vi "test_waypoint-files.vi"() -> ()   [LabVIEW 2019]
panel:
  in  "waypoint files cfg":T1={"Waypoint array"=[{"sel"=TRUE, "inv"=FALSE, "path"=path "C:/AGV/Log/0709/refwpt_0709-1 parking-lot to cafe.txt"}, {"sel"=TRUE, "inv"=TRUE, "path"=path "C:/AGV/Log/0709/refwpt_0709-3 hill to cafe.txt"}, {"sel"=TRUE, "inv"=FALSE, "path"=path "C:/AGV/Log/0709/refwpt_0709-3 hill to cafe.txt"}, {"sel"=TRUE, "inv"=TRUE, "path"=path "C:/AGV/Log/0709/refwpt_0709-1 parking-lot to cafe.txt"}]}
  in  "dt":u32
  out "curr":cluster{cluster{"X":dbl, "Y":dbl}[]}[](graph)
  in  "test run":bool
  in  "Finish":bool
  out "waypoint all":cluster{"XY 그래프":cluster{"X":dbl, "Y":dbl}[]}[](graph)=[{"XY 그래프"=[{"X"=175271.17619236137, "Y"=530128.4758223048}, {"X"=175271.19894111593, "Y"=530128.5113948234}, {"X"=175271.22097384508, "Y"=530128.5456653745}, {"X"=175271.24233997884, "Y"=530128.5782775495}, {"X"=175271.2630835386, "Y"=530128.6094398685}, {"X"=175271.28287635016, "Y"=530128.6390045825}, {"X"=175271.30246842964, "Y"=530128.6674888867}, {"X"=175271.32169791235, "Y"=530128.6949698408}, {"X"=175271.34079370368, "Y"=530128.7218740666}, {"X"=175271.35919639948, "Y"=530128.7486404965}, {"X"=175271.37760654237, "Y"=530128.7749307759}, {"X"=175271.3958476775, "Y"=530128.8006821633}, {"X"=175271.41409588268, "Y"=530128.82612943}, {"X"=175271.43256535105, "Y"=530128.8515127783}, {"X"=175271.45115096163, "Y"=530128.8775306249}, {"X"=175271.47020953769, "Y"=530128.9047301803}, {"X"=175271.48983988236, "Y"=530128.9335728578}, {"X"=175271.51075350813, "Y"=530128.9641342413}, {"X"=175271.5327281118, "Y"=530128.9964238653}, {"X"=175271.5556798252, "Y"=530129.0296384441}, {"X"=175271.57926803536, "Y"=530129.0639199342}, {"X"=175271.60322265813, "Y"=530129.0989961097}, {"X"=175271.62739598114, "Y"=530129.1343413345}, {"X"=175271.65204231316, "Y"=530129.1693854983}, {"X"=175271.67727888995, "Y"=530129.2039340293}, {"X"=175271.7021960715, "Y"=530129.2380118149}, {"X"=175271.7265418914, "Y"=530129.272080192}, {"X"=175271.75024861834, "Y"=530129.3060017383}, {"X"=175271.77407374466, "Y"=530129.3392237227}, {"X"=175271.79764021302, "Y"=530129.3715452666}, {"X"=175271.8208334585, "Y"=530129.4034650351}, {"X"=175271.84318632656, "Y"=530129.4351664272}, {"X"=175271.86533794703, "Y"=530129.4668095922}, {"X"=175271.88783310482, "Y"=530129.4987014595}, {"X"=175271.91096245, "Y"=530129.5317778906}, {"X"=175271.93534531837, "Y"=530129.5660936565}, {"X"=175271.96072388045, "Y"=530129.6019292073}, {"X"=175271.98658903624, "Y"=530129.6387610785}, {"X"=175272.01334256688, "Y"=530129.6755681273}, {"X"=175272.04048386813, "Y"=530129.7120055571}, {"X"=175272.06705517654, "Y"=530129.7482981697}, {"X"=175272.0929584909, "Y"=530129.7842564705}, {"X"=175272.1187534381, "Y"=530129.8198133239}, {"X"=175272.14471871415, "Y"=530129.8539590411}, {"X"=175272.16995301557, "Y"=530129.8877395594}, {"X"=175272.19405677487, "Y"=530129.9217287443}, {"X"=175272.21833020137, "Y"=530129.9549815882}, {"X"=175272.24264042586, "Y"=530129.9874995985}, {"X"=175272.26682258598, "Y"=530130.019843742}, {"X"=175272.29097599763, "Y"=530130.0526518888}, {"X"=175272.3154578647, "Y"=530130.085699904}, {"X"=175272.3404045608, "Y"=530130.1189762856}, {"X"=175272.36576607375, "Y"=530130.1526421116}, {"X"=175272.39173061957, "Y"=530130.1868411056}, {"X"=175272.41826742142, "Y"=530130.2219496026}, {"X"=175272.44515761113, "Y"=530130.2582423848}, {"X"=175272.47299428293, "Y"=530130.2955867319}, {"X"=175272.50161956908, "Y"=530130.333617972}, {"X"=175272.53078700637, "Y"=530130.3725632413}, {"X"=175272.56009692047, "Y"=530130.4117622469}, {"X"=175272.58948861354, "Y"=530130.4507579056}, {"X"=175272.6189694897, "Y"=530130.4887599788}, {"X"=175272.64772876413, "Y"=530130.5265710694}, {"X"=175272.6754292347, "Y"=530130.564287625}, {"X"=175272.70290686525, "Y"=530130.6006341625}, {"X"=175272.73019329942, "Y"=530130.6358292324}, {"X"=175272.75748037494, "Y"=530130.6700431828}, {"X"=175272.78426411733, "Y"=530130.7035893793}, {"X"=175272.8101597084, "Y"=530130.736937318}, {"X"=175272.83573870684, "Y"=530130.7704626593}, {"X"=175272.8619184958, "Y"=530130.8040616941}, {"X"=175272.88838454854, "Y"=530130.8380128188}, {"X"=175272.9151794416, "Y"=530130.8723347735}, {"X"=175272.94225210417, "Y"=530130.9071309266}, {"X"=175272.9695424264, "Y"=530130.941844306}, {"X"=175272.99712724722, "Y"=530130.976398106}, {"X"=175273.02454639255, "Y"=530131.0115406199}, {"X"=175273.05220733272, "Y"=530131.0472728647}, {"X"=175273.0807986791, "Y"=530131.083413007}, {"X"=175273.11001776106, "Y"=530131.12035483}, {"X"=175273.13982529996, "Y"=530131.1576933515}, {"X"=175273.16959295332, "Y"=530131.1950231135}, {"X"=175273.199150427, "Y"=530131.2322702568}, {"X"=175273.22822233994, "Y"=530131.2691692308}, {"X"=175273.25699849764, "Y"=530131.3055019411}, {"X"=175273.28514402997, "Y"=530131.3418553857}, {"X"=175273.31300851193, "Y"=530131.3778234285}, {"X"=175273.34109626192, "Y"=530131.4126099229}, {"X"=175273.36875248022, "Y"=530131.4470458659}, {"X"=175273.39565498653, "Y"=530131.481215453}, {"X"=175273.42227395362, "Y"=530131.5150573613}, {"X"=175273.44885639485, "Y"=530131.5491280085}, {"X"=175273.47631335634, "Y"=530131.5835800796}, {"X"=175273.50455634613, "Y"=530131.6181441419}, {"X"=175273.53303207213, "Y"=530131.6526309372}, {"X"=175273.56118465195, "Y"=530131.6871741797}, {"X"=175273.5885399682, "Y"=530131.7217009136}, {"X"=175273.6153169799, "Y"=530131.7553703267}, {"X"=175273.64185773276, "Y"=530131.7882246927}, {"X"=175273.66779895552, "Y"=530131.8208311108}, {"X"=175273.69422745312, "Y"=530131.8528678423}, {"X"=175273.72143691947, "Y"=530131.8851020389}, {"X"=175273.74863117086, "Y"=530131.9187824245}, {"X"=175273.77588163048, "Y"=530131.9540952493}, {"X"=175273.80346250045, "Y"=530131.9897123085}, {"X"=175273.83148837282, "Y"=530132.0248430432}, {"X"=175273.85959956356, "Y"=530132.0594696489}, {"X"=175273.88716057636, "Y"=530132.0931644908}, {"X"=175273.91324101866, "Y"=530132.1258215536}, {"X"=175273.93725872994, "Y"=530132.1552794413}, {"X"=175273.9610060394, "Y"=530132.1840588958}, {"X"=175273.98491793906, "Y"=530132.2148788949}, {"X"=175274.01010218015, "Y"=530132.247312195}, {"X"=175274.0370394344, "Y"=530132.2812519423}, {"X"=175274.06522422977, "Y"=530132.3159082977}, {"X"=175274.09411559426, "Y"=530132.3504648948}, {"X"=175274.1227654554, "Y"=530132.3851287554}, {"X"=175274.1503264592, "Y"=530132.419419592}, {"X"=175274.17705452998, "Y"=530132.4530147897}, {"X"=175274.20284159074, "Y"=530132.4856116782}, {"X"=175274.2283037938, "Y"=530132.5170863498}, {"X"=175274.25342691143, "Y"=530132.547721861}, {"X"=175274.27838808816, "Y"=530132.5781114623}, {"X"=175274.3033260028, "Y"=530132.6090216575}, {"X"=175274.32839360525, "Y"=530132.6409536466}, {"X"=175274.35449309755, "Y"=530132.6734641539}, {"X"=175274.38062100383, "Y"=530132.7068968687}, {"X"=175274.40689989371, "Y"=530132.7407642006}, {"X"=175274.43333091473, "Y"=530132.7745556141}, {"X"=175274.4600217053, "Y"=530132.807526073}, {"X"=175274.4868586656, "Y"=530132.8399023252}, {"X"=175274.51285591608, "Y"=530132.87228661}, {"X"=175274.5382562742, "Y"=530132.9044162827}, {"X"=175274.5635473854, "Y"=530132.9355474041}, {"X"=175274.5884104021, "Y"=530132.9653934666}, {"X"=175274.61236441362, "Y"=530132.9945796295}, {"X"=175274.63632652618, "Y"=530133.0250077015}, {"X"=175274.66100385884, "Y"=530133.0573637048}, {"X"=175274.68682189335, "Y"=530133.0908495001}, {"X"=175274.71343456453, "Y"=530133.1246625733}, {"X"=175274.7394069741, "Y"=530133.1582322615}, {"X"=175274.76481200277, "Y"=530133.1910433752}, {"X"=175274.78956166538, "Y"=530133.2229962848}, {"X"=175274.8136799043, "Y"=530133.2538012478}, {"X"=175274.83683646756, "Y"=530133.2832084121}, {"X"=175274.85901448457, "Y"=530133.3115041718}, {"X"=175274.88039296027, "Y"=530133.3396114007}, {"X"=175274.90220277346, "Y"=530133.3680036975}, {"X"=175274.92494321318, "Y"=530133.3965796971}, {"X"=175274.94867800857, "Y"=530133.4259230008}, {"X"=175274.97288089248, "Y"=530133.4562959785}, {"X"=175274.99738909313, "Y"=530133.4874727023}, {"X"=175275.02195266922, "Y"=530133.5191031941}, {"X"=175275.04693453235, "Y"=530133.5507990399}, {"X"=175275.07211187517, "Y"=530133.582399972}, {"X"=175275.0973483225, "Y"=530133.6136189348}, {"X"=175275.12214456138, "Y"=530133.6445484182}, {"X"=175275.1461691421, "Y"=530133.6748353543}, {"X"=175275.16997141903, "Y"=530133.7045325036}, {"X"=175275.19344551215, "Y"=530133.7334825781}, {"X"=175275.21657627032, "Y"=530133.7622516518}, {"X"=175275.2396087607, "Y"=530133.791039883}, {"X"=175275.263063832, "Y"=530133.8204461659}, {"X"=175275.28697082214, "Y"=530133.8502073783}, {"X"=175275.3107248371, "Y"=530133.8806593737}, {"X"=175275.33444671123, "Y"=530133.9113245594}, {"X"=175275.35827569605, "Y"=530133.9419672296}, {"X"=175275.38238149675, "Y"=530133.9721618079}, {"X"=175275.40583026237, "Y"=530134.0021319196}, {"X"=175275.42878089705, "Y"=530134.0313976321}, {"X"=175275.451392896, "Y"=530134.0596743522}, {"X"=175275.4738905455, "Y"=530134.0867261271}, {"X"=175275.49585796281, "Y"=530134.113300008}, {"X"=175275.5176917569, "Y"=530134.1402172334}, {"X"=175275.53996690773, "Y"=530134.1678123861}, {"X"=175275.5632661976, "Y"=530134.1963612096}, {"X"=175275.58703968537, "Y"=530134.2259097229}, {"X"=175275.6113424378, "Y"=530134.2565077101}, {"X"=175275.63557628682, "Y"=530134.2880681476}, {"X"=175275.66020323776, "Y"=530134.3195641611}, {"X"=175275.68491628268, "Y"=530134.35081908}, {"X"=175275.7097711018, "Y"=530134.3817905674}, {"X"=175275.73389469017, "Y"=530134.4126088354}, {"X"=175275.7577146616, "Y"=530134.4423003837}, {"X"=175275.78100623479, "Y"=530134.4715351238}, {"X"=175275.80342291066, "Y"=530134.5005604674}, {"X"=175275.82593068006, "Y"=530134.5292381555}, {"X"=175275.84870407218, "Y"=530134.557576552}, {"X"=175275.8723047294, "Y"=530134.5861932964}, {"X"=175275.8962104465, "Y"=530134.6158257698}, {"X"=175275.9206685924, "Y"=530134.6465531515}, {"X"=175275.94534715984, "Y"=530134.6778314793}, {"X"=175275.97041945267, "Y"=530134.7092562574}, {"X"=175275.99540918533, "Y"=530134.7409198968}, {"X"=175276.0208479327, "Y"=530134.7722559111}, {"X"=175276.04626527152, "Y"=530134.8032423825}, {"X"=175276.0707201348, "Y"=530134.8340574529}, {"X"=175276.09469571977, "Y"=530134.8642524196}, {"X"=175276.11845871908, "Y"=530134.8938497994}, {"X"=175276.14216767476, "Y"=530134.9231443482}, {"X"=175276.16565515427, "Y"=530134.9527281164}, {"X"=175276.18933507518, "Y"=530134.9829883279}, {"X"=175276.21328929672, "Y"=530135.0137471656}, {"X"=175276.23786405282, "Y"=530135.0443687653}, {"X"=175276.26216325478, "Y"=530135.07556498}, {"X"=175276.28639760052, "Y"=530135.1066959022}, {"X"=175276.3104839446, "Y"=530135.1375020731}, {"X"=175276.33440064892, "Y"=530135.1675562614}, {"X"=175276.35738667226, "Y"=530135.1965088919}, {"X"=175276.37903969965, "Y"=530135.2246053237}, {"X"=175276.40010305776, "Y"=530135.2524926253}, {"X"=175276.42257118158, "Y"=530135.2821426697}, {"X"=175276.44697916886, "Y"=530135.3138823927}, {"X"=175276.47269765826, "Y"=530135.3469600595}, {"X"=175276.4987057177, "Y"=530135.3812077725}, {"X"=175276.52459011346, "Y"=530135.415572385}, {"X"=175276.54989015873, "Y"=530135.449730072}, {"X"=175276.57483091034, "Y"=530135.4828044904}, {"X"=175276.59904920924, "Y"=530135.5148000421}, {"X"=175276.62270533358, "Y"=530135.5457007147}, {"X"=175276.64582765175, "Y"=530135.5755130845}, {"X"=175276.66823122185, "Y"=530135.6040024065}, {"X"=175276.68969509072, "Y"=530135.6316354779}, {"X"=175276.71066645414, "Y"=530135.6586684603}, {"X"=175276.73236713343, "Y"=530135.6861043859}, {"X"=175276.75435481517, "Y"=530135.7147414407}, {"X"=175276.7766906527, "Y"=530135.7445894321}, {"X"=175276.79958941144, "Y"=530135.7757864564}, {"X"=175276.82353418818, "Y"=530135.8078460784}, {"X"=175276.8479998637, "Y"=530135.8408220143}, {"X"=175276.87281893456, "Y"=530135.874385132}, {"X"=175276.8982353833, "Y"=530135.9077689041}, {"X"=175276.92355676193, "Y"=530135.941353842}, {"X"=175276.94920471654, "Y"=530135.9748434767}, {"X"=175276.97503856523, "Y"=530136.0085911597}, {"X"=175277.00103956382, "Y"=530136.042549222}, {"X"=175277.0271864251, "Y"=530136.0773070601}, {"X"=175277.0538277369, "Y"=530136.1127238036}, {"X"=175277.08122741545, "Y"=530136.1490827955}, {"X"=175277.1097199428, "Y"=530136.1859668468}, {"X"=175277.13826682538, "Y"=530136.2235588295}, {"X"=175277.16623464657, "Y"=530136.2618339786}, {"X"=175277.19366071408, "Y"=530136.3005269243}, {"X"=175277.2211805134, "Y"=530136.3385669983}, {"X"=175277.24894896135, "Y"=530136.3759193327}, {"X"=175277.27651148668, "Y"=530136.4128305535}, {"X"=175277.30377007398, "Y"=530136.4488059506}, {"X"=175277.3310530873, "Y"=530136.4837557664}, {"X"=175277.35790209068, "Y"=530136.5187157434}, {"X"=175277.38489518996, "Y"=530136.5535776294}, {"X"=175277.41163428145, "Y"=530136.5885124052}, {"X"=175277.43827130183, "Y"=530136.6233775625}, {"X"=175277.4651897453, "Y"=530136.6581553189}, {"X"=175277.49179216905, "Y"=530136.6927042685}, {"X"=175277.5176344978, "Y"=530136.727524051}, {"X"=175277.54344339736, "Y"=530136.7624216232}, {"X"=175277.56908157616, "Y"=530136.7971010571}, {"X"=175277.59486848288, "Y"=530136.8314515362}, {"X"=175277.62049959434, "Y"=530136.8667358635}, {"X"=175277.6472220221, "Y"=530136.9020269552}, {"X"=175277.6753270872, "Y"=530136.9375892024}, {"X"=175277.70423989603, "Y"=530136.9740158635}, {"X"=175277.73315492744, "Y"=530137.0114946631}, {"X"=175277.762207521, "Y"=530137.0490629561}, {"X"=175277.79086273597, "Y"=530137.08704529}, {"X"=175277.81920082003, "Y"=530137.1247233516}, {"X"=175277.84718645428, "Y"=530137.1618353155}, {"X"=175277.87464469287, "Y"=530137.1979299895}, {"X"=175277.9008237915, "Y"=530137.2337065866}, {"X"=175277.9271261955, "Y"=530137.2689456482}, {"X"=175277.95360932988, "Y"=530137.3044938259}, {"X"=175277.98064951657, "Y"=530137.3403033918}, {"X"=175278.00823913375, "Y"=530137.376793897}, {"X"=175278.03589400547, "Y"=530137.4140821989}, {"X"=175278.06381256797, "Y"=530137.4518780371}, {"X"=175278.0928952896, "Y"=530137.4894506804}, {"X"=175278.12228673112, "Y"=530137.5271800106}, {"X"=175278.151430175, "Y"=530137.5652175064}, {"X"=175278.180067244, "Y"=530137.6036560485}, {"X"=175278.2089476153, "Y"=530137.6413968799}, {"X"=175278.23784769257, "Y"=530137.67891235}, {"X"=175278.26667870057, "Y"=530137.7167343476}, {"X"=175278.295506967, "Y"=530137.7548282683}, {"X"=175278.3247139495, "Y"=530137.7924860048}, {"X"=175278.35371856295, "Y"=530137.8306049308}, {"X"=175278.38247794105, "Y"=530137.8690675278}, {"X"=175278.41117485458, "Y"=530137.9076745918}, {"X"=175278.43986590861, "Y"=530137.9460974373}, {"X"=175278.46847093437, "Y"=530137.9841853591}, {"X"=175278.49675173132, "Y"=530138.0219634802}, {"X"=175278.52471101953, "Y"=530138.0600522002}, {"X"=175278.55337122487, "Y"=530138.097927977}, {"X"=175278.58284640842, "Y"=530138.1352219965}, {"X"=175278.61280407023, "Y"=530138.1730195764}, {"X"=175278.6421407967, "Y"=530138.212318413}, {"X"=175278.6718176569, "Y"=530138.2519125747}, {"X"=175278.70174630472, "Y"=530138.2918822337}, {"X"=175278.7324047895, "Y"=530138.33213164}, {"X"=175278.76330645662, "Y"=530138.3722427061}, {"X"=175278.7947664709, "Y"=530138.4115552426}, {"X"=175278.82585993598, "Y"=530138.4509254653}, {"X"=175278.85671998298, "Y"=530138.4901432156}, {"X"=175278.88660487908, "Y"=530138.5296956997}, {"X"=175278.91639916634, "Y"=530138.5691607723}, {"X"=175278.9459413744, "Y"=530138.6081526802}, {"X"=175278.97519875658, "Y"=530138.6466803991}, {"X"=175279.00399939533, "Y"=530138.6850196817}, {"X"=175279.0333091102, "Y"=530138.7223730155}, {"X"=175279.06206272755, "Y"=530138.760087587}, {"X"=175279.09082204034, "Y"=530138.7988298717}, {"X"=175279.12034452776, "Y"=530138.8386420244}, {"X"=175279.1511945661, "Y"=530138.8792682199}, {"X"=175279.18281582693, "Y"=530138.9203915691}, {"X"=175279.21403033624, "Y"=530138.9614550801}, {"X"=175279.2443611752, "Y"=530139.0023391879}, {"X"=175279.27433731925, "Y"=530139.0421966133}, {"X"=175279.30379101905, "Y"=530139.0806149871}, {"X"=175279.33186221574, "Y"=530139.1185080461}, {"X"=175279.35892676964, "Y"=530139.1559723445}, {"X"=175279.38686212158, "Y"=530139.1922598379}, {"X"=175279.41540915347, "Y"=530139.2284112311}, {"X"=175279.44399877635, "Y"=530139.2654858995}, {"X"=175279.47229163084, "Y"=530139.3037501057}, {"X"=175279.5011885739, "Y"=530139.3417073153}, {"X"=175279.5302888436, "Y"=530139.3795274108}, {"X"=175279.55929689365, "Y"=530139.4170148209}, {"X"=175279.58712148367, "Y"=530139.4547876343}, {"X"=175279.614104584, "Y"=530139.4922666025}, {"X"=175279.64106285188, "Y"=530139.5288355612}, {"X"=175279.66805218573, "Y"=530139.5639283156}, {"X"=175279.69406272576, "Y"=530139.5987243007}, {"X"=175279.72019882765, "Y"=530139.6337452154}, {"X"=175279.7465857226, "Y"=530139.6700028821}, {"X"=175279.77402264145, "Y"=530139.7072807357}, {"X"=175279.8023412458, "Y"=530139.7461663891}, {"X"=175279.83184920144, "Y"=530139.7864591549}, {"X"=175279.86223487387, "Y"=530139.8276150165}, {"X"=175279.89343681408, "Y"=530139.8689249574}, {"X"=175279.9246664868, "Y"=530139.910027272}, {"X"=175279.95597331063, "Y"=530139.9508596614}, {"X"=175279.98646708307, "Y"=530139.9914291999}, {"X"=175280.0165342933, "Y"=530140.0312308655}, {"X"=175280.0455922527, "Y"=530140.0703207663}, {"X"=175280.07421584064, "Y"=530140.1081000975}, {"X"=175280.10217132277, "Y"=530140.1449069497}, {"X"=175280.1291443291, "Y"=530140.1810696573}, {"X"=175280.15513247682, "Y"=530140.2166825664}, {"X"=175280.18117865722, "Y"=530140.2509501547}, {"X"=175280.206797209, "Y"=530140.2840913909}, {"X"=175280.23235000763, "Y"=530140.3165635753}, {"X"=175280.25719254743, "Y"=530140.350583895}, {"X"=175280.28322486824, "Y"=530140.3861567193}, {"X"=175280.31067604403, "Y"=530140.4234656083}, {"X"=175280.3394714572, "Y"=530140.4627371931}, {"X"=175280.36899300263, "Y"=530140.5034339112}, {"X"=175280.3984291721, "Y"=530140.5446147801}, {"X"=175280.42762195613, "Y"=530140.5855666273}, {"X"=175280.45709143404, "Y"=530140.6248306718}, {"X"=175280.48662985, "Y"=530140.6622443764}, {"X"=175280.51499879934, "Y"=530140.6989856332}, {"X"=175280.54198175855, "Y"=530140.7349207922}, {"X"=175280.56821058405, "Y"=530140.7692488853}, {"X"=175280.5935160324, "Y"=530140.8028483094}, {"X"=175280.61895653373, "Y"=530140.8353896387}, {"X"=175280.64395685605, "Y"=530140.8685493513}, {"X"=175280.66892636206, "Y"=530140.9029710654}, {"X"=175280.69431101237, "Y"=530140.9384925328}, {"X"=175280.72115648974, "Y"=530140.9743659461}, {"X"=175280.74851024564, "Y"=530141.0107827985}, {"X"=175280.77549811464, "Y"=530141.0483794013}, {"X"=175280.80221979975, "Y"=530141.0867248375}, {"X"=175280.83002676512, "Y"=530141.1242324503}, {"X"=175280.85869850015, "Y"=530141.1612214238}, {"X"=175280.88737895148, "Y"=530141.1984623082}, {"X"=175280.9154864763, "Y"=530141.2366638052}, {"X"=175280.94386501168, "Y"=530141.2751508438}, {"X"=175280.97276275096, "Y"=530141.3139804051}, {"X"=175281.00228102322, "Y"=530141.3529734996}, {"X"=175281.03115592728, "Y"=530141.3927687078}, {"X"=175281.0600630094, "Y"=530141.4329611481}, {"X"=175281.08951047983, "Y"=530141.4728734163}, {"X"=175281.1195389884, "Y"=530141.5124709872}, {"X"=175281.1496177038, "Y"=530141.5525733957}, {"X"=175281.1799730451, "Y"=530141.5930623271}, {"X"=175281.20985549872, "Y"=530141.6341930445}, {"X"=175281.24002660922, "Y"=530141.6758856092}, {"X"=175281.2701406386, "Y"=530141.7180455929}, {"X"=175281.30071187392, "Y"=530141.7596526246}, {"X"=175281.3314443854, "Y"=530141.8009806047}, {"X"=175281.36215111212, "Y"=530141.8419768134}, {"X"=175281.39229160105, "Y"=530141.8831999974}, {"X"=175281.42191398598, "Y"=530141.9244513493}, {"X"=175281.4515510467, "Y"=530141.9652731441}, {"X"=175281.48146043535, "Y"=530142.005928764}, {"X"=175281.51131504713, "Y"=530142.0472304844}, {"X"=175281.54193657986, "Y"=530142.088173672}, {"X"=175281.57268864528, "Y"=530142.1289266894}, {"X"=175281.60313783126, "Y"=530142.1699991305}, {"X"=175281.63309546496, "Y"=530142.2110941121}, {"X"=175281.66344358743, "Y"=530142.2512401207}, {"X"=175281.6938036245, "Y"=530142.2909221732}, {"X"=175281.7242871103, "Y"=530142.3298147498}, {"X"=175281.75410497762, "Y"=530142.3688757736}, {"X"=175281.78380300084, "Y"=530142.4081480255}, {"X"=175281.8133516878, "Y"=530142.4481421259}, {"X"=175281.843129746, "Y"=530142.4887193365}, {"X"=175281.87290404478, "Y"=530142.530421954}, {"X"=175281.9035498242, "Y"=530142.5720776024}, {"X"=175281.93428441955, "Y"=530142.6138128963}, {"X"=175281.96503678558, "Y"=530142.6558666679}, {"X"=175281.9955543286, "Y"=530142.697891169}, {"X"=175282.02619666213, "Y"=530142.7392804611}, {"X"=175282.05613426614, "Y"=530142.7804920393}, {"X"=175282.085671532, "Y"=530142.8211187952}, {"X"=175282.11518036062, "Y"=530142.8620131105}, {"X"=175282.1456811949, "Y"=530142.9028811874}, {"X"=175282.1771792938, "Y"=530142.9437019224}, {"X"=175282.20884129676, "Y"=530142.9851325951}, {"X"=175282.2397414916, "Y"=530143.0274545162}, {"X"=175282.27097983484, "Y"=530143.0694003062}, {"X"=175282.30222752306, "Y"=530143.1112106664}, {"X"=175282.33341880344, "Y"=530143.1525184269}, {"X"=175282.36387121098, "Y"=530143.1931857627}, {"X"=175282.39415697358, "Y"=530143.2332143132}, {"X"=175282.42362074467, "Y"=530143.273250842}, {"X"=175282.4527898988, "Y"=530143.313107335}, {"X"=175282.48128543983, "Y"=530143.3534241924}, {"X"=175282.51088211057, "Y"=530143.3931717661}, {"X"=175282.54090583324, "Y"=530143.4323542686}, {"X"=175282.5705854428, "Y"=530143.471693168}, {"X"=175282.59956877265, "Y"=530143.5110152598}, {"X"=175282.6287490361, "Y"=530143.5495365605}, {"X"=175282.6578151003, "Y"=530143.588080396}, {"X"=175282.68706937856, "Y"=530143.626769067}, {"X"=175282.7166015784, "Y"=530143.6659829883}, {"X"=175282.7467854581, "Y"=530143.7057077412}, {"X"=175282.7773134472, "Y"=530143.7458743079}, {"X"=175282.80814411398, "Y"=530143.7859523029}, {"X"=175282.838184342, "Y"=530143.826524301}, {"X"=175282.8683331907, "Y"=530143.8669838827}, {"X"=175282.89893667438, "Y"=530143.906620824}, {"X"=175282.9292553414, "Y"=530143.9460954601}, {"X"=175282.95864972533, "Y"=530143.9860345288}, {"X"=175282.98848236992, "Y"=530144.0253041666}, {"X"=175283.0181754902, "Y"=530144.0647196089}, {"X"=175283.04813967334, "Y"=530144.1041386905}, {"X"=175283.0777535639, "Y"=530144.1434200734}, {"X"=175283.10767498845, "Y"=530144.1824585982}, {"X"=175283.13729311575, "Y"=530144.2216767089}, {"X"=175283.16682575422, "Y"=530144.2604411386}, {"X"=175283.19558793583, "Y"=530144.298968117}, {"X"=175283.2241672666, "Y"=530144.3373668897}, {"X"=175283.25312463212, "Y"=530144.3756990653}, {"X"=175283.2826412646, "Y"=530144.4144435665}, {"X"=175283.31204253566, "Y"=530144.4543149145}, {"X"=175283.3421730828, "Y"=530144.4945792174}, {"X"=175283.3722977522, "Y"=530144.5352508556}, {"X"=175283.40277253534, "Y"=530144.5759991499}, {"X"=175283.4329718328, "Y"=530144.6164463753}, {"X"=175283.46352714679, "Y"=530144.6565706909}, {"X"=175283.49419215746, "Y"=530144.6963472951}, {"X"=175283.52462383907, "Y"=530144.7353998523}, {"X"=175283.55396090678, "Y"=530144.7748296679}, {"X"=175283.5835840078, "Y"=530144.8145316618}, {"X"=175283.61356165347, "Y"=530144.8549118419}, {"X"=175283.64420085354, "Y"=530144.8958449971}, {"X"=175283.6745753304, "Y"=530144.9374226541}, {"X"=175283.7054805737, "Y"=530144.9784593498}, {"X"=175283.73611770716, "Y"=530145.0195933951}, {"X"=175283.76646929348, "Y"=530145.060618409}, {"X"=175283.79638575143, "Y"=530145.1009754644}, {"X"=175283.82613484285, "Y"=530145.1407492278}, {"X"=175283.85577592644, "Y"=530145.1808429519}, {"X"=175283.885663239, "Y"=530145.2218282747}, {"X"=175283.91601352586, "Y"=530145.2642128682}, {"X"=175283.947973915, "Y"=530145.3071054613}, {"X"=175283.98073738883, "Y"=530145.3501865757}, {"X"=175284.0130592979, "Y"=530145.3937184858}, {"X"=175284.04495574543, "Y"=530145.4371550977}, {"X"=175284.07744431793, "Y"=530145.4792348221}, {"X"=175284.10977979988, "Y"=530145.5207656174}, {"X"=175284.14209092426, "Y"=530145.5618481026}, {"X"=175284.1734844176, "Y"=530145.6035470525}, {"X"=175284.20526964756, "Y"=530145.64591853}, {"X"=175284.23726074316, "Y"=530145.6887122538}, {"X"=175284.26911709429, "Y"=530145.7317705223}, {"X"=175284.3002081578, "Y"=530145.7757400281}, {"X"=175284.3324970653, "Y"=530145.8188969061}, {"X"=175284.3652071701, "Y"=530145.861604157}, {"X"=175284.39764851984, "Y"=530145.9041912265}, {"X"=175284.42918119673, "Y"=530145.9465290459}, {"X"=175284.46056710478, "Y"=530145.9883589816}, {"X"=175284.49216892465, "Y"=530146.0298153689}, {"X"=175284.52417019266, "Y"=530146.0712561457}, {"X"=175284.55620185586, "Y"=530146.1139909273}, {"X"=175284.58914297097, "Y"=530146.1578373206}, {"X"=175284.62234006467, "Y"=530146.2022778434}, {"X"=175284.65546114062, "Y"=530146.246771863}, {"X"=175284.6880941868, "Y"=530146.290381658}, {"X"=175284.7208188328, "Y"=530146.3323175148}, {"X"=175284.75239886277, "Y"=530146.3738938312}, {"X"=175284.7831501817, "Y"=530146.4147045729}, {"X"=175284.8133402377, "Y"=530146.4547267567}, {"X"=175284.84401715046, "Y"=530146.4940394099}, {"X"=175284.87397091367, "Y"=530146.5335351082}, {"X"=175284.9036312302, "Y"=530146.5732458769}, {"X"=175284.93309855444, "Y"=530146.613594275}, {"X"=175284.96356257205, "Y"=530146.6534025557}, {"X"=175284.99386236374, "Y"=530146.6933911182}, {"X"=175285.02346019607, "Y"=530146.7338401279}, {"X"=175285.05236272336, "Y"=530146.7740026298}, {"X"=175285.08160787256, "Y"=530146.8135059732}, {"X"=175285.11075855847, "Y"=530146.8522171556}, {"X"=175285.1397029091, "Y"=530146.8900477202}, {"X"=175285.16758823174, "Y"=530146.9277071673}, {"X"=175285.1958097519, "Y"=530146.9649305547}, {"X"=175285.22430324028, "Y"=530147.0021642376}, {"X"=175285.25292049572, "Y"=530147.0399147498}, {"X"=175285.2813211958, "Y"=530147.0781209449}, {"X"=175285.31057523662, "Y"=530147.1161381598}, {"X"=175285.34005196817, "Y"=530147.1539760306}, {"X"=175285.36896240644, "Y"=530147.1923216721}, {"X"=175285.39717128137, "Y"=530147.2306616167}, {"X"=175285.42578933577, "Y"=530147.2680836085}, {"X"=175285.45344861108, "Y"=530147.3059856722}, {"X"=175285.48089067373, "Y"=530147.3438228995}, {"X"=175285.5080579749, "Y"=530147.3816032234}, {"X"=175285.5362745623, "Y"=530147.4192572538}, {"X"=175285.56450088962, "Y"=530147.457507248}, {"X"=175285.59262162892, "Y"=530147.4962980582}, {"X"=175285.62062185156, "Y"=530147.535671899}, {"X"=175285.64955586256, "Y"=530147.5747999209}, {"X"=175285.67873101955, "Y"=530147.6137008192}, {"X"=175285.70778441665, "Y"=530147.6521647931}, {"X"=175285.73595734, "Y"=530147.6906291493}, {"X"=175285.76424656826, "Y"=530147.7282851851}, {"X"=175285.79254815428, "Y"=530147.7653274323}, {"X"=175285.82039661068, "Y"=530147.8022034307}, {"X"=175285.8475120278, "Y"=530147.8389140045}, {"X"=175285.87503700587, "Y"=530147.8754358034}, {"X"=175285.90290258938, "Y"=530147.9124127475}, {"X"=175285.9312492372, "Y"=530147.9503150036}, {"X"=175285.96021217544, "Y"=530147.9893430532}, {"X"=175285.99025259638, "Y"=530148.0293912095}, {"X"=175286.020547502, "Y"=530148.0707260491}, {"X"=175286.0507198295, "Y"=530148.1125473701}, {"X"=175286.0801991385, "Y"=530148.1548557479}, {"X"=175286.11029842027, "Y"=530148.1962377818}, {"X"=175286.140521968, "Y"=530148.236507368}, {"X"=175286.1702336265, "Y"=530148.2765109926}, {"X"=175286.19897639108, "Y"=530148.3165685348}, {"X"=175286.22822459688, "Y"=530148.3559109423}, {"X"=175286.25734444545, "Y"=530148.3955811377}, {"X"=175286.28666392548, "Y"=530148.4356613915}, {"X"=175286.31565993704, "Y"=530148.4762897632}, {"X"=175286.3452906467, "Y"=530148.5167775253}, {"X"=175286.37519197192, "Y"=530148.5571168768}, {"X"=175286.4050008174, "Y"=530148.5970369751}, {"X"=175286.43396749627, "Y"=530148.6376310271}, {"X"=175286.46322490054, "Y"=530148.6782874814}, {"X"=175286.492849835, "Y"=530148.7186198815}, {"X"=175286.52249772992, "Y"=530148.7589289073}, {"X"=175286.55175465223, "Y"=530148.7991236621}, {"X"=175286.58125565466, "Y"=530148.8385840784}, {"X"=175286.61029576242, "Y"=530148.8779481912}, {"X"=175286.63886234077, "Y"=530148.9171383454}, {"X"=175286.6662366717, "Y"=530148.9560379102}, {"X"=175286.69313776202, "Y"=530148.994561523}, {"X"=175286.71988594692, "Y"=530149.0322998049}, {"X"=175286.74621013305, "Y"=530149.0686387003}, {"X"=175286.77196082624, "Y"=530149.105147988}, {"X"=175286.79863885418, "Y"=530149.142826546}, {"X"=175286.826449198, "Y"=530149.1826948401}, {"X"=175286.85571812605, "Y"=530149.22455435}, {"X"=175286.8856057402, "Y"=530149.2680490734}, {"X"=175286.9166891728, "Y"=530149.3112439304}, {"X"=175286.94756222956, "Y"=530149.3539899159}, {"X"=175286.97788231372, "Y"=530149.3960549736}, {"X"=175287.0072642036, "Y"=530149.4374746449}, {"X"=175287.036659181, "Y"=530149.4776268187}, {"X"=175287.06515292102, "Y"=530149.5170491512}, {"X"=175287.09290277224, "Y"=530149.5556312968}, {"X"=175287.119605925, "Y"=530149.5949179686}, {"X"=175287.14739103278, "Y"=530149.6343412843}, {"X"=175287.17584614863, "Y"=530149.6735817129}, {"X"=175287.2043462658, "Y"=530149.713065068}, {"X"=175287.23238548372, "Y"=530149.7533488837}, {"X"=175287.2611683341, "Y"=530149.7940866544}, {"X"=175287.29022015305, "Y"=530149.8350178539}, {"X"=175287.31949523537, "Y"=530149.8762647061}, {"X"=175287.3483993774, "Y"=530149.9178800166}, {"X"=175287.37800341408, "Y"=530149.9598373151}, {"X"=175287.40788540026, "Y"=530150.0026284064}, {"X"=175287.43796715222, "Y"=530150.0458750587}, {"X"=175287.46768028973, "Y"=530150.0890806267}, {"X"=175287.4980408877, "Y"=530150.131969081}, {"X"=175287.52849568735, "Y"=530150.1743611491}, {"X"=175287.55858161338, "Y"=530150.2166244559}, {"X"=175287.587891292, "Y"=530150.2584882879}, {"X"=175287.61718485222, "Y"=530150.299393249}, {"X"=175287.6459290996, "Y"=530150.3402576577}, {"X"=175287.6745216954, "Y"=530150.3816607958}, {"X"=175287.70312189191, "Y"=530150.4232381617}, {"X"=175287.73260160128, "Y"=530150.4650881741}, {"X"=175287.76249647667, "Y"=530150.5074463824}, {"X"=175287.79194968793, "Y"=530150.5502209846}, {"X"=175287.82063771554, "Y"=530150.5936437859}, {"X"=175287.85010417973, "Y"=530150.6364072509}, {"X"=175287.8799999824, "Y"=530150.6784802239}, {"X"=175287.90960605638, "Y"=530150.7208281889}, {"X"=175287.93873272298, "Y"=530150.7643085173}, {"X"=175287.96876992864, "Y"=530150.8083710499}, {"X"=175287.99941347007, "Y"=530150.8537847098}, {"X"=175288.03114061506, "Y"=530150.8995947163}, {"X"=175288.06276278125, "Y"=530150.9458489771}, {"X"=175288.09491236706, "Y"=530150.9922304217}, {"X"=175288.12711197292, "Y"=530151.0378525751}, {"X"=175288.15885105054, "Y"=530151.0829045124}, {"X"=175288.18957201828, "Y"=530151.1275432631}, {"X"=175288.22029953293, "Y"=530151.1716992052}, {"X"=175288.25093068994, "Y"=530151.2162216855}, {"X"=175288.28194385857, "Y"=530151.2608229464}, {"X"=175288.31247756336, "Y"=530151.3053401643}, {"X"=175288.3432649797, "Y"=530151.3499842685}, {"X"=175288.37381855643, "Y"=530151.3946312824}, {"X"=175288.40417486875, "Y"=530151.4390691165}, {"X"=175288.43387214167, "Y"=530151.4838041204}, {"X"=175288.4640216559, "Y"=530151.5281038334}, {"X"=175288.49419391077, "Y"=530151.5723058113}, {"X"=175288.52442907562, "Y"=530151.6168139238}, {"X"=175288.5542325439, "Y"=530151.6615153196}, {"X"=175288.58497125428, "Y"=530151.7061640078}, {"X"=175288.6160333851, "Y"=530151.7508494728}, {"X"=175288.6471765447, "Y"=530151.7953782111}, {"X"=175288.67735389853, "Y"=530151.8404070201}, {"X"=175288.7079524178, "Y"=530151.8849762128}, {"X"=175288.73890247892, "Y"=530151.928907307}, {"X"=175288.76994925848, "Y"=530151.9731943812}, {"X"=175288.80061505685, "Y"=530152.0180497186}, {"X"=175288.8317122577, "Y"=530152.0632134323}, {"X"=175288.86321392213, "Y"=530152.1088598475}, {"X"=175288.89513094307, "Y"=530152.1541798481}, {"X"=175288.92626476596, "Y"=530152.1997463321}, {"X"=175288.95799837503, "Y"=530152.2447483455}, {"X"=175288.98898292525, "Y"=530152.2889612439}, {"X"=175289.01901433212, "Y"=530152.3328628676}, {"X"=175289.04869555627, "Y"=530152.376364868}, {"X"=175289.07902414582, "Y"=530152.419217908}, {"X"=175289.10912839917, "Y"=530152.4628917961}, {"X"=175289.13898367598, "Y"=530152.50744099}, {"X"=175289.16920329822, "Y"=530152.5520878835}, {"X"=175289.200499284, "Y"=530152.5967771014}, {"X"=175289.23222510127, "Y"=530152.6409434144}, {"X"=175289.26360565764, "Y"=530152.6851751207}, {"X"=175289.29417483156, "Y"=530152.7294092241}, {"X"=175289.32498934455, "Y"=530152.7727347375}, {"X"=175289.35533826269, "Y"=530152.8164722754}, {"X"=175289.385890799, "Y"=530152.8604711375}, {"X"=175289.41661120942, "Y"=530152.904625996}, {"X"=175289.4478910891, "Y"=530152.9495616502}, {"X"=175289.47917020373, "Y"=530152.9951376967}, {"X"=175289.5106185431, "Y"=530153.0407265619}, {"X"=175289.54200313758, "Y"=530153.08602594}, {"X"=175289.5739645148, "Y"=530153.130472353}, {"X"=175289.60522496788, "Y"=530153.1748287205}, {"X"=175289.6366590831, "Y"=530153.2192023303}, {"X"=175289.6678968938, "Y"=530153.2639904988}, {"X"=175289.69931618578, "Y"=530153.3099423731}, {"X"=175289.73108270628, "Y"=530153.3561928844}, {"X"=175289.76287250203, "Y"=530153.402526566}, {"X"=175289.7944634813, "Y"=530153.4493247548}, {"X"=175289.82722049116, "Y"=530153.4953348278}, {"X"=175289.8601326513, "Y"=530153.5407928433}, {"X"=175289.89234136775, "Y"=530153.5862074348}, {"X"=175289.9231350958, "Y"=530153.6320945667}, {"X"=175289.95472487184, "Y"=530153.6784854437}, {"X"=175289.98763897427, "Y"=530153.7249001521}, {"X"=175290.0213877559, "Y"=530153.7711048503}, {"X"=175290.05441688612, "Y"=530153.8180774795}, {"X"=175290.0870279125, "Y"=530153.865045794}, {"X"=175290.1190894426, "Y"=530153.9119114052}, {"X"=175290.15082290868, "Y"=530153.9583695601}, {"X"=175290.18253651966, "Y"=530154.004402696}, {"X"=175290.215824471, "Y"=530154.0499339624}, {"X"=175290.24876343764, "Y"=530154.0957714727}, {"X"=175290.28090772417, "Y"=530154.1421662602}, {"X"=175290.31260737777, "Y"=530154.1888720124}, {"X"=175290.34510314872, "Y"=530154.2349083878}, {"X"=175290.37745346018, "Y"=530154.2805800489}, {"X"=175290.40967781737, "Y"=530154.3255950455}, {"X"=175290.4415173953, "Y"=530154.3698930992}, {"X"=175290.47334424395, "Y"=530154.4146795312}, {"X"=175290.50540644318, "Y"=530154.4602743543}, {"X"=175290.5380738031, "Y"=530154.5068251977}, {"X"=175290.57155401353, "Y"=530154.5544701797}, {"X"=175290.60687618723, "Y"=530154.6022528902}, {"X"=175290.64227715097, "Y"=530154.6503194917}, {"X"=175290.6771000642, "Y"=530154.6985121064}, {"X"=175290.71074572636, "Y"=530154.7463930005}, {"X"=175290.74366782108, "Y"=530154.7937166628}, {"X"=175290.77674741115, "Y"=530154.8397823889}, {"X"=175290.8104922183, "Y"=530154.8852446075}, {"X"=175290.84345047412, "Y"=530154.9319166768}, {"X"=175290.8771305831, "Y"=530154.9791648488}, {"X"=175290.91168912026, "Y"=530155.0269198505}, {"X"=175290.94661003543, "Y"=530155.0750045214}, {"X"=175290.981122192, "Y"=530155.1229516666}, {"X"=175291.01579159318, "Y"=530155.1701547412}, {"X"=175291.04955919375, "Y"=530155.2164370784}, {"X"=175291.08231414267, "Y"=530155.262653598}, {"X"=175291.11492730505, "Y"=530155.3085508951}, {"X"=175291.14872001382, "Y"=530155.3537377286}, {"X"=175291.182644366, "Y"=530155.3991095183}, {"X"=175291.21636701853, "Y"=530155.4442699214}, {"X"=175291.24936465317, "Y"=530155.4895811882}, {"X"=175291.28248111415, "Y"=530155.5349365}, {"X"=175291.31537208255, "Y"=530155.580122668}, {"X"=175291.348325878, "Y"=530155.6252864538}, {"X"=175291.38153227052, "Y"=530155.6705005467}, {"X"=175291.41516056712, "Y"=530155.7158055122}, {"X"=175291.44858402072, "Y"=530155.7616338248}, {"X"=175291.48274548614, "Y"=530155.8069127973}, {"X"=175291.51713847913, "Y"=530155.8517049672}, {"X"=175291.55134679007, "Y"=530155.8960504106}, {"X"=175291.58456519523, "Y"=530155.9396351947}, {"X"=175291.61696642355, "Y"=530155.9821591497}, {"X"=175291.6479902135, "Y"=530156.023771541}, {"X"=175291.6785537982, "Y"=530156.0649235916}, {"X"=175291.70969666803, "Y"=530156.1063669323}, {"X"=175291.7420121854, "Y"=530156.1480631868}, {"X"=175291.77421945485, "Y"=530156.1905977037}, {"X"=175291.80641845273, "Y"=530156.2342298953}, {"X"=175291.83880961206, "Y"=530156.2778426528}, {"X"=175291.8714862793, "Y"=530156.3212525729}, {"X"=175291.903615614, "Y"=530156.3652911794}, {"X"=175291.9363788722, "Y"=530156.4089272545}, {"X"=175291.9693198524, "Y"=530156.4530544727}, {"X"=175292.00263982284, "Y"=530156.4980373809}, {"X"=175292.03573972572, "Y"=530156.5440875158}, {"X"=175292.06968311957, "Y"=530156.5908099515}, {"X"=175292.10416577995, "Y"=530156.6374730819}, {"X"=175292.13854745447, "Y"=530156.6838335177}, {"X"=175292.1720661163, "Y"=530156.7301088271}, {"X"=175292.2050774269, "Y"=530156.7758551223}, {"X"=175292.23774666685, "Y"=530156.8212483841}, {"X"=175292.2703950841, "Y"=530156.8658914415}, {"X"=175292.30284617713, "Y"=530156.9103042324}, {"X"=175292.33573019976, "Y"=530156.9552418168}, {"X"=175292.3690841089, "Y"=530157.0006197365}, {"X"=175292.40287209605, "Y"=530157.0463115734}, {"X"=175292.43625491866, "Y"=530157.0924818472}, {"X"=175292.46991898818, "Y"=530157.1379065764}, {"X"=175292.50292587615, "Y"=530157.1830557807}, {"X"=175292.53606117488, "Y"=530157.2272967426}, {"X"=175292.56777705185, "Y"=530157.2717072674}, {"X"=175292.59928240773, "Y"=530157.317118397}, {"X"=175292.63191829307, "Y"=530157.3626160842}, {"X"=175292.66587593383, "Y"=530157.4075682566}, {"X"=175292.69985293486, "Y"=530157.4527767475}, {"X"=175292.73331970134, "Y"=530157.49827975}, {"X"=175292.76675738787, "Y"=530157.5444332153}, {"X"=175292.8009040642, "Y"=530157.5910063332}, {"X"=175292.8354354053, "Y"=530157.637958995}, {"X"=175292.87064782495, "Y"=530157.6854778919}, {"X"=175292.90666329346, "Y"=530157.7325748918}, {"X"=175292.94218916725, "Y"=530157.7803559012}, {"X"=175292.97651543948, "Y"=530157.8283546561}, {"X"=175293.01087843996, "Y"=530157.8758927135}, {"X"=175293.04497236086, "Y"=530157.9235003758}, {"X"=175293.07881658027, "Y"=530157.9705383087}, {"X"=175293.11260566092, "Y"=530158.0172023829}, {"X"=175293.14703717566, "Y"=530158.0636470264}, {"X"=175293.1813700373, "Y"=530158.1105791891}, {"X"=175293.21539555187, "Y"=530158.1584179054}, {"X"=175293.2495375595, "Y"=530158.205812335}, {"X"=175293.28470608912, "Y"=530158.252269229}, {"X"=175293.3199063943, "Y"=530158.2983886322}, {"X"=175293.35488698122, "Y"=530158.3438949328}, {"X"=175293.3886446154, "Y"=530158.389809945}, {"X"=175293.4223983855, "Y"=530158.4359169754}, {"X"=175293.45635716093, "Y"=530158.4824551338}, {"X"=175293.49104767398, "Y"=530158.5290177691}, {"X"=175293.52591940033, "Y"=530158.5751547926}, {"X"=175293.56061870293, "Y"=530158.6210958796}, {"X"=175293.59411550115, "Y"=530158.6668718222}, {"X"=175293.6271809516, "Y"=530158.7120597042}, {"X"=175293.65945930034, "Y"=530158.7576716585}, {"X"=175293.69267942, "Y"=530158.8030433188}, {"X"=175293.72706808845, "Y"=530158.8484792291}, {"X"=175293.76185547217, "Y"=530158.895451116}, {"X"=175293.7965144529, "Y"=530158.9433356876}, {"X"=175293.83203452808, "Y"=530158.9915551107}, {"X"=175293.86796527763, "Y"=530159.0399619979}, {"X"=175293.90361325, "Y"=530159.0885983519}, {"X"=175293.93887625565, "Y"=530159.1373534874}, {"X"=175293.97487363513, "Y"=530159.1852274456}, {"X"=175294.01073365632, "Y"=530159.2333814944}, {"X"=175294.04643691002, "Y"=530159.2821408798}, {"X"=175294.0818756446, "Y"=530159.3307123703}, {"X"=175294.11788264144, "Y"=530159.3791445598}, {"X"=175294.15405635608, "Y"=530159.4270401951}, {"X"=175294.19031250803, "Y"=530159.474657012}, {"X"=175294.2255617339, "Y"=530159.5217474012}, {"X"=175294.25969315338, "Y"=530159.5685591893}, {"X"=175294.29275883175, "Y"=530159.6156260639}, {"X"=175294.32651326683, "Y"=530159.6616609548}, {"X"=175294.3607518941, "Y"=530159.7075834295}, {"X"=175294.3953102612, "Y"=530159.754094294}, {"X"=175294.4301660572, "Y"=530159.800839571}, {"X"=175294.46538930168, "Y"=530159.8478312608}, {"X"=175294.5005892464, "Y"=530159.8944334593}, {"X"=175294.5360717114, "Y"=530159.9401191891}, {"X"=175294.57088286872, "Y"=530159.9855471951}, {"X"=175294.60512637242, "Y"=530160.0307227217}, {"X"=175294.63868134032, "Y"=530160.0764041571}, {"X"=175294.67373468378, "Y"=530160.1216560913}, {"X"=175294.7093190078, "Y"=530160.167040749}, {"X"=175294.74458629126, "Y"=530160.2136494077}, {"X"=175294.7794420138, "Y"=530160.2609707027}, {"X"=175294.81483305173, "Y"=530160.3092915086}, {"X"=175294.85090509735, "Y"=530160.3593561125}, {"X"=175294.88806120938, "Y"=530160.4102709948}, {"X"=175294.92585483048, "Y"=530160.4622982909}, {"X"=175294.96463635506, "Y"=530160.5147089018}, {"X"=175295.00314084318, "Y"=530160.5674932406}, {"X"=175295.04201721685, "Y"=530160.6190278914}, {"X"=175295.08002002342, "Y"=530160.6696039869}, {"X"=175295.1164572531, "Y"=530160.7191503169}, {"X"=175295.15120238528, "Y"=530160.7677160925}, {"X"=175295.18513989958, "Y"=530160.8154596288}, {"X"=175295.21911985, "Y"=530160.8622751979}, {"X"=175295.25361585215, "Y"=530160.908367834}, {"X"=175295.2882631498, "Y"=530160.9541026478}, {"X"=175295.3227068247, "Y"=530160.9995739195}, {"X"=175295.35650395526, "Y"=530161.0453733961}, {"X"=175295.39054459677, "Y"=530161.090246534}, {"X"=175295.4242712038, "Y"=530161.1346622286}, {"X"=175295.45741238436, "Y"=530161.1797045011}, {"X"=175295.49052893237, "Y"=530161.2251053321}, {"X"=175295.52422381577, "Y"=530161.2716753556}, {"X"=175295.5584969615, "Y"=530161.3190916035}, {"X"=175295.59356381797, "Y"=530161.3671225884}, {"X"=175295.62898613833, "Y"=530161.4158406355}, {"X"=175295.66490363725, "Y"=530161.4645672088}, {"X"=175295.70087106727, "Y"=530161.5140039441}, {"X"=175295.7368334574, "Y"=530161.563833585}, {"X"=175295.77286787695, "Y"=530161.6140581218}, {"X"=175295.80940447663, "Y"=530161.6645608615}, {"X"=175295.84631290415, "Y"=530161.7143954771}, {"X"=175295.88293148752, "Y"=530161.7641654665}, {"X"=175295.91866648968, "Y"=530161.8137837979}, {"X"=175295.95399056026, "Y"=530161.862829545}, {"X"=175295.9882959008, "Y"=530161.9112501208}, {"X"=175296.021704602, "Y"=530161.9589974427}, {"X"=175296.05467506434, "Y"=530162.0062210971}, {"X"=175296.08883693878, "Y"=530162.0522559017}, {"X"=175296.12335942886, "Y"=530162.0980232735}, {"X"=175296.15767913012, "Y"=530162.1438101135}, {"X"=175296.19184323237, "Y"=530162.18969841}, {"X"=175296.22616491732, "Y"=530162.2364574812}, {"X"=175296.26090724123, "Y"=530162.2837780067}, {"X"=175296.29650390253, "Y"=530162.3312458408}, {"X"=175296.33225156722, "Y"=530162.3800550482}, {"X"=175296.36839006183, "Y"=530162.4298308986}, {"X"=175296.40405752033, "Y"=530162.4808744899}, {"X"=175296.4404195736, "Y"=530162.5316652008}, {"X"=175296.4771856306, "Y"=530162.5818831403}, {"X"=175296.5143190418, "Y"=530162.6314185419}, {"X"=175296.55121999886, "Y"=530162.6796261277}, {"X"=175296.58696759774, "Y"=530162.7272156009}, {"X"=175296.62106253332, "Y"=530162.7745791067}, {"X"=175296.65513370547, "Y"=530162.8216951848}, {"X"=175296.6894842066, "Y"=530162.8689147633}, {"X"=175296.7245051825, "Y"=530162.9161112749}, {"X"=175296.7594826378, "Y"=530162.9641680548}, {"X"=175296.7949428259, "Y"=530163.0125164114}, {"X"=175296.83066872833, "Y"=530163.0611569866}, {"X"=175296.8668875833, "Y"=530163.1102511483}, {"X"=175296.90347265196, "Y"=530163.1594751914}, {"X"=175296.94033878695, "Y"=530163.2096906174}, {"X"=175296.97742890092, "Y"=530163.2601628694}, {"X"=175297.0145870955, "Y"=530163.3102930847}, {"X"=175297.0517672564, "Y"=530163.3603633035}, {"X"=175297.0892145761, "Y"=530163.4100154234}, {"X"=175297.1260384531, "Y"=530163.4594196689}, {"X"=175297.16179432158, "Y"=530163.5083098755}, {"X"=175297.1968335202, "Y"=530163.5568792308}, {"X"=175297.2321241116, "Y"=530163.6047908057}, {"X"=175297.26783519427, "Y"=530163.6517155846}, {"X"=175297.3031716078, "Y"=530163.6989466816}, {"X"=175297.3376430369, "Y"=530163.7460238435}, {"X"=175297.37241788793, "Y"=530163.7935651409}, {"X"=175297.40764496886, "Y"=530163.8421672372}, {"X"=175297.44412403886, "Y"=530163.8908943782}, {"X"=175297.4814756149, "Y"=530163.9405212577}, {"X"=175297.51936847973, "Y"=530163.9910710508}, {"X"=175297.5573672983, "Y"=530164.0433064074}, {"X"=175297.595877763, "Y"=530164.0960252604}, {"X"=175297.63482324645, "Y"=530164.1484764633}, {"X"=175297.67408375622, "Y"=530164.201420622}, {"X"=175297.71312810254, "Y"=530164.2540568792}, {"X"=175297.7516670672, "Y"=530164.3059288258}, {"X"=175297.78913671337, "Y"=530164.3565442422}, {"X"=175297.82573620637, "Y"=530164.4067560205}, {"X"=175297.8615577048, "Y"=530164.4559778853}, {"X"=175297.8972371134, "Y"=530164.5047762007}, {"X"=175297.93302551022, "Y"=530164.553887177}, {"X"=175297.96961301554, "Y"=530164.6033398478}, {"X"=175298.00658313325, "Y"=530164.653376285}, {"X"=175298.04413234367, "Y"=530164.7030403184}, {"X"=175298.08174063195, "Y"=530164.7529128302}, {"X"=175298.11949670635, "Y"=530164.8033376161}, {"X"=175298.15754264174, "Y"=530164.8535340244}, {"X"=175298.19573262517, "Y"=530164.9039153553}, {"X"=175298.2333517534, "Y"=530164.9547600736}, {"X"=175298.2709253971, "Y"=530165.0063984748}, {"X"=175298.30921058325, "Y"=530165.0575242384}, {"X"=175298.34725989297, "Y"=530165.108563021}, {"X"=175298.3849848592, "Y"=530165.160152141}, {"X"=175298.42313040857, "Y"=530165.2113859762}, {"X"=175298.46161175598, "Y"=530165.2629473361}, {"X"=175298.5006422235, "Y"=530165.3141863251}, {"X"=175298.53957860355, "Y"=530165.3662590976}, {"X"=175298.57924604914, "Y"=530165.4196282434}, {"X"=175298.61979824462, "Y"=530165.4744453614}, {"X"=175298.66179051698, "Y"=530165.5306877274}, {"X"=175298.70499840498, "Y"=530165.5885357952}, {"X"=175298.74955290352, "Y"=530165.6482533285}, {"X"=175298.79480152024, "Y"=530165.7087545921}, {"X"=175298.83997422215, "Y"=530165.7702460737}, {"X"=175298.8847225618, "Y"=530165.8314136203}, {"X"=175298.9291021474, "Y"=530165.8912926009}, {"X"=175298.97281817885, "Y"=530165.9496397171}, {"X"=175299.01543963805, "Y"=530166.0068768775}, {"X"=175299.05688362545, "Y"=530166.0634271845}, {"X"=175299.09825262203, "Y"=530166.1191808339}, {"X"=175299.13975714424, "Y"=530166.173434664}, {"X"=175299.18070865513, "Y"=530166.2269953544}, {"X"=175299.22062828136, "Y"=530166.2793770946}, {"X"=175299.25974002617, "Y"=530166.3308455878}, {"X"=175299.297952328, "Y"=530166.3812912287}, {"X"=175299.33612488734, "Y"=530166.4305771838}, {"X"=175299.37402761978, "Y"=530166.4784788326}, {"X"=175299.41189246927, "Y"=530166.5255504185}, {"X"=175299.44854593184, "Y"=530166.5730484385}, {"X"=175299.48464680242, "Y"=530166.620295045}, {"X"=175299.5206186963, "Y"=530166.667360014}, {"X"=175299.5570817157, "Y"=530166.7139596118}, {"X"=175299.59393444148, "Y"=530166.760246189}, {"X"=175299.63101704643, "Y"=530166.8075875615}, {"X"=175299.66873832993, "Y"=530166.8558371342}, {"X"=175299.70755977381, "Y"=530166.9049891003}, {"X"=175299.74702618556, "Y"=530166.954779551}, {"X"=175299.78702946118, "Y"=530167.0048947148}, {"X"=175299.8269780119, "Y"=530167.0550766316}, {"X"=175299.86691015412, "Y"=530167.1045016735}, {"X"=175299.9056200963, "Y"=530167.1539902581}, {"X"=175299.94444108658, "Y"=530167.202690514}, {"X"=175299.9832469312, "Y"=530167.2507615263}, {"X"=175300.02239172766, "Y"=530167.2984286564}, {"X"=175300.06160983795, "Y"=530167.3454263278}, {"X"=175300.10023907598, "Y"=530167.3924845605}, {"X"=175300.13795698716, "Y"=530167.4389938845}, {"X"=175300.17463229306, "Y"=530167.4854940797}, {"X"=175300.21027157555, "Y"=530167.53151233}, {"X"=175300.2456148467, "Y"=530167.5762784209}, {"X"=175300.28083256615, "Y"=530167.6208229107}, {"X"=175300.31683014592, "Y"=530167.6648911891}, {"X"=175300.35295156413, "Y"=530167.7092010507}, {"X"=175300.38885968522, "Y"=530167.754471571}, {"X"=175300.42531408952, "Y"=530167.7996572366}, {"X"=175300.4626722015, "Y"=530167.8446127126}, {"X"=175300.49978768127, "Y"=530167.8895922136}, {"X"=175300.5366776678, "Y"=530167.9350018955}, {"X"=175300.57296706524, "Y"=530167.9810026871}, {"X"=175300.60997343756, "Y"=530168.02653078}, {"X"=175300.64725950157, "Y"=530168.0722844577}, {"X"=175300.6848355032, "Y"=530168.1178341768}, {"X"=175300.72194708392, "Y"=530168.1629945957}, {"X"=175300.75843372697, "Y"=530168.2077007085}, {"X"=175300.79459920572, "Y"=530168.2516353095}, {"X"=175300.8309390622, "Y"=530168.2958279934}, {"X"=175300.86721646803, "Y"=530168.3407689049}, {"X"=175300.9041467231, "Y"=530168.3860186503}, {"X"=175300.94086441226, "Y"=530168.431876116}, {"X"=175300.97748970473, "Y"=530168.4773398549}, {"X"=175301.01311529457, "Y"=530168.5226245311}, {"X"=175301.04880451673, "Y"=530168.5675605212}, {"X"=175301.08470138145, "Y"=530168.6111218947}, {"X"=175301.11998015357, "Y"=530168.6544464744}, {"X"=175301.1544579749, "Y"=530168.6983050416}, {"X"=175301.1899404005, "Y"=530168.7422039253}, {"X"=175301.2262133977, "Y"=530168.787153732}, {"X"=175301.26329977365, "Y"=530168.8327792599}, {"X"=175301.30040072044, "Y"=530168.8794402435}, {"X"=175301.33783310797, "Y"=530168.9261524099}, {"X"=175301.37482062684, "Y"=530168.9724974196}, {"X"=175301.41083388752, "Y"=530169.0185789398}, {"X"=175301.44611475465, "Y"=530169.0635150287}, {"X"=175301.48104166967, "Y"=530169.107673044}, {"X"=175301.515584441, "Y"=530169.1522306317}, {"X"=175301.5505684368, "Y"=530169.1965216612}, {"X"=175301.58586430468, "Y"=530169.2408384063}, {"X"=175301.621437572, "Y"=530169.2849046132}, {"X"=175301.65624651004, "Y"=530169.3287078214}, {"X"=175301.69067446323, "Y"=530169.3715787638}, {"X"=175301.72433513994, "Y"=530169.4131889531}, {"X"=175301.7572057744, "Y"=530169.4545273413}, {"X"=175301.7897156011, "Y"=530169.4957669071}, {"X"=175301.82262842666, "Y"=530169.5363948606}, {"X"=175301.85541520052, "Y"=530169.5775315022}, {"X"=175301.88877971005, "Y"=530169.6193356836}, {"X"=175301.92198627733, "Y"=530169.6622479695}, {"X"=175301.9549979493, "Y"=530169.7066524813}, {"X"=175301.98874946675, "Y"=530169.7514277223}, {"X"=175302.02408231725, "Y"=530169.7962715428}, {"X"=175302.05988879167, "Y"=530169.84162117}, {"X"=175302.09521931363, "Y"=530169.886875645}, {"X"=175302.12915909418, "Y"=530169.9324128029}, {"X"=175302.16313239714, "Y"=530169.9770042623}, {"X"=175302.19741865405, "Y"=530170.0198878336}, {"X"=175302.23161996814, "Y"=530170.0622022983}, {"X"=175302.2647214002, "Y"=530170.1043091388}, {"X"=175302.29732747353, "Y"=530170.1466471837}, {"X"=175302.32942471874, "Y"=530170.1900533064}, {"X"=175302.36214685687, "Y"=530170.2339004164}, {"X"=175302.39546431036, "Y"=530170.2777679664}, {"X"=175302.42970125427, "Y"=530170.3213508952}, {"X"=175302.46371953157, "Y"=530170.3649755353}, {"X"=175302.4970483943, "Y"=530170.409108309}, {"X"=175302.53014454423, "Y"=530170.452725684}, {"X"=175302.56359763598, "Y"=530170.4957338027}, {"X"=175302.59699459223, "Y"=530170.5389285439}, {"X"=175302.63076028306, "Y"=530170.5819079936}, {"X"=175302.6641188947, "Y"=530170.625916373}, {"X"=175302.6977430426, "Y"=530170.6704567027}, {"X"=175302.7314268824, "Y"=530170.7154141635}, {"X"=175302.76559054904, "Y"=530170.7605799701}, {"X"=175302.80000400502, "Y"=530170.8048449432}, {"X"=175302.83450216462, "Y"=530170.8486979064}, {"X"=175302.868423361, "Y"=530170.8930431358}, {"X"=175302.9020594507, "Y"=530170.9368298354}, {"X"=175302.93501567593, "Y"=530170.9804587241}, {"X"=175302.96820232505, "Y"=530171.0238283353}, {"X"=175303.0014239085, "Y"=530171.0667294834}, {"X"=175303.03441731303, "Y"=530171.1100519415}, {"X"=175303.06691230068, "Y"=530171.153469102}, {"X"=175303.09917383848, "Y"=530171.1964219182}, {"X"=175303.13118923537, "Y"=530171.2397117508}, {"X"=175303.1637000194, "Y"=530171.2824795955}, {"X"=175303.19595648517, "Y"=530171.3261138815}, {"X"=175303.22875163666, "Y"=530171.3703914051}, {"X"=175303.26162110508, "Y"=530171.4149395159}, {"X"=175303.2943639709, "Y"=530171.4604080732}, {"X"=175303.3270933593, "Y"=530171.5061119605}, {"X"=175303.36078521397, "Y"=530171.5507863855}, {"X"=175303.39476642053, "Y"=530171.5950592977}, {"X"=175303.42826067653, "Y"=530171.6391105651}, {"X"=175303.46060070378, "Y"=530171.683447147}, {"X"=175303.4932010295, "Y"=530171.7277418941}, {"X"=175303.5264554045, "Y"=530171.7715508118}, {"X"=175303.56027406864, "Y"=530171.815673263}, {"X"=175303.59372100336, "Y"=530171.8604982444}, {"X"=175303.62725594908, "Y"=530171.9051320691}, {"X"=175303.66013932397, "Y"=530171.9501906737}, {"X"=175303.69312924595, "Y"=530171.9947339906}, {"X"=175303.72571887134, "Y"=530172.0390054631}, {"X"=175303.75856571438, "Y"=530172.0833916041}, {"X"=175303.7914979888, "Y"=530172.1276121215}, {"X"=175303.82426099747, "Y"=530172.1724058269}, {"X"=175303.85658823774, "Y"=530172.2175126894}, {"X"=175303.8893403862, "Y"=530172.2622276273}, {"X"=175303.9219982045, "Y"=530172.3070960032}, {"X"=175303.95487855875, "Y"=530172.3514321018}, {"X"=175303.98756941865, "Y"=530172.395190523}, {"X"=175304.0198873744, "Y"=530172.4383540505}, {"X"=175304.05146210626, "Y"=530172.4803022576}, {"X"=175304.08243248635, "Y"=530172.5218682386}, {"X"=175304.11302771606, "Y"=530172.5638781629}, {"X"=175304.14440576072, "Y"=530172.6058125234}, {"X"=175304.17647083785, "Y"=530172.6485317448}, {"X"=175304.2092485257, "Y"=530172.6916983553}, {"X"=175304.2421544904, "Y"=530172.7351098659}, {"X"=175304.27474581596, "Y"=530172.7793591394}, {"X"=175304.30713692037, "Y"=530172.8241972291}, {"X"=175304.33966600779, "Y"=530172.8692668731}, {"X"=175304.3725380399, "Y"=530172.9146862191}, {"X"=175304.40615073708, "Y"=530172.9595551069}, {"X"=175304.43922888403, "Y"=530173.0045820643}, {"X"=175304.47193721798, "Y"=530173.0500607167}, {"X"=175304.50408048517, "Y"=530173.095561017}, {"X"=175304.53664703757, "Y"=530173.1407204481}, {"X"=175304.57019344828, "Y"=530173.1850401526}, {"X"=175304.60417604624, "Y"=530173.229188761}, {"X"=175304.63733822326, "Y"=530173.274475177}, {"X"=175304.67012666404, "Y"=530173.3200845581}, {"X"=175304.70293440312, "Y"=530173.3656295104}, {"X"=175304.73601901694, "Y"=530173.4107485677}, {"X"=175304.7688052838, "Y"=530173.4550216836}, {"X"=175304.80180875398, "Y"=530173.4984595454}, {"X"=175304.83439683876, "Y"=530173.5410129662}, {"X"=175304.86641084577, "Y"=530173.5832384543}, {"X"=175304.89706473134, "Y"=530173.6259163404}, {"X"=175304.92851563115, "Y"=530173.6676274072}, {"X"=175304.96001501603, "Y"=530173.7089609802}, {"X"=175304.9911972434, "Y"=530173.7511778257}, {"X"=175305.0218017102, "Y"=530173.7939191228}, {"X"=175305.0528701443, "Y"=530173.8368965593}, {"X"=175305.0845467455, "Y"=530173.8803494384}, {"X"=175305.11676661787, "Y"=530173.9241980441}, {"X"=175305.1485606208, "Y"=530173.9687116023}, {"X"=175305.1810053819, "Y"=530174.0134252321}, {"X"=175305.21403351048, "Y"=530174.0580150564}, {"X"=175305.24728412752, "Y"=530174.1035575917}, {"X"=175305.28061614945, "Y"=530174.1499689076}, {"X"=175305.31471056672, "Y"=530174.1962902915}, {"X"=175305.3486507356, "Y"=530174.243170392}, {"X"=175305.3823800229, "Y"=530174.2900289173}, {"X"=175305.4154933949, "Y"=530174.3367893738}, {"X"=175305.4486278848, "Y"=530174.3826019497}, {"X"=175305.48151879795, "Y"=530174.4275195878}, {"X"=175305.5138967311, "Y"=530174.4724010066}, {"X"=175305.54595081756, "Y"=530174.517701799}, {"X"=175305.57926572644, "Y"=530174.562519407}, {"X"=175305.61313334163, "Y"=530174.6076283868}, {"X"=175305.64742550213, "Y"=530174.6531223445}, {"X"=175305.68094282097, "Y"=530174.6995930464}, {"X"=175305.7142195681, "Y"=530174.7464862061}, {"X"=175305.74732664338, "Y"=530174.7932144965}, {"X"=175305.78057287785, "Y"=530174.8402742251}, {"X"=175305.8133739154, "Y"=530174.8877536852}, {"X"=175305.84608374408, "Y"=530174.9352422942}, {"X"=175305.8802467283, "Y"=530174.9825878779}, {"X"=175305.91585264518, "Y"=530175.02962732}, {"X"=175305.95117603574, "Y"=530175.0772802396}, {"X"=175305.98675250847, "Y"=530175.1248480605}, {"X"=175306.0226269634, "Y"=530175.1719366532}, {"X"=175306.05766248834, "Y"=530175.219295199}, {"X"=175306.09146300732, "Y"=530175.2665819227}, {"X"=175306.1256061778, "Y"=530175.3138176922}, {"X"=175306.15987830423, "Y"=530175.3612284362}, {"X"=175306.19375731278, "Y"=530175.4089977182}, {"X"=175306.2272617157, "Y"=530175.4570955143}, {"X"=175306.26149442443, "Y"=530175.5043554353}, {"X"=175306.29601557076, "Y"=530175.5512049651}, {"X"=175306.33110052024, "Y"=530175.5979052205}, {"X"=175306.3664420601, "Y"=530175.6445070498}, {"X"=175306.40137430347, "Y"=530175.6922876495}, {"X"=175306.43611313298, "Y"=530175.7405627077}, {"X"=175306.47135692826, "Y"=530175.7888606924}, {"X"=175306.50683563814, "Y"=530175.836619701}, {"X"=175306.5427093849, "Y"=530175.8837704501}, {"X"=175306.57804036967, "Y"=530175.9312979346}, {"X"=175306.61314321528, "Y"=530175.9786596134}, {"X"=175306.64723720393, "Y"=530176.0260398111}, {"X"=175306.68197792507, "Y"=530176.0728576195}, {"X"=175306.71729545467, "Y"=530176.1191287831}, {"X"=175306.75288187485, "Y"=530176.1655689615}, {"X"=175306.78805515857, "Y"=530176.2121868278}, {"X"=175306.82317604765, "Y"=530176.2593597791}, {"X"=175306.85816065417, "Y"=530176.3068771907}, {"X"=175306.89302999235, "Y"=530176.3543549852}, {"X"=175306.92829042548, "Y"=530176.4019892259}, {"X"=175306.96434128538, "Y"=530176.4494269079}, {"X"=175307.0002629, "Y"=530176.4974909314}, {"X"=175307.03651319438, "Y"=530176.5461732863}, {"X"=175307.07280654478, "Y"=530176.5944370972}, {"X"=175307.10929617652, "Y"=530176.6425793526}, {"X"=175307.1459389947, "Y"=530176.6904026284}, {"X"=175307.1830941412, "Y"=530176.738340926}, {"X"=175307.2198662148, "Y"=530176.7870406077}, {"X"=175307.25608431565, "Y"=530176.836519937}, {"X"=175307.2923623031, "Y"=530176.8870823126}, {"X"=175307.32952882035, "Y"=530176.9370727075}, {"X"=175307.36630468437, "Y"=530176.9870564856}, {"X"=175307.40306440124, "Y"=530177.0369715019}, {"X"=175307.43982546963, "Y"=530177.0867444496}, {"X"=175307.47700678377, "Y"=530177.1363463515}, {"X"=175307.51413816065, "Y"=530177.1855366402}, {"X"=175307.55166098283, "Y"=530177.2347013578}, {"X"=175307.58907466935, "Y"=530177.2841050166}, {"X"=175307.62627763985, "Y"=530177.3341430286}, {"X"=175307.66311196302, "Y"=530177.3850267321}, {"X"=175307.7005225817, "Y"=530177.4357899772}, {"X"=175307.73824461747, "Y"=530177.486425782}, {"X"=175307.77605915256, "Y"=530177.5362899586}, {"X"=175307.81286147056, "Y"=530177.5865344778}, {"X"=175307.84951953805, "Y"=530177.6365241562}, {"X"=175307.88651088442, "Y"=530177.6859901074}, {"X"=175307.92401568915, "Y"=530177.7353546531}, {"X"=175307.9616221725, "Y"=530177.7846556385}, {"X"=175307.99953877402, "Y"=530177.8345883267}, {"X"=175308.03749193915, "Y"=530177.884904919}, {"X"=175308.07523145544, "Y"=530177.9354618721}, {"X"=175308.11299889255, "Y"=530177.9858755714}, {"X"=175308.15146935455, "Y"=530178.0352905402}, {"X"=175308.1892898605, "Y"=530178.0844787983}, {"X"=175308.2265397046, "Y"=530178.1335943816}, {"X"=175308.26328121778, "Y"=530178.1833474154}, {"X"=175308.30082930517, "Y"=530178.2326729915}, {"X"=175308.3391933072, "Y"=530178.2817331203}, {"X"=175308.37776592822, "Y"=530178.3309480151}, {"X"=175308.41586902775, "Y"=530178.3798457655}, {"X"=175308.45360439137, "Y"=530178.4289987606}, {"X"=175308.49054393347, "Y"=530178.4786213585}, {"X"=175308.52805617274, "Y"=530178.5275064252}, {"X"=175308.56581533956, "Y"=530178.5760211812}, {"X"=175308.60384613005, "Y"=530178.6241300373}, {"X"=175308.6412520306, "Y"=530178.6727002201}, {"X"=175308.67826697233, "Y"=530178.7214602334}, {"X"=175308.71486306612, "Y"=530178.7711648659}, {"X"=175308.75246034496, "Y"=530178.8215513228}, {"X"=175308.7912765256, "Y"=530178.872557922}, {"X"=175308.83084101314, "Y"=530178.9247021361}, {"X"=175308.8709113982, "Y"=530178.9771833654}, {"X"=175308.9109508622, "Y"=530179.0296935422}, {"X"=175308.95094127575, "Y"=530179.0814902235}, {"X"=175308.99123117467, "Y"=530179.1321184501}, {"X"=175309.03012990014, "Y"=530179.1819827599}, {"X"=175309.0674750189, "Y"=530179.2309682134}, {"X"=175309.1034754659, "Y"=530179.2796402158}, {"X"=175309.13934451604, "Y"=530179.327610065}, {"X"=175309.1753644265, "Y"=530179.3756738087}, {"X"=175309.21217135477, "Y"=530179.4232857344}, {"X"=175309.24893715564, "Y"=530179.4707690383}, {"X"=175309.28518585657, "Y"=530179.5189197841}, {"X"=175309.32090653412, "Y"=530179.5670399042}, {"X"=175309.35713197305, "Y"=530179.6151130308}, {"X"=175309.3934266228, "Y"=530179.6635266797}, {"X"=175309.42987620586, "Y"=530179.712513667}, {"X"=175309.46639058788, "Y"=530179.7624460628}, {"X"=175309.50371548356, "Y"=530179.8120852838}, {"X"=175309.5409782049, "Y"=530179.8619666371}, {"X"=175309.5787927472, "Y"=530179.9121404743}, {"X"=175309.61645778242, "Y"=530179.9635788811}, {"X"=175309.65459812188, "Y"=530180.0163932223}, {"X"=175309.69325909083, "Y"=530180.0694357668}, {"X"=175309.7317165625, "Y"=530180.122557711}, {"X"=175309.76908308847, "Y"=530180.1751967588}, {"X"=175309.80636802042, "Y"=530180.2269015467}, {"X"=175309.84373904276, "Y"=530180.2774640337}, {"X"=175309.88096197287, "Y"=530180.3267706002}, {"X"=175309.91734318458, "Y"=530180.3757034084}, {"X"=175309.9532567708, "Y"=530180.4237596989}, {"X"=175309.98798831712, "Y"=530180.472282293}, {"X"=175310.02238339974, "Y"=530180.5208502738}, {"X"=175310.0573020126, "Y"=530180.5694289177}, {"X"=175310.09330661935, "Y"=530180.6183128951}, {"X"=175310.12955154193, "Y"=530180.6672871724}, {"X"=175310.1658978246, "Y"=530180.7169914382}, {"X"=175310.20254698073, "Y"=530180.7669722736}, {"X"=175310.23967130386, "Y"=530180.817684213}, {"X"=175310.2773086728, "Y"=530180.8690550049}, {"X"=175310.3148211599, "Y"=530180.9201309427}, {"X"=175310.3511979726, "Y"=530180.9723744758}, {"X"=175310.38740139623, "Y"=530181.0252955357}, {"X"=175310.42416107788, "Y"=530181.0797110443}, {"X"=175310.4624049127, "Y"=530181.1348802013}, {"X"=175310.50164816767, "Y"=530181.1901351993}, {"X"=175310.54203527907, "Y"=530181.244894042}, {"X"=175310.58194975206, "Y"=530181.2991792613}, {"X"=175310.62001042886, "Y"=530181.3529172424}, {"X"=175310.65622358862, "Y"=530181.4049370685}, {"X"=175310.69123930926, "Y"=530181.4558061787}, {"X"=175310.72519802517, "Y"=530181.5047872087}, {"X"=175310.75874079563, "Y"=530181.5520969089}, {"X"=175310.79136085967, "Y"=530181.5980020331}, {"X"=175310.82360926468, "Y"=530181.6437328964}, {"X"=175310.85623968006, "Y"=530181.6907456301}, {"X"=175310.8897590421, "Y"=530181.7388267526}, {"X"=175310.9243145624, "Y"=530181.7880357637}, {"X"=175310.959343698, "Y"=530181.8383487933}, {"X"=175310.99435753067, "Y"=530181.8885797397}, {"X"=175311.0290962056, "Y"=530181.9392199271}, {"X"=175311.06388729028, "Y"=530181.990211786}, {"X"=175311.09868500763, "Y"=530182.0416486778}, {"X"=175311.13335366588, "Y"=530182.0931758506}, {"X"=175311.16810784728, "Y"=530182.1445684781}, {"X"=175311.20274703568, "Y"=530182.1960147172}, {"X"=175311.2379057422, "Y"=530182.2467135971}, {"X"=175311.27227776014, "Y"=530182.2976745092}, {"X"=175311.30606672564, "Y"=530182.3482675583}, {"X"=175311.3395601565, "Y"=530182.3986683643}, {"X"=175311.37393442274, "Y"=530182.448891213}, {"X"=175311.40852775157, "Y"=530182.4980068854}, {"X"=175311.44232597886, "Y"=530182.5478374333}, {"X"=175311.475157056, "Y"=530182.5983112288}, {"X"=175311.50801931764, "Y"=530182.6491478536}, {"X"=175311.54183613407, "Y"=530182.6998740053}, {"X"=175311.57663097818, "Y"=530182.7503397807}, {"X"=175311.61155363472, "Y"=530182.8014932929}, {"X"=175311.64626777923, "Y"=530182.8537284222}, {"X"=175311.68068305723, "Y"=530182.906743557}, {"X"=175311.7154702105, "Y"=530182.9591049955}, {"X"=175311.75001092287, "Y"=530183.0102019231}, {"X"=175311.78433634012, "Y"=530183.0606824049}, {"X"=175311.8183494312, "Y"=530183.1100850247}, {"X"=175311.8516716377, "Y"=530183.1588970209}, {"X"=175311.88408727964, "Y"=530183.2072721894}, {"X"=175311.91671428684, "Y"=530183.2552338662}, {"X"=175311.94992222873, "Y"=530183.3031472128}, {"X"=175311.98340970423, "Y"=530183.3515336459}, {"X"=175312.01677082642, "Y"=530183.4009259832}, {"X"=175312.0510007853, "Y"=530183.4505787942}, {"X"=175312.08557931965, "Y"=530183.5009863878}, {"X"=175312.12013653468, "Y"=530183.5522741646}, {"X"=175312.1542311072, "Y"=530183.6031737451}, {"X"=175312.1881540991, "Y"=530183.6538618514}, {"X"=175312.22243575216, "Y"=530183.7045222601}, {"X"=175312.25757506452, "Y"=530183.7549559459}, {"X"=175312.29278177244, "Y"=530183.8060153938}, {"X"=175312.32824544844, "Y"=530183.8574059312}, {"X"=175312.36394127307, "Y"=530183.9094206324}, {"X"=175312.4001556887, "Y"=530183.9609732128}, {"X"=175312.43641827087, "Y"=530184.0123380839}, {"X"=175312.4721263033, "Y"=530184.0636879449}, {"X"=175312.5069555313, "Y"=530184.1153023272}, {"X"=175312.54130807726, "Y"=530184.1674741576}, {"X"=175312.57628509818, "Y"=530184.2193444809}, {"X"=175312.61243834853, "Y"=530184.2708817059}, {"X"=175312.64919719583, "Y"=530184.3226235745}, {"X"=175312.68595615213, "Y"=530184.375303274}, {"X"=175312.72274589876, "Y"=530184.4288108387}, {"X"=175312.76002624852, "Y"=530184.4819762268}, {"X"=175312.79754509203, "Y"=530184.5349156114}, {"X"=175312.83499864914, "Y"=530184.5870438805}, {"X"=175312.8714617927, "Y"=530184.639437001}, {"X"=175312.90760069605, "Y"=530184.6915169893}, {"X"=175312.94404201457, "Y"=530184.7425184103}, {"X"=175312.98059682967, "Y"=530184.792660466}, {"X"=175313.01660241385, "Y"=530184.8418874011}, {"X"=175313.0520811022, "Y"=530184.891164725}, {"X"=175313.08734580636, "Y"=530184.9402695426}, {"X"=175313.12239439436, "Y"=530184.9893805474}, {"X"=175313.15734865, "Y"=530185.0386427735}, {"X"=175313.19286568387, "Y"=530185.0874072288}, {"X"=175313.22880935456, "Y"=530185.1363668718}, {"X"=175313.2649331918, "Y"=530185.1854447369}, {"X"=175313.30088473303, "Y"=530185.2346696118}, {"X"=175313.33722131583, "Y"=530185.2841008937}, {"X"=175313.37432573305, "Y"=530185.3331847425}, {"X"=175313.41198690207, "Y"=530185.3824289885}, {"X"=175313.449257545, "Y"=530185.4320095631}, {"X"=175313.48641791966, "Y"=530185.4820455073}, {"X"=175313.52345464373, "Y"=530185.5322027901}, {"X"=175313.56054014363, "Y"=530185.581779473}, {"X"=175313.59761448327, "Y"=530185.6311763932}, {"X"=175313.63479581906, "Y"=530185.6799115203}, {"X"=175313.67125340502, "Y"=530185.7286254782}, {"X"=175313.7071050316, "Y"=530185.7767130446}, {"X"=175313.74212418348, "Y"=530185.8236565841}, {"X"=175313.77722887165, "Y"=530185.8701692459}, {"X"=175313.8128344303, "Y"=530185.915917957}, {"X"=175313.8479152154, "Y"=530185.9618358053}, {"X"=175313.8821893614, "Y"=530186.0081600237}, {"X"=175313.9155590152, "Y"=530186.0544491778}, {"X"=175313.94968215242, "Y"=530186.1009303334}, {"X"=175313.98505024164, "Y"=530186.1469527704}, {"X"=175314.021090573, "Y"=530186.1929521351}, {"X"=175314.0570167525, "Y"=530186.2398907787}, {"X"=175314.0929765313, "Y"=530186.2871078982}, {"X"=175314.12863386451, "Y"=530186.3353935948}, {"X"=175314.16455866926, "Y"=530186.3845663889}, {"X"=175314.20138941368, "Y"=530186.4342648024}, {"X"=175314.2386463122, "Y"=530186.4848942381}, {"X"=175314.2759694681, "Y"=530186.5360639819}, {"X"=175314.31256280615, "Y"=530186.5878574002}, {"X"=175314.34945666775, "Y"=530186.638833074}, {"X"=175314.3865433375, "Y"=530186.6888093075}, {"X"=175314.42391436658, "Y"=530186.7372930504}, {"X"=175314.46051972595, "Y"=530186.7847590921}, {"X"=175314.49610486344, "Y"=530186.8319939679}, {"X"=175314.53065131142, "Y"=530186.8787435716}, {"X"=175314.56469552708, "Y"=530186.925797649}, {"X"=175314.5991626018, "Y"=530186.9729659047}, {"X"=175314.63475583828, "Y"=530187.0199443783}, {"X"=175314.6702479863, "Y"=530187.0677866219}, {"X"=175314.70570368378, "Y"=530187.1158842411}, {"X"=175314.74113296997, "Y"=530187.1637366577}, {"X"=175314.7767761707, "Y"=530187.2114375022}, {"X"=175314.8127982049, "Y"=530187.2590428923}, {"X"=175314.84901318164, "Y"=530187.3068952105}, {"X"=175314.88495516544, "Y"=530187.354989174}, {"X"=175314.92082059308, "Y"=530187.4035550535}, {"X"=175314.9563999271, "Y"=530187.4521262179}, {"X"=175314.99203503237, "Y"=530187.5000867952}, {"X"=175315.027573906, "Y"=530187.5481553137}, {"X"=175315.06366672198, "Y"=530187.5957349675}, {"X"=175315.09989612902, "Y"=530187.6433741514}, {"X"=175315.13577743215, "Y"=530187.6919177884}, {"X"=175315.17143027333, "Y"=530187.7407861799}, {"X"=175315.2078786093, "Y"=530187.7896733094}, {"X"=175315.24473079812, "Y"=530187.8379388351}, {"X"=175315.28113080456, "Y"=530187.8863588558}, {"X"=175315.3168192751, "Y"=530187.9346944091}, {"X"=175315.35221031535, "Y"=530187.9824947795}, {"X"=175315.3872724083, "Y"=530188.0301884642}, {"X"=175315.4232301929, "Y"=530188.0770360122}, {"X"=175315.45946732393, "Y"=530188.1242933825}, {"X"=175315.49556506728, "Y"=530188.172942929}, {"X"=175315.53165468454, "Y"=530188.2221396589}, {"X"=175315.5681028295, "Y"=530188.2712643011}, {"X"=175315.6050792257, "Y"=530188.319897936}, {"X"=175315.64205526988, "Y"=530188.3684117062}, {"X"=175315.67818000304, "Y"=530188.4163031384}, {"X"=175315.71349551325, "Y"=530188.4634256088}, {"X"=175315.7479487243, "Y"=530188.5107026764}, {"X"=175315.78355792633, "Y"=530188.5570928828}, {"X"=175315.8199135922, "Y"=530188.6030968745}, {"X"=175315.85587449878, "Y"=530188.6498034624}, {"X"=175315.890835794, "Y"=530188.6969602753}, {"X"=175315.92577562438, "Y"=530188.7449473259}, {"X"=175315.96154261148, "Y"=530188.7925767798}, {"X"=175315.99833612668, "Y"=530188.8407736705}, {"X"=175316.03534774587, "Y"=530188.8896380548}, {"X"=175316.07250852248, "Y"=530188.9386196402}, {"X"=175316.10918241073, "Y"=530188.9883018779}, {"X"=175316.14599503172, "Y"=530189.0375697273}, {"X"=175316.18267309142, "Y"=530189.0859634053}, {"X"=175316.21865495804, "Y"=530189.1340705757}, {"X"=175316.2542279634, "Y"=530189.1823032569}, {"X"=175316.28991713698, "Y"=530189.2311815331}, {"X"=175316.32575928187, "Y"=530189.2802680123}, {"X"=175316.36204323257, "Y"=530189.3298859186}, {"X"=175316.39863125872, "Y"=530189.3786882918}, {"X"=175316.43458270805, "Y"=530189.426994219}, {"X"=175316.4692830125, "Y"=530189.4751606653}, {"X"=175316.5038935927, "Y"=530189.5220388316}, {"X"=175316.5382121839, "Y"=530189.5681254207}, {"X"=175316.57219325224, "Y"=530189.6144993486}, {"X"=175316.60615941638, "Y"=530189.6612262579}, {"X"=175316.64103085897, "Y"=530189.7085542566}, {"X"=175316.67637426974, "Y"=530189.7564302428}, {"X"=175316.71164391257, "Y"=530189.8054218558}, {"X"=175316.74676780688, "Y"=530189.8548511842}, {"X"=175316.78219569896, "Y"=530189.9043395466}, {"X"=175316.8177323982, "Y"=530189.9537787547}, {"X"=175316.85369295246, "Y"=530190.0021701136}, {"X"=175316.8896444052, "Y"=530190.050779032}, {"X"=175316.92564777914, "Y"=530190.1001735788}, {"X"=175316.9620438199, "Y"=530190.1499565273}, {"X"=175316.99894420846, "Y"=530190.1998534118}, {"X"=175317.03558734115, "Y"=530190.2499219743}, {"X"=175317.07208662984, "Y"=530190.3004748595}, {"X"=175317.1083717217, "Y"=530190.3504823267}, {"X"=175317.1443335403, "Y"=530190.400203296}, {"X"=175317.18068957215, "Y"=530190.4502371901}, {"X"=175317.21824675493, "Y"=530190.4999789775}, {"X"=175317.25626110364, "Y"=530190.5500545918}, {"X"=175317.29395553737, "Y"=530190.6003819788}, {"X"=175317.3309519411, "Y"=530190.6512985411}, {"X"=175317.36805747618, "Y"=530190.7025765971}, {"X"=175317.40498688072, "Y"=530190.7539028961}, {"X"=175317.4429407785, "Y"=530190.8048066457}, {"X"=175317.48180363432, "Y"=530190.8554568817}, {"X"=175317.52073454688, "Y"=530190.9072578424}, {"X"=175317.55972893158, "Y"=530190.9592550602}, {"X"=175317.59894806604, "Y"=530191.0108720445}, {"X"=175317.6377611856, "Y"=530191.0620784669}, {"X"=175317.67635760055, "Y"=530191.1127916438}, {"X"=175317.7140501114, "Y"=530191.1633687577}, {"X"=175317.75095119307, "Y"=530191.2141035862}, {"X"=175317.78765461638, "Y"=530191.2650953768}, {"X"=175317.82558087553, "Y"=530191.3156396138}, {"X"=175317.86396142832, "Y"=530191.3661447766}, {"X"=175317.90213229894, "Y"=530191.4170345672}, {"X"=175317.94015622098, "Y"=530191.4673554361}, {"X"=175317.97785589864, "Y"=530191.5182610467}, {"X"=175318.0155045048, "Y"=530191.5692700257}, {"X"=175318.05364278206, "Y"=530191.620222066}, {"X"=175318.09153813362, "Y"=530191.6719994495}, {"X"=175318.1293183478, "Y"=530191.7246817079}, {"X"=175318.16774718426, "Y"=530191.7774419627}, {"X"=175318.20674981424, "Y"=530191.8298353782}, {"X"=175318.24521226567, "Y"=530191.8828796588}, {"X"=175318.28403795866, "Y"=530191.9350482963}, {"X"=175318.32304521388, "Y"=530191.9869078569}, {"X"=175318.36204793068, "Y"=530192.0384311461}, {"X"=175318.4005898055, "Y"=530192.0898758835}, {"X"=175318.43864458468, "Y"=530192.1416494689}, {"X"=175318.47640338843, "Y"=530192.1930820906}, {"X"=175318.51419378835, "Y"=530192.2441161796}, {"X"=175318.55208232062, "Y"=530192.2944862834}, {"X"=175318.58985834898, "Y"=530192.3451530531}, {"X"=175318.62736532633, "Y"=530192.3949971002}, {"X"=175318.66480275526, "Y"=530192.4440855398}, {"X"=175318.70216220792, "Y"=530192.4937657638}, {"X"=175318.74007465132, "Y"=530192.5435342542}, {"X"=175318.77838922056, "Y"=530192.5935956714}, {"X"=175318.81680214155, "Y"=530192.6436667865}, {"X"=175318.85473180335, "Y"=530192.6944685044}, {"X"=175318.893105015, "Y"=530192.7454908877}, {"X"=175318.93198027203, "Y"=530192.7964474163}, {"X"=175318.97074562093, "Y"=530192.847981396}, {"X"=175319.00950281188, "Y"=530192.8997518}, {"X"=175319.04856699263, "Y"=530192.9522948697}, {"X"=175319.08807038947, "Y"=530193.0047922492}, {"X"=175319.12802343152, "Y"=530193.0571762068}, {"X"=175319.16773230815, "Y"=530193.1099670911}, {"X"=175319.20749691897, "Y"=530193.1627333963}, {"X"=175319.24724586855, "Y"=530193.2155963047}, {"X"=175319.2868629425, "Y"=530193.2681954568}, {"X"=175319.32616219769, "Y"=530193.3205547077}, {"X"=175319.36573062692, "Y"=530193.3722783243}, {"X"=175319.4052265945, "Y"=530193.4237613154}, {"X"=175319.4445765745, "Y"=530193.4753002316}, {"X"=175319.48329824244, "Y"=530193.5267411147}, {"X"=175319.52202255937, "Y"=530193.5781808796}, {"X"=175319.56047417186, "Y"=530193.6296591858}, {"X"=175319.59880642896, "Y"=530193.6815151966}, {"X"=175319.6371569635, "Y"=530193.7326608438}, {"X"=175319.67575621096, "Y"=530193.7837424942}, {"X"=175319.71455607042, "Y"=530193.8343662901}, {"X"=175319.75346005248, "Y"=530193.8851551494}, {"X"=175319.7919885356, "Y"=530193.936569968}, {"X"=175319.83131689022, "Y"=530193.9879868631}, {"X"=175319.87087732382, "Y"=530194.0400046195}, {"X"=175319.91055584635, "Y"=530194.0927179083}, {"X"=175319.95018736875, "Y"=530194.1460129021}, {"X"=175319.99024830922, "Y"=530194.1992444766}, {"X"=175320.0305557881, "Y"=530194.2525741017}, {"X"=175320.0712095635, "Y"=530194.3052889514}, {"X"=175320.1119900287, "Y"=530194.3568103306}, {"X"=175320.15219124436, "Y"=530194.4083500657}, {"X"=175320.1921387411, "Y"=530194.458860601}, {"X"=175320.23155410215, "Y"=530194.5097467307}, {"X"=175320.2707313738, "Y"=530194.5609953767}, {"X"=175320.31042178915, "Y"=530194.6123379564}, {"X"=175320.35031262046, "Y"=530194.664057296}, {"X"=175320.3899530186, "Y"=530194.7158606148}, {"X"=175320.4297119804, "Y"=530194.767318418}, {"X"=175320.46997990887, "Y"=530194.8180544211}, {"X"=175320.51043847628, "Y"=530194.8688564525}, {"X"=175320.55115700723, "Y"=530194.9195034475}, {"X"=175320.5917810682, "Y"=530194.9702550462}, {"X"=175320.63193107033, "Y"=530195.0218526484}, {"X"=175320.67129892917, "Y"=530195.0737522215}, {"X"=175320.7100377912, "Y"=530195.1256225747}, {"X"=175320.74886255787, "Y"=530195.1768866911}, {"X"=175320.78829647583, "Y"=530195.2277594492}, {"X"=175320.82829674848, "Y"=530195.2781466381}, {"X"=175320.86779848064, "Y"=530195.3288871238}, {"X"=175320.90681250475, "Y"=530195.3794503614}, {"X"=175320.94602985482, "Y"=530195.429575715}, {"X"=175320.98480971038, "Y"=530195.4797301069}, {"X"=175321.02332181047, "Y"=530195.5292005048}, {"X"=175321.06128693797, "Y"=530195.57882124}, {"X"=175321.0995861466, "Y"=530195.6287894842}, {"X"=175321.1379527546, "Y"=530195.679084939}, {"X"=175321.17684378868, "Y"=530195.7290947222}, {"X"=175321.215752246, "Y"=530195.7787049029}, {"X"=175321.25457779068, "Y"=530195.8284340859}, {"X"=175321.2935347585, "Y"=530195.877373769}, {"X"=175321.33197582242, "Y"=530195.9267866664}, {"X"=175321.37019807613, "Y"=530195.9761924401}, {"X"=175321.40871088055, "Y"=530196.0256029064}, {"X"=175321.44677992928, "Y"=530196.0747216789}, {"X"=175321.48483888872, "Y"=530196.1231224035}, {"X"=175321.52257193413, "Y"=530196.1715429577}, {"X"=175321.56068217533, "Y"=530196.2202121164}, {"X"=175321.59924221472, "Y"=530196.2700208839}, {"X"=175321.63872254826, "Y"=530196.3210178126}, {"X"=175321.67865082875, "Y"=530196.3731266094}, {"X"=175321.71942213873, "Y"=530196.4266546473}, {"X"=175321.76037410757, "Y"=530196.4798691729}, {"X"=175321.80112038535, "Y"=530196.533019933}, {"X"=175321.8411714933, "Y"=530196.5856289156}, {"X"=175321.88069651256, "Y"=530196.6376612135}, {"X"=175321.9201304299, "Y"=530196.6885384173}, {"X"=175321.95949093453, "Y"=530196.7391528002}, {"X"=175321.99841810143, "Y"=530196.7900026427}, {"X"=175322.0373316636, "Y"=530196.8410456412}, {"X"=175322.0760458568, "Y"=530196.8926663568}, {"X"=175322.1152349461, "Y"=530196.9440259628}, {"X"=175322.1544901605, "Y"=530196.9952810451}, {"X"=175322.19440987587, "Y"=530197.0465907722}, {"X"=175322.23411659995, "Y"=530197.0980642746}, {"X"=175322.27372288413, "Y"=530197.1497212022}, {"X"=175322.31351665533, "Y"=530197.2012765786}, {"X"=175322.3533722951, "Y"=530197.2530859321}, {"X"=175322.39274468354, "Y"=530197.3041264676}, {"X"=175322.4312461575, "Y"=530197.3551040938}, {"X"=175322.4689193067, "Y"=530197.4054426665}, {"X"=175322.50720476272, "Y"=530197.454959244}, {"X"=175322.5459091693, "Y"=530197.5032659507}, {"X"=175322.58469188528, "Y"=530197.5513948477}, {"X"=175322.62243093, "Y"=530197.6003503415}, {"X"=175322.66002250477, "Y"=530197.64946276}, {"X"=175322.69777533837, "Y"=530197.6982894691}, {"X"=175322.7353187513, "Y"=530197.7469891632}, {"X"=175322.77224196383, "Y"=530197.7959381866}, {"X"=175322.80897855092, "Y"=530197.8452817602}, {"X"=175322.84632591892, "Y"=530197.8941851374}, {"X"=175322.88443607936, "Y"=530197.9437333102}, {"X"=175322.92386567718, "Y"=530197.9931510669}, {"X"=175322.96401642516, "Y"=530198.0432104138}, {"X"=175323.00403330493, "Y"=530198.0938306333}, {"X"=175323.04346028506, "Y"=530198.1450630171}, {"X"=175323.08229208103, "Y"=530198.196318245}, {"X"=175323.12123135975, "Y"=530198.2470748299}, {"X"=175323.15985042084, "Y"=530198.2982807423}, {"X"=175323.1988480503, "Y"=530198.3486997583}, {"X"=175323.23756583783, "Y"=530198.3991429065}, {"X"=175323.27665734818, "Y"=530198.4495583154}, {"X"=175323.31587152585, "Y"=530198.4992186585}, {"X"=175323.35479760286, "Y"=530198.5488043812}, {"X"=175323.39322686996, "Y"=530198.5981307524}, {"X"=175323.4315682364, "Y"=530198.6476860173}, {"X"=175323.46929583582, "Y"=530198.6969700654}, {"X"=175323.50722869192, "Y"=530198.7461702713}, {"X"=175323.5459397161, "Y"=530198.7946223526}, {"X"=175323.58439744834, "Y"=530198.8427899504}, {"X"=175323.62209566595, "Y"=530198.8917222602}, {"X"=175323.65877359055, "Y"=530198.9410005299}, {"X"=175323.69556244335, "Y"=530198.9900487311}, {"X"=175323.73411028614, "Y"=530199.0387354754}, {"X"=175323.77350876122, "Y"=530199.0881155926}, {"X"=175323.81290300708, "Y"=530199.1384646274}, {"X"=175323.85108638834, "Y"=530199.1891157913}, {"X"=175323.8888683214, "Y"=530199.2397037674}, {"X"=175323.92692682054, "Y"=530199.2885584359}, {"X"=175323.96485641086, "Y"=530199.3369540031}, {"X"=175324.00191990237, "Y"=530199.3851190561}, {"X"=175324.03842280654, "Y"=530199.4336209428}, {"X"=175324.07507156418, "Y"=530199.4829237162}, {"X"=175324.11335812218, "Y"=530199.5322183277}, {"X"=175324.15240360756, "Y"=530199.5817493182}, {"X"=175324.19127746008, "Y"=530199.6313518472}, {"X"=175324.2287002106, "Y"=530199.6817921636}, {"X"=175324.26553019526, "Y"=530199.7321742966}, {"X"=175324.30255214145, "Y"=530199.7815691971}, {"X"=175324.33997542586, "Y"=530199.8309895523}, {"X"=175324.3778948948, "Y"=530199.8801598336}, {"X"=175324.41578257747, "Y"=530199.929665387}, {"X"=175324.45303470409, "Y"=530199.9793193169}, {"X"=175324.49021220786, "Y"=530200.0288991062}, {"X"=175324.52719458667, "Y"=530200.0780943516}, {"X"=175324.56453317933, "Y"=530200.126432844}, {"X"=175324.6018519318, "Y"=530200.1752519632}, {"X"=175324.639619019, "Y"=530200.2247134796}, {"X"=175324.67763583743, "Y"=530200.2756559197}, {"X"=175324.71633669882, "Y"=530200.3275730183}, {"X"=175324.75549563722, "Y"=530200.3789316149}, {"X"=175324.79472103066, "Y"=530200.4299981245}, {"X"=175324.83290145468, "Y"=530200.4805516311}, {"X"=175324.8698345541, "Y"=530200.5307581061}, {"X"=175324.90571872293, "Y"=530200.5803106372}, {"X"=175324.94164630468, "Y"=530200.6292659377}, {"X"=175324.9781788097, "Y"=530200.6769974988}, {"X"=175325.01496359013, "Y"=530200.723770505}, {"X"=175325.05083836144, "Y"=530200.7713397482}, {"X"=175325.08665947133, "Y"=530200.8193353349}, {"X"=175325.12301564822, "Y"=530200.8679497532}, {"X"=175325.1597467984, "Y"=530200.9175597209}, {"X"=175325.1965801437, "Y"=530200.9678830262}, {"X"=175325.23368578497, "Y"=530201.0192288171}, {"X"=175325.27100025493, "Y"=530201.0708015133}, {"X"=175325.3086159226, "Y"=530201.1226851918}, {"X"=175325.3462306779, "Y"=530201.173658787}, {"X"=175325.38365508235, "Y"=530201.224064698}, {"X"=175325.42044835156, "Y"=530201.2740152087}, {"X"=175325.4568644001, "Y"=530201.3231078014}, {"X"=175325.49279309702, "Y"=530201.3721430111}, {"X"=175325.5287187662, "Y"=530201.4210528162}, {"X"=175325.56390410103, "Y"=530201.4709259429}, {"X"=175325.59903368057, "Y"=530201.5214163167}, {"X"=175325.63438651664, "Y"=530201.5719193501}, {"X"=175325.67106088204, "Y"=530201.6224007264}, {"X"=175325.70852292405, "Y"=530201.672954138}, {"X"=175325.74600077514, "Y"=530201.724963639}, {"X"=175325.78311414344, "Y"=530201.7780296917}, {"X"=175325.8204649508, "Y"=530201.8323125597}, {"X"=175325.85848104864, "Y"=530201.8872194239}, {"X"=175325.89734364732, "Y"=530201.9414190304}, {"X"=175325.93574889482, "Y"=530201.9949218861}, {"X"=175325.9731610076, "Y"=530202.0477684161}, {"X"=175326.00978406958, "Y"=530202.100076773}, {"X"=175326.0468937723, "Y"=530202.1507011494}, {"X"=175326.083703109, "Y"=530202.2006971186}, {"X"=175326.11978964065, "Y"=530202.2500903491}, {"X"=175326.15506203403, "Y"=530202.2991508055}, {"X"=175326.18999830802, "Y"=530202.3477727488}, {"X"=175326.2249742177, "Y"=530202.3954179}, {"X"=175326.26010835878, "Y"=530202.4426541552}, {"X"=175326.2947142973, "Y"=530202.4894968602}, {"X"=175326.32881687392, "Y"=530202.536559692}, {"X"=175326.36266935102, "Y"=530202.5844190321}, {"X"=175326.39759400964, "Y"=530202.6330077152}, {"X"=175326.43383685724, "Y"=530202.683445973}, {"X"=175326.47190138185, "Y"=530202.7349532002}, {"X"=175326.51121043155, "Y"=530202.7876609504}, {"X"=175326.55136520957, "Y"=530202.8415015922}, {"X"=175326.59171968058, "Y"=530202.8960752623}, {"X"=175326.6321905429, "Y"=530202.9510703352}, {"X"=175326.6722261586, "Y"=530203.0062542596}, {"X"=175326.71219305095, "Y"=530203.0615638003}, {"X"=175326.75209383233, "Y"=530203.116381868}, {"X"=175326.7917454435, "Y"=530203.1711107733}, {"X"=175326.83161576497, "Y"=530203.2246126398}, {"X"=175326.87189651153, "Y"=530203.2770178622}, {"X"=175326.91170643645, "Y"=530203.3286631126}, {"X"=175326.9508110747, "Y"=530203.3796411991}, {"X"=175326.98866926372, "Y"=530203.4302678084}, {"X"=175327.02652639092, "Y"=530203.4799343928}, {"X"=175327.06383915478, "Y"=530203.5291353314}, {"X"=175327.1012313738, "Y"=530203.5773460448}, {"X"=175327.13767728163, "Y"=530203.62515778}, {"X"=175327.1733785629, "Y"=530203.6724767144}, {"X"=175327.20888498292, "Y"=530203.7192002304}, {"X"=175327.24457231665, "Y"=530203.7662961268}, {"X"=175327.28073190898, "Y"=530203.8137380134}, {"X"=175327.31828937924, "Y"=530203.8621169378}, {"X"=175327.3568467017, "Y"=530203.9113286342}, {"X"=175327.39573231337, "Y"=530203.9613273641}, {"X"=175327.4348463128, "Y"=530204.0118770179}, {"X"=175327.4746820218, "Y"=530204.0623568422}, {"X"=175327.51439785375, "Y"=530204.1136372288}, {"X"=175327.55409277766, "Y"=530204.1650364326}, {"X"=175327.59377426372, "Y"=530204.2166853956}, {"X"=175327.63384299536, "Y"=530204.2683875972}, {"X"=175327.67389632692, "Y"=530204.3193728758}, {"X"=175327.71366109003, "Y"=530204.3698262745}, {"X"=175327.75270769326, "Y"=530204.419750169}, {"X"=175327.7914221135, "Y"=530204.4690701697}, {"X"=175327.82960123813, "Y"=530204.517694761}, {"X"=175327.86709288435, "Y"=530204.5662825343}, {"X"=175327.9041485433, "Y"=530204.6145086712}, {"X"=175327.94210074993, "Y"=530204.6615801282}, {"X"=175327.9798551974, "Y"=530204.7091738019}, {"X"=175328.0173480477, "Y"=530204.7569702436}, {"X"=175328.05459147744, "Y"=530204.8057918225}, {"X"=175328.09215344326, "Y"=530204.8553971305}, {"X"=175328.13028118102, "Y"=530204.9055201834}, {"X"=175328.16931487413, "Y"=530204.9561744055}, {"X"=175328.20865300385, "Y"=530205.0073360448}, {"X"=175328.24843108968, "Y"=530205.0590047016}, {"X"=175328.28835976106, "Y"=530205.110072481}, {"X"=175328.3279304532, "Y"=530205.1607994803}, {"X"=175328.36635310898, "Y"=530205.2115076702}, {"X"=175328.4048222024, "Y"=530205.2614421498}, {"X"=175328.44354148043, "Y"=530205.3115112955}, {"X"=175328.48294085654, "Y"=530205.3621167176}, {"X"=175328.52195241617, "Y"=530205.4139774231}, {"X"=175328.56165370328, "Y"=530205.4657362077}, {"X"=175328.60110805032, "Y"=530205.5175612008}, {"X"=175328.6405652865, "Y"=530205.568864554}, {"X"=175328.6796272788, "Y"=530205.619805039}, {"X"=175328.71811733616, "Y"=530205.670242225}, {"X"=175328.75615469483, "Y"=530205.7197573447}, {"X"=175328.79388382484, "Y"=530205.7689803721}, {"X"=175328.83173539452, "Y"=530205.8179721874}, {"X"=175328.86998914456, "Y"=530205.8666753601}, {"X"=175328.90845591988, "Y"=530205.9152258562}, {"X"=175328.94701416916, "Y"=530205.9638582114}, {"X"=175328.98495470296, "Y"=530206.0135811617}, {"X"=175329.02283770952, "Y"=530206.063320929}, {"X"=175329.061211757, "Y"=530206.1137684488}, {"X"=175329.1004535877, "Y"=530206.1644198417}, {"X"=175329.13965264565, "Y"=530206.215584116}, {"X"=175329.17943126732, "Y"=530206.2665369152}, {"X"=175329.21919262805, "Y"=530206.3173443769}, {"X"=175329.25909633044, "Y"=530206.3683600716}, {"X"=175329.29923168753, "Y"=530206.4189333583}, {"X"=175329.33950991664, "Y"=530206.4692942395}, {"X"=175329.37883474256, "Y"=530206.5198543807}, {"X"=175329.4174794207, "Y"=530206.5710624671}, {"X"=175329.45618161428, "Y"=530206.6222492951}, {"X"=175329.49601390955, "Y"=530206.6721808698}, {"X"=175329.53568236195, "Y"=530206.7218221434}, {"X"=175329.57487133163, "Y"=530206.7710708327}, {"X"=175329.61317725817, "Y"=530206.8203476531}, {"X"=175329.65166145592, "Y"=530206.868802654}, {"X"=175329.69034324563, "Y"=530206.9169784943}, {"X"=175329.72884437937, "Y"=530206.9657686227}, {"X"=175329.76712680032, "Y"=530207.0151864667}, {"X"=175329.80580621227, "Y"=530207.0652579557}, {"X"=175329.84515547164, "Y"=530207.1153951712}, {"X"=175329.88507176263, "Y"=530207.1655773262}, {"X"=175329.92491169384, "Y"=530207.2159972164}, {"X"=175329.96473889175, "Y"=530207.2666047115}, {"X"=175330.0045233484, "Y"=530207.3177372969}, {"X"=175330.04477562633, "Y"=530207.3689128957}, {"X"=175330.08507576596, "Y"=530207.4206987759}, {"X"=175330.12605519747, "Y"=530207.4715492621}, {"X"=175330.16637356245, "Y"=530207.5226070208}, {"X"=175330.20511206114, "Y"=530207.5740934082}, {"X"=175330.24271986936, "Y"=530207.6257351815}, {"X"=175330.2810642061, "Y"=530207.6763248568}, {"X"=175330.31986330473, "Y"=530207.7258344068}, {"X"=175330.35768402094, "Y"=530207.775783018}, {"X"=175330.39437893714, "Y"=530207.8254430583}, {"X"=175330.4313906394, "Y"=530207.874092192}, {"X"=175330.46888017948, "Y"=530207.921375898}, {"X"=175330.50616064473, "Y"=530207.9677490287}, {"X"=175330.5426012657, "Y"=530208.0146817855}, {"X"=175330.57887375378, "Y"=530208.0619724141}, {"X"=175330.61506270058, "Y"=530208.1103698179}, {"X"=175330.65235307286, "Y"=530208.1595009197}, {"X"=175330.6898371192, "Y"=530208.2097268798}, {"X"=175330.72784761153, "Y"=530208.2603519466}, {"X"=175330.7657841934, "Y"=530208.3108440499}, {"X"=175330.80350983172, "Y"=530208.361594262}, {"X"=175330.84116910724, "Y"=530208.4123679763}, {"X"=175330.8800341823, "Y"=530208.4632258139}, {"X"=175330.91904552278, "Y"=530208.5144217251}, {"X"=175330.95728834765, "Y"=530208.5660349927}, {"X"=175330.99433718255, "Y"=530208.6182655349}, {"X"=175331.0318488113, "Y"=530208.6688343638}, {"X"=175331.06905319763, "Y"=530208.7185461762}, {"X"=175331.10566655878, "Y"=530208.7675871584}, {"X"=175331.14137250715, "Y"=530208.8168039559}, {"X"=175331.17715414436, "Y"=530208.8661548237}, {"X"=175331.21332360696, "Y"=530208.9154568233}, {"X"=175331.25029619085, "Y"=530208.9649606678}, {"X"=175331.2873574178, "Y"=530209.0144875587}, {"X"=175331.32414960433, "Y"=530209.0643948126}, {"X"=175331.36084215975, "Y"=530209.114159192}, {"X"=175331.3975425129, "Y"=530209.1638647242}, {"X"=175331.43446336297, "Y"=530209.2144497242}, {"X"=175331.47308668031, "Y"=530209.2647300402}, {"X"=175331.51153533268, "Y"=530209.315855475}, {"X"=175331.54889317372, "Y"=530209.3674425003}, {"X"=175331.5855494454, "Y"=530209.4196220397}, {"X"=175331.62295978758, "Y"=530209.4709902672}, {"X"=175331.66061267612, "Y"=530209.5217040731}, {"X"=175331.69814321943, "Y"=530209.5723827237}, {"X"=175331.73536540987, "Y"=530209.6233275409}, {"X"=175331.77258882776, "Y"=530209.6746885533}, {"X"=175331.80997591818, "Y"=530209.7262832607}, {"X"=175331.8481199299, "Y"=530209.7774340136}, {"X"=175331.88623244286, "Y"=530209.8287158216}, {"X"=175331.9241847472, "Y"=530209.8794387324}, {"X"=175331.96143662307, "Y"=530209.9299384085}, {"X"=175331.99790744064, "Y"=530209.9799065489}, {"X"=175332.03363035072, "Y"=530210.0303718917}, {"X"=175332.07052518567, "Y"=530210.0802477727}, {"X"=175332.10833857156, "Y"=530210.1304217139}, {"X"=175332.14653489395, "Y"=530210.1818897336}, {"X"=175332.1846024039, "Y"=530210.2341328121}, {"X"=175332.22300738035, "Y"=530210.2869697822}, {"X"=175332.2621362657, "Y"=530210.339582644}, {"X"=175332.30199405577, "Y"=530210.3918626182}, {"X"=175332.34141600237, "Y"=530210.4441305593}, {"X"=175332.38041804795, "Y"=530210.4963853122}, {"X"=175332.4185211116, "Y"=530210.5486704636}, {"X"=175332.45682697443, "Y"=530210.5997386106}, {"X"=175332.49514308042, "Y"=530210.6506768743}, {"X"=175332.53412157384, "Y"=530210.7006542655}, {"X"=175332.57272378285, "Y"=530210.7512909137}, {"X"=175332.61101197888, "Y"=530210.8029773051}, {"X"=175332.64921056182, "Y"=530210.8558148851}, {"X"=175332.68851538797, "Y"=530210.9095182215}, {"X"=175332.72771294997, "Y"=530210.9640942254}, {"X"=175332.76750234602, "Y"=530211.0190136484}, {"X"=175332.80752506072, "Y"=530211.0731554804}, {"X"=175332.84765670967, "Y"=530211.1269895624}, {"X"=175332.88795444716, "Y"=530211.1803758806}, {"X"=175332.92839109115, "Y"=530211.234007068}, {"X"=175332.96848531367, "Y"=530211.2886669956}, {"X"=175333.0089040344, "Y"=530211.3437299544}, {"X"=175333.0491415058, "Y"=530211.3989066537}, {"X"=175333.08910233053, "Y"=530211.4539887221}, {"X"=175333.1285585995, "Y"=530211.5088869324}, {"X"=175333.16815412405, "Y"=530211.5626471259}, {"X"=175333.20753422027, "Y"=530211.6163446938}, {"X"=175333.2473421582, "Y"=530211.6697457767}, {"X"=175333.28705198405, "Y"=530211.724119386}, {"X"=175333.3265540142, "Y"=530211.779216127}, {"X"=175333.3660775373, "Y"=530211.8349931492}, {"X"=175333.40622949848, "Y"=530211.8900102822}, {"X"=175333.44650034822, "Y"=530211.9444932247}, {"X"=175333.48723672854, "Y"=530211.9985430562}, {"X"=175333.52736064664, "Y"=530212.0530630564}, {"X"=175333.56740341955, "Y"=530212.1080017141}, {"X"=175333.6077093309, "Y"=530212.1626599086}, {"X"=175333.64857199727, "Y"=530212.2168813988}, {"X"=175333.68922026566, "Y"=530212.2707905404}, {"X"=175333.72890749428, "Y"=530212.3247113958}, {"X"=175333.76778450757, "Y"=530212.3784270975}, {"X"=175333.80736747183, "Y"=530212.4321351693}, {"X"=175333.84828877196, "Y"=530212.4858159842}, {"X"=175333.88984022452, "Y"=530212.539917797}, {"X"=175333.93109660895, "Y"=530212.5948872815}, {"X"=175333.97284515807, "Y"=530212.6497432184}, {"X"=175334.0142686215, "Y"=530212.7046001133}, {"X"=175334.05544437704, "Y"=530212.7586608616}, {"X"=175334.0959890387, "Y"=530212.8128810698}, {"X"=175334.13627522383, "Y"=530212.8671608662}, {"X"=175334.17651603464, "Y"=530212.9222742985}, {"X"=175334.2177644458, "Y"=530212.9772438075}, {"X"=175334.25957639978, "Y"=530213.0322760266}, {"X"=175334.30213095952, "Y"=530213.0865147257}, {"X"=175334.34455506905, "Y"=530213.1406738986}, {"X"=175334.38594238626, "Y"=530213.195288953}, {"X"=175334.42704816477, "Y"=530213.2499525625}, {"X"=175334.46824282644, "Y"=530213.3047191269}, {"X"=175334.50961381703, "Y"=530213.3595051488}, {"X"=175334.55108627415, "Y"=530213.4141565791}, {"X"=175334.59266786097, "Y"=530213.4679675244}, {"X"=175334.63399788298, "Y"=530213.5211776675}, {"X"=175334.6750819692, "Y"=530213.573293105}, {"X"=175334.71570326976, "Y"=530213.6252711763}, {"X"=175334.75589895574, "Y"=530213.6780007676}, {"X"=175334.79658751158, "Y"=530213.7311584209}, {"X"=175334.83711118187, "Y"=530213.7854730334}, {"X"=175334.87751620755, "Y"=530213.8401054167}, {"X"=175334.9179042401, "Y"=530213.894081924}, {"X"=175334.95911596806, "Y"=530213.9465288344}, {"X"=175334.99991220928, "Y"=530213.9986573323}, {"X"=175335.04026648914, "Y"=530214.050201127}, {"X"=175335.08012203232, "Y"=530214.1026320615}, {"X"=175335.12058568108, "Y"=530214.1555184657}, {"X"=175335.16164489972, "Y"=530214.2088137578}, {"X"=175335.2026623043, "Y"=530214.2629493396}, {"X"=175335.24292566493, "Y"=530214.317904002}, {"X"=175335.2838600399, "Y"=530214.3724194007}, {"X"=175335.32589039847, "Y"=530214.4264254693}, {"X"=175335.36913003057, "Y"=530214.4801915719}, {"X"=175335.4125249086, "Y"=530214.5343367882}, {"X"=175335.45555095756, "Y"=530214.5889669928}, {"X"=175335.49830331592, "Y"=530214.6433027806}, {"X"=175335.54073540578, "Y"=530214.6974685959}, {"X"=175335.58196774634, "Y"=530214.7521007617}, {"X"=175335.62354322325, "Y"=530214.8059483555}, {"X"=175335.66565024323, "Y"=530214.8586179304}, {"X"=175335.70747625933, "Y"=530214.9106157594}, {"X"=175335.7480881228, "Y"=530214.963002292}, {"X"=175335.7885573149, "Y"=530215.0144669515}, {"X"=175335.82880391076, "Y"=530215.0658434787}, {"X"=175335.86905572907, "Y"=530215.1162866012}, {"X"=175335.909482951, "Y"=530215.1667380838}, {"X"=175335.95024341732, "Y"=530215.2175526178}, {"X"=175335.9909282017, "Y"=530215.2700366036}, {"X"=175336.03225353497, "Y"=530215.3231646375}, {"X"=175336.0742294917, "Y"=530215.3758479197}, {"X"=175336.1162228887, "Y"=530215.4281371495}, {"X"=175336.15780792251, "Y"=530215.480420926}, {"X"=175336.198753351, "Y"=530215.5338830402}, {"X"=175336.2400447598, "Y"=530215.5884240265}, {"X"=175336.28280096015, "Y"=530215.6431649067}, {"X"=175336.32627274963, "Y"=530215.697862611}, {"X"=175336.3695396637, "Y"=530215.7518728063}, {"X"=175336.41189431006, "Y"=530215.8050133444}, {"X"=175336.4530581296, "Y"=530215.857140764}, {"X"=175336.4923324384, "Y"=530215.9083226097}, {"X"=175336.53024073623, "Y"=530215.9582587824}, {"X"=175336.56758054454, "Y"=530216.0079569012}, {"X"=175336.60624975662, "Y"=530216.0567010613}, {"X"=175336.64522401133, "Y"=530216.1052567544}, {"X"=175336.68329837156, "Y"=530216.1538350807}, {"X"=175336.72042406868, "Y"=530216.2021165418}, {"X"=175336.75789178454, "Y"=530216.2498342964}, {"X"=175336.79601195845, "Y"=530216.2977277045}, {"X"=175336.83490120104, "Y"=530216.3474945049}, {"X"=175336.8747391946, "Y"=530216.3987878956}, {"X"=175336.9155644031, "Y"=530216.4511349584}, {"X"=175336.9565872925, "Y"=530216.5038343738}, {"X"=175336.99702923294, "Y"=530216.5562757964}, {"X"=175337.03653662247, "Y"=530216.608701107}, {"X"=175337.07562676386, "Y"=530216.6599112444}, {"X"=175337.11431845836, "Y"=530216.7105731766}, {"X"=175337.15316399393, "Y"=530216.7608384356}, {"X"=175337.19213873718, "Y"=530216.8122653349}, {"X"=175337.232309873, "Y"=530216.8641903627}, {"X"=175337.27302243776, "Y"=530216.9167896998}, {"X"=175337.31390302093, "Y"=530216.9698935254}, {"X"=175337.3542175054, "Y"=530217.0235705986}, {"X"=175337.39383505605, "Y"=530217.0782097556}, {"X"=175337.43345427106, "Y"=530217.1331130541}, {"X"=175337.4731671136, "Y"=530217.1885266124}, {"X"=175337.51269825146, "Y"=530217.2435999815}, {"X"=175337.55194491986, "Y"=530217.2977274793}, {"X"=175337.59038441366, "Y"=530217.3505776902}, {"X"=175337.62842923752, "Y"=530217.40235916}, {"X"=175337.6661001939, "Y"=530217.4535179922}, {"X"=175337.70416076016, "Y"=530217.5037300759}, {"X"=175337.7420038972, "Y"=530217.5544022826}, {"X"=175337.7794317696, "Y"=530217.6051323175}, {"X"=175337.81701866104, "Y"=530217.6563202547}, {"X"=175337.8544032769, "Y"=530217.708001567}, {"X"=175337.8925377935, "Y"=530217.7595608027}, {"X"=175337.93128742423, "Y"=530217.8109495258}, {"X"=175337.9695507337, "Y"=530217.8629301275}, {"X"=175338.0082516581, "Y"=530217.9152235296}, {"X"=175338.04761985684, "Y"=530217.967611521}, {"X"=175338.08728319546, "Y"=530218.0209597816}, {"X"=175338.1271335317, "Y"=530218.0749423284}, {"X"=175338.16702309356, "Y"=530218.1290091096}, {"X"=175338.20661768012, "Y"=530218.1830734315}, {"X"=175338.2461740608, "Y"=530218.2367982493}, {"X"=175338.28507050654, "Y"=530218.2905139152}, {"X"=175338.32402685797, "Y"=530218.3435179845}, {"X"=175338.3628983841, "Y"=530218.3962936742}, {"X"=175338.40248170623, "Y"=530218.4477409829}, {"X"=175338.44199884526, "Y"=530218.4989731741}, {"X"=175338.4810465143, "Y"=530218.5499037582}, {"X"=175338.51934318643, "Y"=530218.600885391}, {"X"=175338.55710943416, "Y"=530218.6522204147}, {"X"=175338.5948762553, "Y"=530218.7037507715}, {"X"=175338.6338252904, "Y"=530218.7548769822}, {"X"=175338.6739002579, "Y"=530218.8060364973}, {"X"=175338.71384854216, "Y"=530218.8583928163}, {"X"=175338.753222827, "Y"=530218.9113457106}, {"X"=175338.792356318, "Y"=530218.9646467023}, {"X"=175338.8311580059, "Y"=530219.01837153}, {"X"=175338.87071642242, "Y"=530219.0715880294}, {"X"=175338.91075334582, "Y"=530219.1254668134}, {"X"=175338.95190623117, "Y"=530219.1793034604}, {"X"=175338.99320496703, "Y"=530219.2336380056}, {"X"=175339.03450596903, "Y"=530219.2878393602}, {"X"=175339.07593600373, "Y"=530219.3419426669}, {"X"=175339.1173234146, "Y"=530219.3954090409}, {"X"=175339.15756587937, "Y"=530219.4490019855}, {"X"=175339.196607049, "Y"=530219.5022366615}, {"X"=175339.23502417348, "Y"=530219.5550181346}, {"X"=175339.27417272714, "Y"=530219.6071215451}, {"X"=175339.31415161595, "Y"=530219.6584433867}, {"X"=175339.35397403524, "Y"=530219.7095736838}, {"X"=175339.3928394618, "Y"=530219.7608854916}, {"X"=175339.43153280398, "Y"=530219.8121156775}, {"X"=175339.4711378264, "Y"=530219.8631167639}, {"X"=175339.5113195704, "Y"=530219.9153447627}, {"X"=175339.5514793716, "Y"=530219.968542844}, {"X"=175339.59169131416, "Y"=530220.0223001395}, {"X"=175339.63130955625, "Y"=530220.077183476}, {"X"=175339.6713096225, "Y"=530220.1317837801}, {"X"=175339.71162398445, "Y"=530220.1860302234}, {"X"=175339.75238126508, "Y"=530220.2396849147}, {"X"=175339.79291413393, "Y"=530220.2938363759}, {"X"=175339.8341795131, "Y"=530220.3476771363}, {"X"=175339.87538622756, "Y"=530220.4017489201}, {"X"=175339.91570330068, "Y"=530220.4557134501}, {"X"=175339.95501255686, "Y"=530220.5094489943}, {"X"=175339.99378179503, "Y"=530220.5623881428}, {"X"=175340.032220397, "Y"=530220.614045269}, {"X"=175340.0706813909, "Y"=530220.6642850373}, {"X"=175340.1095277134, "Y"=530220.7136280148}, {"X"=175340.1483784491, "Y"=530220.7632662015}, {"X"=175340.1866975091, "Y"=530220.8131345876}, {"X"=175340.22491300027, "Y"=530220.8627269252}, {"X"=175340.26314188118, "Y"=530220.9126532906}, {"X"=175340.30124549245, "Y"=530220.9624546103}, {"X"=175340.3389347308, "Y"=530221.0126145277}, {"X"=175340.3772862895, "Y"=530221.0623907007}, {"X"=175340.41577064258, "Y"=530221.1127436082}, {"X"=175340.45473172294, "Y"=530221.1634558148}, {"X"=175340.49399150687, "Y"=530221.2139340698}, {"X"=175340.53319028806, "Y"=530221.2641516883}, {"X"=175340.57132779274, "Y"=530221.3143324822}, {"X"=175340.60874069866, "Y"=530221.3645043136}, {"X"=175340.64630832113, "Y"=530221.4133749353}, {"X"=175340.68330462027, "Y"=530221.4616479168}, {"X"=175340.7200604363, "Y"=530221.5097728887}, {"X"=175340.7568127796, "Y"=530221.5576215149}, {"X"=175340.79352235922, "Y"=530221.6056866894}, {"X"=175340.83133687428, "Y"=530221.6532746962}, {"X"=175340.86972653927, "Y"=530221.701257226}, {"X"=175340.9080893437, "Y"=530221.7497437114}, {"X"=175340.9458108464, "Y"=530221.7991321841}, {"X"=175340.98414187023, "Y"=530221.8497574623}, {"X"=175341.02349582317, "Y"=530221.9009324348}, {"X"=175341.06375182403, "Y"=530221.9531158272}, {"X"=175341.1044829561, "Y"=530222.005719567}, {"X"=175341.14595957266, "Y"=530222.0579060195}, {"X"=175341.1872804957, "Y"=530222.1101617429}, {"X"=175341.2283713614, "Y"=530222.1619009508}, {"X"=175341.26824615517, "Y"=530222.213376271}, {"X"=175341.3077069612, "Y"=530222.2638406174}, {"X"=175341.3464592256, "Y"=530222.3143336911}, {"X"=175341.38514233282, "Y"=530222.3636039045}, {"X"=175341.42348113446, "Y"=530222.4123623798}, {"X"=175341.4619506573, "Y"=530222.4606942837}, {"X"=175341.500862789, "Y"=530222.5080282264}, {"X"=175341.53989545174, "Y"=530222.5556858942}, {"X"=175341.57855971582, "Y"=530222.6045743736}, {"X"=175341.61733350207, "Y"=530222.6548576218}, {"X"=175341.65613315726, "Y"=530222.7061030421}, {"X"=175341.69501567204, "Y"=530222.7578132504}, {"X"=175341.7343073941, "Y"=530222.8095144829}, {"X"=175341.77426430586, "Y"=530222.8600028963}, {"X"=175341.81392813384, "Y"=530222.9102291381}, {"X"=175341.85343851932, "Y"=530222.9594858147}, {"X"=175341.89225202618, "Y"=530223.0088222381}, {"X"=175341.93099129558, "Y"=530223.0579147108}, {"X"=175341.96965254052, "Y"=530223.1075823216}, {"X"=175342.0079390977, "Y"=530223.1578514714}, {"X"=175342.04531629087, "Y"=530223.208234289}, {"X"=175342.0823620307, "Y"=530223.2582584881}, {"X"=175342.12036757922, "Y"=530223.3069524673}, {"X"=175342.15868380744, "Y"=530223.3555689492}, {"X"=175342.19669862968, "Y"=530223.4053061692}, {"X"=175342.235050533, "Y"=530223.455206654}, {"X"=175342.2738534825, "Y"=530223.5063710476}, {"X"=175342.31314116152, "Y"=530223.5582054758}, {"X"=175342.35286638304, "Y"=530223.6106301709}, {"X"=175342.39277461008, "Y"=530223.6626336892}, {"X"=175342.43220801378, "Y"=530223.7146241793}, {"X"=175342.47159401196, "Y"=530223.7661575475}, {"X"=175342.51108410227, "Y"=530223.8175463284}, {"X"=175342.55094774097, "Y"=530223.869450092}, {"X"=175342.5912302505, "Y"=530223.9216189857}, {"X"=175342.63127412286, "Y"=530223.9742658229}, {"X"=175342.67080800404, "Y"=530224.0272881878}, {"X"=175342.71031867288, "Y"=530224.0796480348}, {"X"=175342.74951846778, "Y"=530224.1317202356}, {"X"=175342.78877232302, "Y"=530224.1828999498}, {"X"=175342.82772654106, "Y"=530224.2342991909}, {"X"=175342.86694903608, "Y"=530224.2847575897}, {"X"=175342.90560732182, "Y"=530224.3358291847}, {"X"=175342.94384633898, "Y"=530224.3871017921}, {"X"=175342.9820561291, "Y"=530224.4380759329}, {"X"=175343.02040845525, "Y"=530224.4887244644}, {"X"=175343.05860425235, "Y"=530224.539158146}, {"X"=175343.09711823752, "Y"=530224.5899571424}, {"X"=175343.1359562095, "Y"=530224.6415875782}, {"X"=175343.17549843973, "Y"=530224.6935377966}, {"X"=175343.21551242692, "Y"=530224.7456653102}, {"X"=175343.25560978387, "Y"=530224.7972276604}, {"X"=175343.29504013137, "Y"=530224.849386863}, {"X"=175343.3341498303, "Y"=530224.9012462393}, {"X"=175343.37274251977, "Y"=530224.9538052416}, {"X"=175343.41201237464, "Y"=530225.0068095207}, {"X"=175343.451815017, "Y"=530225.0602606118}, {"X"=175343.49195184934, "Y"=530225.1131957419}, {"X"=175343.53112082684, "Y"=530225.1662347257}, {"X"=175343.56961757506, "Y"=530225.219001554}, {"X"=175343.6080597585, "Y"=530225.2706864333}, {"X"=175343.64636462432, "Y"=530225.3217635131}, {"X"=175343.68403406208, "Y"=530225.3727314826}, {"X"=175343.7218600944, "Y"=530225.4236357275}, {"X"=175343.7595005975, "Y"=530225.4756059833}, {"X"=175343.79804115012, "Y"=530225.5279087643}, {"X"=175343.8375512105, "Y"=530225.5809689405}, {"X"=175343.87768913654, "Y"=530225.634275872}, {"X"=175343.917179842, "Y"=530225.6888821401}, {"X"=175343.95703650004, "Y"=530225.7435317221}, {"X"=175343.99699233004, "Y"=530225.7993696701}, {"X"=175344.0379195635, "Y"=530225.8560071833}, {"X"=175344.07954486008, "Y"=530225.9129678269}, {"X"=175344.1215070291, "Y"=530225.9700218146}, {"X"=175344.16306955542, "Y"=530226.0270237095}, {"X"=175344.20444305483, "Y"=530226.0836044145}, {"X"=175344.2454281164, "Y"=530226.140028664}, {"X"=175344.2863313288, "Y"=530226.1963310726}, {"X"=175344.32693259235, "Y"=530226.2520683417}, {"X"=175344.3668732474, "Y"=530226.3081693741}, {"X"=175344.40610914843, "Y"=530226.3646831337}, {"X"=175344.44565920217, "Y"=530226.4204934239}, {"X"=175344.48556397823, "Y"=530226.4755424161}, {"X"=175344.52579878274, "Y"=530226.5292641538}, {"X"=175344.56470778922, "Y"=530226.5830608321}, {"X"=175344.60305079306, "Y"=530226.6368625081}, {"X"=175344.64138657736, "Y"=530226.6909194754}, {"X"=175344.6803523717, "Y"=530226.7450500538}, {"X"=175344.7192578378, "Y"=530226.8000498302}, {"X"=175344.75917082647, "Y"=530226.8551809292}, {"X"=175344.79916464357, "Y"=530226.9115892368}, {"X"=175344.83981818473, "Y"=530226.9691365355}, {"X"=175344.88087487346, "Y"=530227.0279256878}, {"X"=175344.92272513863, "Y"=530227.0869855267}, {"X"=175344.96484817393, "Y"=530227.1460290228}, {"X"=175345.00702341314, "Y"=530227.2047527262}, {"X"=175345.04837276042, "Y"=530227.2636608795}, {"X"=175345.08951531787, "Y"=530227.322132361}, {"X"=175345.13091765594, "Y"=530227.3797862194}, {"X"=175345.17261180005, "Y"=530227.4369697464}, {"X"=175345.2138841165, "Y"=530227.4943875886}, {"X"=175345.25474182, "Y"=530227.5523837806}, {"X"=175345.2953319248, "Y"=530227.6103496855}, {"X"=175345.33608077082, "Y"=530227.6677768407}, {"X"=175345.3767031518, "Y"=530227.7246727465}, {"X"=175345.41711203125, "Y"=530227.7815592935}, {"X"=175345.45734774778, "Y"=530227.8385984013}, {"X"=175345.49814907316, "Y"=530227.8961008744}, {"X"=175345.53987397553, "Y"=530227.9535040656}, {"X"=175345.58270584818, "Y"=530228.0105188708}, {"X"=175345.62524984934, "Y"=530228.0681371794}, {"X"=175345.66747818922, "Y"=530228.1265477482}, {"X"=175345.70959393718, "Y"=530228.1852261261}, {"X"=175345.7526580195, "Y"=530228.2440892733}, {"X"=175345.79605483665, "Y"=530228.3031445545}, {"X"=175345.8397833751, "Y"=530228.362049028}, {"X"=175345.8829142793, "Y"=530228.4219463692}, {"X"=175345.92626609065, "Y"=530228.4816599311}, {"X"=175345.96973678764, "Y"=530228.5405385285}, {"X"=175346.0128790672, "Y"=530228.5985868099}, {"X"=175346.05557086875, "Y"=530228.6564643917}, {"X"=175346.09855932498, "Y"=530228.7140148013}, {"X"=175346.14169494555, "Y"=530228.7716069507}, {"X"=175346.18538720495, "Y"=530228.8284227776}, {"X"=175346.2289090404, "Y"=530228.8851192427}, {"X"=175346.27231195508, "Y"=530228.9411379342}, {"X"=175346.31467855422, "Y"=530228.9977745438}, {"X"=175346.3565197893, "Y"=530229.0540797464}, {"X"=175346.398209656, "Y"=530229.1098182551}, {"X"=175346.44036334916, "Y"=530229.1648461967}, {"X"=175346.48222626268, "Y"=530229.2206929632}, {"X"=175346.5240881895, "Y"=530229.2768060985}, {"X"=175346.56605635298, "Y"=530229.3332008257}, {"X"=175346.60913138627, "Y"=530229.3894735328}, {"X"=175346.65260054462, "Y"=530229.4460303147}, {"X"=175346.6961474528, "Y"=530229.5031207076}, {"X"=175346.73861139643, "Y"=530229.5606304918}, {"X"=175346.78057418144, "Y"=530229.6182061245}, {"X"=175346.8221392308, "Y"=530229.6754743905}, {"X"=175346.8638107502, "Y"=530229.7325026138}, {"X"=175346.90517967637, "Y"=530229.789648263}, {"X"=175346.94734387382, "Y"=530229.8467382959}, {"X"=175346.99017519283, "Y"=530229.9032714318}, {"X"=175347.03319368736, "Y"=530229.9604987887}, {"X"=175347.07558367634, "Y"=530230.0181630625}, {"X"=175347.1179610232, "Y"=530230.0760460165}, {"X"=175347.16041506414, "Y"=530230.1341029915}, {"X"=175347.20272800326, "Y"=530230.1926742499}, {"X"=175347.24512683423, "Y"=530230.2515349273}, {"X"=175347.2874182252, "Y"=530230.3109086764}, {"X"=175347.3299874161, "Y"=530230.3695679661}, {"X"=175347.37305761402, "Y"=530230.4275088108}, {"X"=175347.41586943413, "Y"=530230.4849409934}, {"X"=175347.45826517747, "Y"=530230.5418549861}, {"X"=175347.50003243302, "Y"=530230.5983091341}, {"X"=175347.54152667837, "Y"=530230.6550004845}, {"X"=175347.5828384125, "Y"=530230.7116779468}, {"X"=175347.62513317316, "Y"=530230.7676899249}, {"X"=175347.66725613666, "Y"=530230.8237168362}, {"X"=175347.70895552073, "Y"=530230.8796850655}, {"X"=175347.75047259853, "Y"=530230.936010097}, {"X"=175347.79224858, "Y"=530230.992420933}, {"X"=175347.83379821095, "Y"=530231.0501731497}, {"X"=175347.87598747012, "Y"=530231.1085583183}, {"X"=175347.91865063147, "Y"=530231.1672461922}, {"X"=175347.96190239483, "Y"=530231.2254839465}, {"X"=175348.0049063384, "Y"=530231.2837890219}, {"X"=175348.04776506487, "Y"=530231.3412110822}, {"X"=175348.09002578325, "Y"=530231.3988968299}, {"X"=175348.1320544484, "Y"=530231.4565921396}, {"X"=175348.17388105046, "Y"=530231.5145510836}, {"X"=175348.2155488722, "Y"=530231.5718334815}, {"X"=175348.25715479362, "Y"=530231.6288519169}, {"X"=175348.298702659, "Y"=530231.6857062625}, {"X"=175348.34000642208, "Y"=530231.7423881912}, {"X"=175348.38131569765, "Y"=530231.7988370324}, {"X"=175348.42291422226, "Y"=530231.8557500527}, {"X"=175348.4651085602, "Y"=530231.9128555425}, {"X"=175348.5074611014, "Y"=530231.9701425808}, {"X"=175348.54977016072, "Y"=530232.0277038846}, {"X"=175348.59204602803, "Y"=530232.085123225}, {"X"=175348.63413675412, "Y"=530232.1425386709}, {"X"=175348.6759034338, "Y"=530232.200305787}, {"X"=175348.71787818449, "Y"=530232.2589446416}, {"X"=175348.76045198838, "Y"=530232.317371966}, {"X"=175348.80372661783, "Y"=530232.3755574945}, {"X"=175348.8467706997, "Y"=530232.4330600277}, {"X"=175348.88973412907, "Y"=530232.4902464917}, {"X"=175348.9325830176, "Y"=530232.5467385219}, {"X"=175348.97525145314, "Y"=530232.6036150943}, {"X"=175349.01743876605, "Y"=530232.6613454565}, {"X"=175349.05979153828, "Y"=530232.719614725}, {"X"=175349.1024098835, "Y"=530232.7775280537}, {"X"=175349.1453880101, "Y"=530232.8351950453}, {"X"=175349.18802687485, "Y"=530232.8922581619}, {"X"=175349.23083361104, "Y"=530232.9488757306}, {"X"=175349.2737960797, "Y"=530233.0057381197}, {"X"=175349.31699101478, "Y"=530233.0627330062}, {"X"=175349.35974836414, "Y"=530233.1203262894}, {"X"=175349.40281906206, "Y"=530233.1778453963}, {"X"=175349.44570093186, "Y"=530233.2353117875}, {"X"=175349.4887297444, "Y"=530233.2927455591}, {"X"=175349.53150355406, "Y"=530233.3505141508}, {"X"=175349.5747305128, "Y"=530233.4081582131}, {"X"=175349.61876782076, "Y"=530233.4660540435}, {"X"=175349.66334610982, "Y"=530233.5235709278}, {"X"=175349.70725425257, "Y"=530233.5815204117}, {"X"=175349.7504956164, "Y"=530233.639544004}, {"X"=175349.79353860093, "Y"=530233.6972796193}, {"X"=175349.83754390068, "Y"=530233.7539336112}, {"X"=175349.88171600256, "Y"=530233.8106814525}, {"X"=175349.92563081637, "Y"=530233.8675898704}, {"X"=175349.96906826223, "Y"=530233.9251234373}, {"X"=175350.01293208322, "Y"=530233.9821629709}, {"X"=175350.05650620023, "Y"=530234.0394841522}, {"X"=175350.09989550654, "Y"=530234.096613872}, {"X"=175350.14314725774, "Y"=530234.1536552103}, {"X"=175350.18660337463, "Y"=530234.2106127074}, {"X"=175350.2305396156, "Y"=530234.2675798872}, {"X"=175350.2749188809, "Y"=530234.3239919407}, {"X"=175350.31926038675, "Y"=530234.3805162015}, {"X"=175350.36325309795, "Y"=530234.4371080835}, {"X"=175350.40650135832, "Y"=530234.4938686392}, {"X"=175350.44973874703, "Y"=530234.5505470965}, {"X"=175350.49322314374, "Y"=530234.6074834237}, {"X"=175350.5372465261, "Y"=530234.6645657729}, {"X"=175350.58161553548, "Y"=530234.7214062652}, {"X"=175350.62636864078, "Y"=530234.7781335282}, {"X"=175350.67098936674, "Y"=530234.8347268899}, {"X"=175350.71522448817, "Y"=530234.8915222726}, {"X"=175350.75861984972, "Y"=530234.9483045933}, {"X"=175350.80163544806, "Y"=530235.0051679431}, {"X"=175350.8455027871, "Y"=530235.061300714}, {"X"=175350.88993979365, "Y"=530235.1168702191}, {"X"=175350.93419405032, "Y"=530235.1720451514}, {"X"=175350.97797018028, "Y"=530235.2272858657}, {"X"=175351.0211706906, "Y"=530235.2819733487}, {"X"=175351.06420086315, "Y"=530235.3368710969}, {"X"=175351.1069546017, "Y"=530235.391745242}, {"X"=175351.14969397328, "Y"=530235.4471543846}, {"X"=175351.19290508452, "Y"=530235.5030349332}, {"X"=175351.23708086298, "Y"=530235.5592333905}, {"X"=175351.28094664667, "Y"=530235.6163428451}, {"X"=175351.32507018273, "Y"=530235.6737500923}, {"X"=175351.36946815113, "Y"=530235.7311032579}, {"X"=175351.4141272058, "Y"=530235.7883812926}, {"X"=175351.45875193508, "Y"=530235.845434128}, {"X"=175351.5033432786, "Y"=530235.9016790844}, {"X"=175351.5477972615, "Y"=530235.9573007046}, {"X"=175351.5920627689, "Y"=530236.0123890406}, {"X"=175351.63490704828, "Y"=530236.0676302855}, {"X"=175351.67720670445, "Y"=530236.1229175301}, {"X"=175351.71963278952, "Y"=530236.1781233831}, {"X"=175351.76294240737, "Y"=530236.2322667169}, {"X"=175351.80625901482, "Y"=530236.2860770716}, {"X"=175351.84902049394, "Y"=530236.3393729797}, {"X"=175351.89089530785, "Y"=530236.3929711628}, {"X"=175351.9331973055, "Y"=530236.4457479022}, {"X"=175351.97514771618, "Y"=530236.498248212}, {"X"=175352.01617310618, "Y"=530236.5512595625}, {"X"=175352.05664432573, "Y"=530236.6049850797}, {"X"=175352.09796583082, "Y"=530236.6580865675}, {"X"=175352.13995707338, "Y"=530236.7103159536}, {"X"=175352.18166292325, "Y"=530236.7621876963}, {"X"=175352.22252090828, "Y"=530236.813099689}, {"X"=175352.26255605364, "Y"=530236.8637288735}, {"X"=175352.30208352584, "Y"=530236.9137169486}, {"X"=175352.34150491114, "Y"=530236.9634744846}, {"X"=175352.38042420865, "Y"=530237.0135842154}, {"X"=175352.4199305173, "Y"=530237.0639053108}, {"X"=175352.45956587067, "Y"=530237.114131686}, {"X"=175352.49899166732, "Y"=530237.1641844318}, {"X"=175352.53829575534, "Y"=530237.2141165627}, {"X"=175352.5774806659, "Y"=530237.2632843519}, {"X"=175352.6156511215, "Y"=530237.3132742075}, {"X"=175352.6533883326, "Y"=530237.3629312733}, {"X"=175352.6910130333, "Y"=530237.4119815769}, {"X"=175352.72911552244, "Y"=530237.4611514483}, {"X"=175352.7674107072, "Y"=530237.5110854433}, {"X"=175352.80628102296, "Y"=530237.5626092828}, {"X"=175352.84566256969, "Y"=530237.6153813166}, {"X"=175352.886305737, "Y"=530237.6688455134}, {"X"=175352.92686425932, "Y"=530237.7224420327}, {"X"=175352.96628213656, "Y"=530237.776421486}, {"X"=175353.00479581486, "Y"=530237.8295612222}, {"X"=175353.04309125987, "Y"=530237.8813875283}, {"X"=175353.0805856114, "Y"=530237.9321951261}, {"X"=175353.1178263727, "Y"=530237.9820145867}, {"X"=175353.15486826623, "Y"=530238.031681473}, {"X"=175353.19223656916, "Y"=530238.0808956837}, {"X"=175353.22936573613, "Y"=530238.1307199139}, {"X"=175353.26626025818, "Y"=530238.1808755734}, {"X"=175353.3027933256, "Y"=530238.2313119823}, {"X"=175353.33960005036, "Y"=530238.2823335917}, {"X"=175353.37707444988, "Y"=530238.3338859645}, {"X"=175353.41547161504, "Y"=530238.386566564}, {"X"=175353.45446338505, "Y"=530238.4399313043}, {"X"=175353.49378934092, "Y"=530238.4939798436}, {"X"=175353.53226842728, "Y"=530238.5480086806}, {"X"=175353.57047974097, "Y"=530238.6019472994}, {"X"=175353.60875617847, "Y"=530238.6557414449}, {"X"=175353.6469764394, "Y"=530238.7094103412}, {"X"=175353.68457545002, "Y"=530238.7638723999}, {"X"=175353.72234228044, "Y"=530238.8184738057}, {"X"=175353.76045086328, "Y"=530238.8730198212}, {"X"=175353.79898426452, "Y"=530238.9271461678}, {"X"=175353.8375490814, "Y"=530238.9808107199}, {"X"=175353.8752460613, "Y"=530239.0342536401}, {"X"=175353.91189012938, "Y"=530239.0874910104}, {"X"=175353.94910051365, "Y"=530239.1393293964}, {"X"=175353.98627210603, "Y"=530239.1909281688}, {"X"=175354.02308637538, "Y"=530239.2430096754}, {"X"=175354.05967783305, "Y"=530239.2955291213}, {"X"=175354.09668178417, "Y"=530239.3488542204}, {"X"=175354.1341990515, "Y"=530239.4023320772}, {"X"=175354.17198692198, "Y"=530239.4562597376}, {"X"=175354.20951566947, "Y"=530239.5106276667}, {"X"=175354.24727854424, "Y"=530239.5653911263}, {"X"=175354.28528886437, "Y"=530239.6202604033}, {"X"=175354.3236916914, "Y"=530239.6751662572}, {"X"=175354.36217982642, "Y"=530239.7301650902}, {"X"=175354.401261916, "Y"=530239.784725996}, {"X"=175354.4399844256, "Y"=530239.8399039346}, {"X"=175354.47800392206, "Y"=530239.8951827234}, {"X"=175354.51573281956, "Y"=530239.9501405099}, {"X"=175354.55374814585, "Y"=530240.0043061222}, {"X"=175354.5920931261, "Y"=530240.0585195966}, {"X"=175354.6307848023, "Y"=530240.1125533618}, {"X"=175354.66938268108, "Y"=530240.1672211337}, {"X"=175354.70835670453, "Y"=530240.22178347}, {"X"=175354.74747454954, "Y"=530240.2767560309}, {"X"=175354.78668856682, "Y"=530240.3322011083}, {"X"=175354.82573295297, "Y"=530240.3880961786}, {"X"=175354.86442117963, "Y"=530240.4448679785}, {"X"=175354.90385480528, "Y"=530240.5017940709}, {"X"=175354.9438868584, "Y"=530240.5585985357}, {"X"=175354.98450460396, "Y"=530240.6151670938}, {"X"=175355.02560184867, "Y"=530240.6712336912}, {"X"=175355.0663030908, "Y"=530240.7269795968}, {"X"=175355.10590519384, "Y"=530240.7830661403}, {"X"=175355.1451417851, "Y"=530240.8386587655}, {"X"=175355.1843346686, "Y"=530240.8944490728}, {"X"=175355.22404374706, "Y"=530240.9501668296}, {"X"=175355.2643191493, "Y"=530241.0056886901}, {"X"=175355.30494895973, "Y"=530241.0609420296}, {"X"=175355.34536480953, "Y"=530241.1163314045}, {"X"=175355.38549545314, "Y"=530241.1717260601}, {"X"=175355.42590157175, "Y"=530241.2271199028}, {"X"=175355.466450924, "Y"=530241.2827253059}, {"X"=175355.50749417936, "Y"=530241.3382071704}, {"X"=175355.54871472975, "Y"=530241.3943377783}, {"X"=175355.5905385754, "Y"=530241.4498939218}, {"X"=175355.6317120192, "Y"=530241.5056695165}, {"X"=175355.6725872653, "Y"=530241.5612506543}, {"X"=175355.7131346146, "Y"=530241.6170791457}, {"X"=175355.7536999294, "Y"=530241.6726922737}, {"X"=175355.79431457655, "Y"=530241.7288135714}, {"X"=175355.83564892667, "Y"=530241.7844865855}, {"X"=175355.87750007684, "Y"=530241.8402923684}, {"X"=175355.9195047443, "Y"=530241.8958912657}, {"X"=175355.96087904507, "Y"=530241.9515952377}, {"X"=175356.0021839649, "Y"=530242.0072017458}, {"X"=175356.04336760036, "Y"=530242.0628308104}, {"X"=175356.08446281333, "Y"=530242.1185134072}, {"X"=175356.1253711881, "Y"=530242.1742165342}, {"X"=175356.16642529293, "Y"=530242.2294763982}, {"X"=175356.20768692662, "Y"=530242.2839210114}, {"X"=175356.24861907747, "Y"=530242.3386751397}, {"X"=175356.28909854963, "Y"=530242.3934161742}, {"X"=175356.3297216975, "Y"=530242.4482167154}, {"X"=175356.37073719004, "Y"=530242.5026975726}, {"X"=175356.4121149016, "Y"=530242.5571573845}, {"X"=175356.45343968744, "Y"=530242.6113920517}, {"X"=175356.4948522827, "Y"=530242.6656653044}, {"X"=175356.53583169985, "Y"=530242.7208310526}, {"X"=175356.57724413514, "Y"=530242.7765537826}, {"X"=175356.61908518994, "Y"=530242.8331442699}, {"X"=175356.66122786675, "Y"=530242.8895895861}, {"X"=175356.7031677672, "Y"=530242.9460588078}, {"X"=175356.74520092676, "Y"=530243.0017108984}, {"X"=175356.78699071577, "Y"=530243.0568376329}, {"X"=175356.82860514967, "Y"=530243.1110725575}, {"X"=175356.86955351502, "Y"=530243.1650197727}, {"X"=175356.90969446828, "Y"=530243.2182091132}, {"X"=175356.9490777895, "Y"=530243.2712996902}, {"X"=175356.98857629084, "Y"=530243.3234998218}, {"X"=175357.02793550797, "Y"=530243.375025569}, {"X"=175357.06710013995, "Y"=530243.4266473373}, {"X"=175357.10620575276, "Y"=530243.4780817132}, {"X"=175357.14540980468, "Y"=530243.5298554179}, {"X"=175357.18500684414, "Y"=530243.5818288475}, {"X"=175357.2246604417, "Y"=530243.6349596942}, {"X"=175357.2641467288, "Y"=530243.6890266448}, {"X"=175357.30388953027, "Y"=530243.7438730717}, {"X"=175357.34434687858, "Y"=530243.7989260455}, {"X"=175357.38561276108, "Y"=530243.853314052}, {"X"=175357.42714635562, "Y"=530243.9080741812}, {"X"=175357.46842059385, "Y"=530243.9631946698}, {"X"=175357.50957774406, "Y"=530244.0191612169}, {"X"=175357.55071779378, "Y"=530244.0753364675}, {"X"=175357.5918336218, "Y"=530244.1320090053}, {"X"=175357.63331725454, "Y"=530244.1881499484}, {"X"=175357.6750473695, "Y"=530244.2440715226}, {"X"=175357.7166139784, "Y"=530244.2995152301}, {"X"=175357.75781324354, "Y"=530244.3550454788}, {"X"=175357.79876509352, "Y"=530244.4101791265}, {"X"=175357.8395200305, "Y"=530244.4652223483}, {"X"=175357.88012770392, "Y"=530244.5204901953}, {"X"=175357.92098501846, "Y"=530244.5757073621}, {"X"=175357.96204256182, "Y"=530244.6303379341}, {"X"=175358.0031356214, "Y"=530244.6843968236}, {"X"=175358.04383856695, "Y"=530244.7389307731}, {"X"=175358.08452646548, "Y"=530244.7931695447}, {"X"=175358.12566475326, "Y"=530244.8472460592}, {"X"=175358.16694392514, "Y"=530244.9013388081}, {"X"=175358.20819046954, "Y"=530244.9557823667}, {"X"=175358.2494700914, "Y"=530245.0103279366}, {"X"=175358.29098381952, "Y"=530245.064361171}, {"X"=175358.33216177375, "Y"=530245.118073536}, {"X"=175358.3732513863, "Y"=530245.1718660723}, {"X"=175358.41425988183, "Y"=530245.2263869141}, {"X"=175358.45530746563, "Y"=530245.2806457151}, {"X"=175358.4961279473, "Y"=530245.3353901925}, {"X"=175358.53755439995, "Y"=530245.389565749}, {"X"=175358.57880946694, "Y"=530245.4429948742}, {"X"=175358.6194754227, "Y"=530245.4955001123}, {"X"=175358.65923557561, "Y"=530245.5475241211}, {"X"=175358.6986810228, "Y"=530245.5985601745}, {"X"=175358.73818095252, "Y"=530245.6497481184}, {"X"=175358.77788761366, "Y"=530245.7016557507}, {"X"=175358.81772277673, "Y"=530245.7538848643}, {"X"=175358.8581828618, "Y"=530245.8068668401}, {"X"=175358.89923729494, "Y"=530245.8601456174}, {"X"=175358.94051532645, "Y"=530245.9144559056}, {"X"=175358.9816894016, "Y"=530245.9692592768}, {"X"=175359.02267067126, "Y"=530246.024462766}, {"X"=175359.06317469152, "Y"=530246.0791293798}, {"X"=175359.10328494103, "Y"=530246.1330302408}, {"X"=175359.1426311365, "Y"=530246.1864572257}, {"X"=175359.18170182902, "Y"=530246.2389749364}, {"X"=175359.22067294916, "Y"=530246.2913686386}, {"X"=175359.26036426862, "Y"=530246.3431819814}, {"X"=175359.3002206982, "Y"=530246.3951147026}, {"X"=175359.33957727332, "Y"=530246.4472564398}, {"X"=175359.37847526275, "Y"=530246.4997835399}, {"X"=175359.41736539445, "Y"=530246.5517468553}, {"X"=175359.45611866727, "Y"=530246.6035596343}, {"X"=175359.49516651212, "Y"=530246.6552394703}, {"X"=175359.534532394, "Y"=530246.7066320259}, {"X"=175359.5738779074, "Y"=530246.7589269583}, {"X"=175359.61317105513, "Y"=530246.8120899559}, {"X"=175359.65284148513, "Y"=530246.8658334052}, {"X"=175359.6924238613, "Y"=530246.9197546942}, {"X"=175359.7321189642, "Y"=530246.9737555607}, {"X"=175359.7722131497, "Y"=530247.0267175318}, {"X"=175359.812302406, "Y"=530247.078607394}, {"X"=175359.8517182705, "Y"=530247.1301296569}, {"X"=175359.89077924602, "Y"=530247.180555317}, {"X"=175359.9290297936, "Y"=530247.2313018942}, {"X"=175359.96678072223, "Y"=530247.2823373973}, {"X"=175360.00470898786, "Y"=530247.3328329864}, {"X"=175360.04301417153, "Y"=530247.3831842932}, {"X"=175360.0812444498, "Y"=530247.4339664449}, {"X"=175360.11974357752, "Y"=530247.4852061785}, {"X"=175360.15889532102, "Y"=530247.5363762868}, {"X"=175360.19878413517, "Y"=530247.5878805108}, {"X"=175360.23892902656, "Y"=530247.6391142854}, {"X"=175360.278401387, "Y"=530247.6905731225}, {"X"=175360.31737113406, "Y"=530247.7419035878}, {"X"=175360.3562170554, "Y"=530247.7923964746}, {"X"=175360.39471564715, "Y"=530247.8425529867}, {"X"=175360.43373020628, "Y"=530247.8922584872}, {"X"=175360.47263689383, "Y"=530247.9426313309}, {"X"=175360.51171172748, "Y"=530247.9935541683}, {"X"=175360.55096069007, "Y"=530248.0452522838}, {"X"=175360.59049010673, "Y"=530248.0971371413}, {"X"=175360.63068016354, "Y"=530248.1486704462}, {"X"=175360.67107729564, "Y"=530248.2001354393}, {"X"=175360.71119287587, "Y"=530248.2510430022}, {"X"=175360.75040324742, "Y"=530248.3025725349}, {"X"=175360.78979999508, "Y"=530248.3545254847}, {"X"=175360.8304710297, "Y"=530248.4066589174}, {"X"=175360.87127768132, "Y"=530248.4591260182}, {"X"=175360.91191723972, "Y"=530248.5123017002}, {"X"=175360.9523743838, "Y"=530248.5657975603}, {"X"=175360.99262587648, "Y"=530248.618641429}, {"X"=175361.0330122471, "Y"=530248.6709654863}, {"X"=175361.0729788118, "Y"=530248.7224062232}, {"X"=175361.11191044463, "Y"=530248.7737323643}, {"X"=175361.1505965638, "Y"=530248.8241047515}, {"X"=175361.18968035345, "Y"=530248.8732595601}, {"X"=175361.22874977769, "Y"=530248.921748496}, {"X"=175361.26740235148, "Y"=530248.9697558712}, {"X"=175361.3060301731, "Y"=530249.0177799684}, {"X"=175361.34393528936, "Y"=530249.066737368}, {"X"=175361.38214647444, "Y"=530249.1170578811}, {"X"=175361.4216719192, "Y"=530249.1682002577}, {"X"=175361.46218246105, "Y"=530249.2199790122}, {"X"=175361.50222234274, "Y"=530249.2728556928}, {"X"=175361.54213471914, "Y"=530249.3257493963}, {"X"=175361.5823825225, "Y"=530249.3776443499}, {"X"=175361.62273221207, "Y"=530249.428344794}, {"X"=175361.6628429453, "Y"=530249.4785132093}, {"X"=175361.70243138418, "Y"=530249.528188167}, {"X"=175361.74098416534, "Y"=530249.578102579}, {"X"=175361.77956365625, "Y"=530249.6283642957}, {"X"=175361.81847626573, "Y"=530249.6783475681}, {"X"=175361.8581347175, "Y"=530249.7283353001}, {"X"=175361.8979152902, "Y"=530249.778284938}, {"X"=175361.93752073805, "Y"=530249.8283216615}, {"X"=175361.97688238163, "Y"=530249.8785866245}, {"X"=175362.0162104847, "Y"=530249.9285919806}, {"X"=175362.0553811717, "Y"=530249.978382486}, {"X"=175362.09459135542, "Y"=530250.0277489105}, {"X"=175362.1339222446, "Y"=530250.0774978804}, {"X"=175362.1736222086, "Y"=530250.1271469857}, {"X"=175362.21321350688, "Y"=530250.1768918592}, {"X"=175362.252683638, "Y"=530250.2270011243}, {"X"=175362.2924473459, "Y"=530250.2766389428}, {"X"=175362.33200780407, "Y"=530250.3264405108}, {"X"=175362.37099305278, "Y"=530250.376127239}, {"X"=175362.41009984864, "Y"=530250.4258801995}, {"X"=175362.44898119677, "Y"=530250.4751765631}, {"X"=175362.48782192072, "Y"=530250.52421334}, {"X"=175362.52699950442, "Y"=530250.5730404704}, {"X"=175362.5667985681, "Y"=530250.6220522263}, {"X"=175362.60660301094, "Y"=530250.6722892505}, {"X"=175362.64652048083, "Y"=530250.7230076215}, {"X"=175362.6858567776, "Y"=530250.7736921888}, {"X"=175362.7251310844, "Y"=530250.8240806081}, {"X"=175362.7639446701, "Y"=530250.8741296573}, {"X"=175362.8025109473, "Y"=530250.9235190699}, {"X"=175362.84085578495, "Y"=530250.9717071552}, {"X"=175362.87910314006, "Y"=530251.0198799929}, {"X"=175362.91751004552, "Y"=530251.0674885499}, {"X"=175362.95600635879, "Y"=530251.1153798591}, {"X"=175362.99435708468, "Y"=530251.1643636992}, {"X"=175363.0334184228, "Y"=530251.2137227969}, {"X"=175363.07259438004, "Y"=530251.2638029656}, {"X"=175363.11199823796, "Y"=530251.3139701424}, {"X"=175363.1513796253, "Y"=530251.364327171}, {"X"=175363.1906501197, "Y"=530251.4146268141}, {"X"=175363.22968945027, "Y"=530251.4646341368}, {"X"=175363.26866563145, "Y"=530251.5142531929}, {"X"=175363.3073697122, "Y"=530251.563214906}, {"X"=175363.34559084047, "Y"=530251.6127085537}, {"X"=175363.38380230192, "Y"=530251.6619292059}, {"X"=175363.42243679025, "Y"=530251.7104205436}, {"X"=175363.4610109799, "Y"=530251.7588898608}, {"X"=175363.49973307314, "Y"=530251.8073520857}, {"X"=175363.5383682305, "Y"=530251.8560709434}, {"X"=175363.57717002617, "Y"=530251.9048281554}, {"X"=175363.61560527026, "Y"=530251.9542412636}, {"X"=175363.65436447458, "Y"=530252.0032738473}, {"X"=175363.69337000587, "Y"=530252.0523334497}, {"X"=175363.7324087816, "Y"=530252.1018546579}, {"X"=175363.77137032332, "Y"=530252.1516169315}, {"X"=175363.81046026983, "Y"=530252.2025719273}, {"X"=175363.85010976103, "Y"=530252.253435373}, {"X"=175363.89048429485, "Y"=530252.3041590624}, {"X"=175363.9305881354, "Y"=530252.3547037531}, {"X"=175363.97065607106, "Y"=530252.4053872812}, {"X"=175364.0104260441, "Y"=530252.455955151}, {"X"=175364.05022246856, "Y"=530252.5055817852}, {"X"=175364.0895394326, "Y"=530252.5551210414}, {"X"=175364.12854528782, "Y"=530252.6042938508}, {"X"=175364.1669772529, "Y"=530252.6537979816}, {"X"=175364.2054922055, "Y"=530252.702908976}, {"X"=175364.24385568034, "Y"=530252.7514155437}, {"X"=175364.28218815473, "Y"=530252.799923314}, {"X"=175364.32078050665, "Y"=530252.848247191}, {"X"=175364.35987321084, "Y"=530252.8971334021}, {"X"=175364.39976063493, "Y"=530252.9472814032}, {"X"=175364.44051739766, "Y"=530252.9990649943}, {"X"=175364.48121062687, "Y"=530253.052132879}, {"X"=175364.5217449672, "Y"=530253.1050880281}, {"X"=175364.56172633727, "Y"=530253.1576607942}, {"X"=175364.60130530893, "Y"=530253.2095455242}, {"X"=175364.64039269785, "Y"=530253.2608368186}, {"X"=175364.67953891496, "Y"=530253.3116529188}, {"X"=175364.71831601113, "Y"=530253.3628541183}, {"X"=175364.75731318252, "Y"=530253.4135907482}, {"X"=175364.79603092565, "Y"=530253.4635879273}, {"X"=175364.8341888009, "Y"=530253.5129652326}, {"X"=175364.8714835971, "Y"=530253.5616292221}, {"X"=175364.90849024183, "Y"=530253.6105027163}, {"X"=175364.94563348373, "Y"=530253.6594390685}, {"X"=175364.98314331504, "Y"=530253.7089359304}, {"X"=175365.02100005752, "Y"=530253.7595272006}, {"X"=175365.05918145005, "Y"=530253.8114759818}, {"X"=175365.09803261896, "Y"=530253.864670273}, {"X"=175365.1369677881, "Y"=530253.9178143732}, {"X"=175365.175450904, "Y"=530253.9711551395}, {"X"=175365.2146263419, "Y"=530254.0234727964}, {"X"=175365.25404981908, "Y"=530254.0748962869}, {"X"=175365.29313406267, "Y"=530254.1257247813}, {"X"=175365.3311370293, "Y"=530254.1760414864}, {"X"=175365.36840857498, "Y"=530254.2258364942}, {"X"=175365.40494955413, "Y"=530254.2744971587}, {"X"=175365.44107322232, "Y"=530254.3225197739}, {"X"=175365.4766030218, "Y"=530254.3695064213}, {"X"=175365.51182505823, "Y"=530254.4166593428}, {"X"=175365.54752247653, "Y"=530254.4640172995}, {"X"=175365.58419388309, "Y"=530254.5115499632}, {"X"=175365.62093701866, "Y"=530254.5602788435}, {"X"=175365.65774631436, "Y"=530254.6098177265}, {"X"=175365.6950449408, "Y"=530254.6597857933}, {"X"=175365.73257001908, "Y"=530254.7099496393}, {"X"=175365.76995592058, "Y"=530254.7600772697}, {"X"=175365.80677752316, "Y"=530254.8101854757}, {"X"=175365.84416599848, "Y"=530254.8596838082}, {"X"=175365.88176222175, "Y"=530254.9096443404}, {"X"=175365.91953173553, "Y"=530254.9594944854}, {"X"=175365.9574402241, "Y"=530255.0090134849}, {"X"=175365.99470143978, "Y"=530255.0589117429}, {"X"=175366.03154062154, "Y"=530255.1089755029}, {"X"=175366.0680535847, "Y"=530255.1592533174}, {"X"=175366.10490100825, "Y"=530255.2091083997}, {"X"=175366.1418778741, "Y"=530255.2596034913}, {"X"=175366.1794578632, "Y"=530255.3106683819}, {"X"=175366.2173681856, "Y"=530255.3620142048}, {"X"=175366.25529422174, "Y"=530255.4138827252}, {"X"=175366.29256422166, "Y"=530255.465561172}, {"X"=175366.3293060358, "Y"=530255.517452049}, {"X"=175366.36565792985, "Y"=530255.5689833704}, {"X"=175366.40203412157, "Y"=530255.6200418209}, {"X"=175366.4388502521, "Y"=530255.6703997643}, {"X"=175366.47596965497, "Y"=530255.7205714668}, {"X"=175366.51282475406, "Y"=530255.770928185}, {"X"=175366.5496163633, "Y"=530255.821080876}, {"X"=175366.58622919343, "Y"=530255.8712851491}, {"X"=175366.62272470424, "Y"=530255.9216551357}, {"X"=175366.65895272506, "Y"=530255.9726318942}, {"X"=175366.69602994501, "Y"=530256.0244207871}, {"X"=175366.73390271078, "Y"=530256.0771507177}, {"X"=175366.77233000507, "Y"=530256.1316958538}, {"X"=175366.81173351035, "Y"=530256.1868696233}, {"X"=175366.8519770966, "Y"=530256.2427678755}, {"X"=175366.8918884384, "Y"=530256.2989401333}, {"X"=175366.93135789846, "Y"=530256.3554544192}, {"X"=175366.9706897959, "Y"=530256.4115784413}, {"X"=175367.01058779864, "Y"=530256.4677340913}, {"X"=175367.05065983246, "Y"=530256.5246328339}, {"X"=175367.09101690596, "Y"=530256.5811689214}, {"X"=175367.1310731591, "Y"=530256.6375227704}, {"X"=175367.17083612958, "Y"=530256.6932448632}, {"X"=175367.21025581684, "Y"=530256.7481999461}, {"X"=175367.2492354851, "Y"=530256.8023261506}, {"X"=175367.287581066, "Y"=530256.8564975066}, {"X"=175367.32615449073, "Y"=530256.910735893}, {"X"=175367.3651370734, "Y"=530256.9652505389}, {"X"=175367.40405244404, "Y"=530257.0192004658}, {"X"=175367.44224889282, "Y"=530257.0729627243}, {"X"=175367.48063509667, "Y"=530257.1270928971}, {"X"=175367.5193307458, "Y"=530257.1810268238}, {"X"=175367.55835376275, "Y"=530257.2354370258}, {"X"=175367.59777806984, "Y"=530257.2904586872}, {"X"=175367.63832748993, "Y"=530257.3464415018}, {"X"=175367.67939942481, "Y"=530257.4029932447}, {"X"=175367.7207491782, "Y"=530257.4600391674}, {"X"=175367.7617005033, "Y"=530257.5171439771}, {"X"=175367.80307118673, "Y"=530257.5743796235}, {"X"=175367.84486851882, "Y"=530257.6312133558}, {"X"=175367.88690845872, "Y"=530257.6877145241}, {"X"=175367.92825091735, "Y"=530257.7446905482}, {"X"=175367.9699223432, "Y"=530257.8011817061}, {"X"=175368.01151293772, "Y"=530257.8572957474}, {"X"=175368.05314487906, "Y"=530257.9130123383}, {"X"=175368.09419173302, "Y"=530257.9685697247}, {"X"=175368.13502857919, "Y"=530258.0240999819}, {"X"=175368.17578947498, "Y"=530258.0794073816}, {"X"=175368.21706993572, "Y"=530258.1336810826}, {"X"=175368.2580036735, "Y"=530258.1878248417}, {"X"=175368.29871781138, "Y"=530258.2416928933}, {"X"=175368.33960146687, "Y"=530258.29567476}, {"X"=175368.38056272513, "Y"=530258.349538754}, {"X"=175368.42160467047, "Y"=530258.403431366}, {"X"=175368.46324653408, "Y"=530258.4574065608}, {"X"=175368.50493600065, "Y"=530258.5113039257}, {"X"=175368.546039586, "Y"=530258.5653739354}, {"X"=175368.58627301786, "Y"=530258.619636295}, {"X"=175368.62661766922, "Y"=530258.6737673621}, {"X"=175368.66737663423, "Y"=530258.7275187485}, {"X"=175368.707789486, "Y"=530258.7819492777}, {"X"=175368.74817281184, "Y"=530258.8368815499}, {"X"=175368.78905969212, "Y"=530258.8922607239}, {"X"=175368.83060171016, "Y"=530258.9472239888}, {"X"=175368.87236381875, "Y"=530259.0017271258}, {"X"=175368.91362172773, "Y"=530259.0555647215}, {"X"=175368.9541187612, "Y"=530259.1088041244}, {"X"=175368.99351905257, "Y"=530259.161693824}, {"X"=175369.03251394143, "Y"=530259.2140797316}, {"X"=175369.07165795774, "Y"=530259.2668725194}, {"X"=175369.1116919916, "Y"=530259.3202020752}, {"X"=175369.1522712206, "Y"=530259.3739828493}, {"X"=175369.19244677763, "Y"=530259.4275450595}, {"X"=175369.2315454748, "Y"=530259.4811925745}, {"X"=175369.27035327113, "Y"=530259.5341139864}, {"X"=175369.30912567972, "Y"=530259.5858479531}, {"X"=175369.34761534786, "Y"=530259.637222049}, {"X"=175369.38570391198, "Y"=530259.6883464997}, {"X"=175369.4236531108, "Y"=530259.7393714729}, {"X"=175369.4617789277, "Y"=530259.7896123657}, {"X"=175369.49993611278, "Y"=530259.8390751553}, {"X"=175369.53771359075, "Y"=530259.8880362958}, {"X"=175369.57511864332, "Y"=530259.9371627924}, {"X"=175369.61242632216, "Y"=530259.9872129811}, {"X"=175369.65026476423, "Y"=530260.0379253004}, {"X"=175369.68844804208, "Y"=530260.0899329198}, {"X"=175369.72774864096, "Y"=530260.1420593341}, {"X"=175369.76747697193, "Y"=530260.1944530737}, {"X"=175369.80690045215, "Y"=530260.2470996501}, {"X"=175369.84600582987, "Y"=530260.2994086567}, {"X"=175369.8855787249, "Y"=530260.3516585723}, {"X"=175369.92548969664, "Y"=530260.4038098247}, {"X"=175369.96521553188, "Y"=530260.4568606102}, {"X"=175370.0048233524, "Y"=530260.5098418208}, {"X"=175370.04435833584, "Y"=530260.5630540976}, {"X"=175370.08360233658, "Y"=530260.6155147478}, {"X"=175370.12268043496, "Y"=530260.6666828998}, {"X"=175370.161077391, "Y"=530260.7169574014}, {"X"=175370.1988345409, "Y"=530260.7665367983}, {"X"=175370.23621340372, "Y"=530260.8160973303}, {"X"=175370.2741603868, "Y"=530260.8651700723}, {"X"=175370.31198308783, "Y"=530260.9147526048}, {"X"=175370.3494809023, "Y"=530260.9653027819}, {"X"=175370.38678381703, "Y"=530261.0161443175}, {"X"=175370.42433720775, "Y"=530261.0678208391}, {"X"=175370.4626341092, "Y"=530261.1193120438}, {"X"=175370.50168795633, "Y"=530261.1715712609}, {"X"=175370.54076009642, "Y"=530261.2252288469}, {"X"=175370.58048902013, "Y"=530261.279631433}, {"X"=175370.62107124308, "Y"=530261.333832843}, {"X"=175370.66210860672, "Y"=530261.3879840766}, {"X"=175370.70264565348, "Y"=530261.4421856187}, {"X"=175370.74249817466, "Y"=530261.4961483381}, {"X"=175370.78169428193, "Y"=530261.5497933521}, {"X"=175370.82119589235, "Y"=530261.6028059552}, {"X"=175370.8604972166, "Y"=530261.6560855159}, {"X"=175370.89999125095, "Y"=530261.7092335463}, {"X"=175370.93876096676, "Y"=530261.7621650669}, {"X"=175370.97771263926, "Y"=530261.8146221417}, {"X"=175371.01739352918, "Y"=530261.8662513338}, {"X"=175371.057154059, "Y"=530261.9175528833}, {"X"=175371.09605709632, "Y"=530261.9691366423}, {"X"=175371.13461257404, "Y"=530262.0218090902}, {"X"=175371.17493162048, "Y"=530262.074476341}, {"X"=175371.2161687712, "Y"=530262.1281930344}, {"X"=175371.2574986481, "Y"=530262.1824155508}, {"X"=175371.29896848748, "Y"=530262.2372436394}, {"X"=175371.34017383057, "Y"=530262.2927928045}, {"X"=175371.38163837852, "Y"=530262.3479305593}, {"X"=175371.4233859332, "Y"=530262.4026168778}, {"X"=175371.4653806578, "Y"=530262.457616558}, {"X"=175371.50709616198, "Y"=530262.5134505647}, {"X"=175371.5492311775, "Y"=530262.5688660291}, {"X"=175371.59135206408, "Y"=530262.6242970738}, {"X"=175371.63361993022, "Y"=530262.6797065984}, {"X"=175371.67533013487, "Y"=530262.7352465111}, {"X"=175371.7166030467, "Y"=530262.7908820468}, {"X"=175371.7576439664, "Y"=530262.846846788}, {"X"=175371.79961031346, "Y"=530262.9018365643}, {"X"=175371.8417403082, "Y"=530262.9558502925}, {"X"=175371.88340146284, "Y"=530263.0091728515}, {"X"=175371.92439824372, "Y"=530263.0615795128}, {"X"=175371.96503316762, "Y"=530263.1135310883}, {"X"=175372.0052249805, "Y"=530263.1648058448}, {"X"=175372.04496494954, "Y"=530263.216047527}, {"X"=175372.08486382675, "Y"=530263.267409716}, {"X"=175372.12527531054, "Y"=530263.3195872516}, {"X"=175372.16591554228, "Y"=530263.3718373646}, {"X"=175372.20672269005, "Y"=530263.4245209418}, {"X"=175372.24767576595, "Y"=530263.4771275077}, {"X"=175372.28965336786, "Y"=530263.5290240761}, {"X"=175372.33110264182, "Y"=530263.5816868937}, {"X"=175372.3726853523, "Y"=530263.6348432075}, {"X"=175372.4151099726, "Y"=530263.6881424303}, {"X"=175372.45798269208, "Y"=530263.7411051576}, {"X"=175372.50007205043, "Y"=530263.7942555395}, {"X"=175372.5416247459, "Y"=530263.8474474571}, {"X"=175372.5829580622, "Y"=530263.9010406794}, {"X"=175372.62484024334, "Y"=530263.9542238587}, {"X"=175372.66669413337, "Y"=530264.0071252142}, {"X"=175372.70904192966, "Y"=530264.0599052535}, {"X"=175372.75097860975, "Y"=530264.112345775}, {"X"=175372.7924628684, "Y"=530264.1645578903}, {"X"=175372.8333104372, "Y"=530264.2162313784}, {"X"=175372.8738449646, "Y"=530264.2680833666}, {"X"=175372.91441410081, "Y"=530264.319957451}, {"X"=175372.9557862025, "Y"=530264.3719834397}, {"X"=175372.99767016945, "Y"=530264.4239701862}, {"X"=175373.03924414562, "Y"=530264.4765704875}, {"X"=175373.0804756962, "Y"=530264.529296102}, {"X"=175373.12245933426, "Y"=530264.5811404951}, {"X"=175373.1641074646, "Y"=530264.6327539145}, {"X"=175373.2048067197, "Y"=530264.6842968779}, {"X"=175373.245243158, "Y"=530264.7356275225}, {"X"=175373.28613031158, "Y"=530264.7872098872}, {"X"=175373.3268719919, "Y"=530264.8396239675}, {"X"=175373.36816244232, "Y"=530264.8921995794}, {"X"=175373.40948345076, "Y"=530264.9443233894}, {"X"=175373.45060314657, "Y"=530264.9963656624}, {"X"=175373.49133239881, "Y"=530265.0475689222}, {"X"=175373.53206551704, "Y"=530265.0985812743}, {"X"=175373.5723972954, "Y"=530265.1501674973}, {"X"=175373.6127379377, "Y"=530265.2029590018}, {"X"=175373.65307959612, "Y"=530265.2560956681}, {"X"=175373.6935509451, "Y"=530265.3090554855}, {"X"=175373.73412274377, "Y"=530265.3609340055}, {"X"=175373.7750503279, "Y"=530265.4118103823}, {"X"=175373.8156763603, "Y"=530265.4625544671}, {"X"=175373.85636513907, "Y"=530265.512649098}, {"X"=175373.8966237603, "Y"=530265.5631567544}, {"X"=175373.9368359794, "Y"=530265.6141495564}, {"X"=175373.97664394762, "Y"=530265.6659315486}, {"X"=175374.01652882574, "Y"=530265.7176611514}, {"X"=175374.0558253849, "Y"=530265.7696377665}, {"X"=175374.09546728528, "Y"=530265.8215756294}, {"X"=175374.1352996199, "Y"=530265.8735107117}, {"X"=175374.1753605969, "Y"=530265.9263862808}, {"X"=175374.21554098636, "Y"=530265.9792048966}, {"X"=175374.25634345112, "Y"=530266.0321115775}, {"X"=175374.29684755186, "Y"=530266.0847660915}, {"X"=175374.3370072678, "Y"=530266.1368822271}, {"X"=175374.37684985562, "Y"=530266.1883899836}, {"X"=175374.41664284474, "Y"=530266.2401997693}, {"X"=175374.45623583646, "Y"=530266.2926760602}, {"X"=175374.4957903801, "Y"=530266.3453322599}, {"X"=175374.53494277128, "Y"=530266.3985856391}, {"X"=175374.5738609444, "Y"=530266.4514124128}, {"X"=175374.61273645412, "Y"=530266.5035878264}, {"X"=175374.6511642197, "Y"=530266.5553183937}, {"X"=175374.68891586334, "Y"=530266.6066558418}, {"X"=175374.72739777548, "Y"=530266.6569223469}, {"X"=175374.7656299184, "Y"=530266.7065947026}, {"X"=175374.80313963493, "Y"=530266.7566920433}, {"X"=175374.8399778119, "Y"=530266.8064484142}, {"X"=175374.8766657008, "Y"=530266.8563062254}, {"X"=175374.91344849125, "Y"=530266.9059040511}, {"X"=175374.95023190015, "Y"=530266.9560135192}, {"X"=175374.98740198716, "Y"=530267.0068876502}, {"X"=175375.02601149524, "Y"=530267.0580716352}, {"X"=175375.06553802377, "Y"=530267.1114426706}, {"X"=175375.10591067414, "Y"=530267.1669876481}, {"X"=175375.146517546, "Y"=530267.2238637658}, {"X"=175375.1877406851, "Y"=530267.2809611515}, {"X"=175375.22830013547, "Y"=530267.3382780246}, {"X"=175375.26785239112, "Y"=530267.3949719046}, {"X"=175375.30721058228, "Y"=530267.4504355218}, {"X"=175375.34715167427, "Y"=530267.5053180757}, {"X"=175375.38706773933, "Y"=530267.5595225785}, {"X"=175375.4267418654, "Y"=530267.613685621}, {"X"=175375.46535510637, "Y"=530267.6676442431}, {"X"=175375.50396058234, "Y"=530267.7216716999}, {"X"=175375.54284507962, "Y"=530267.7750990131}, {"X"=175375.58147326022, "Y"=530267.8287157561}, {"X"=175375.61925587003, "Y"=530267.8830519565}, {"X"=175375.6576886122, "Y"=530267.9376803568}, {"X"=175375.69664500767, "Y"=530267.9926623688}, {"X"=175375.73603756493, "Y"=530268.0480681743}, {"X"=175375.77532893803, "Y"=530268.1040047903}, {"X"=175375.81435740308, "Y"=530268.1602995562}, {"X"=175375.85262212646, "Y"=530268.2171293042}, {"X"=175375.89158039243, "Y"=530268.2739503484}, {"X"=175375.93173150255, "Y"=530268.330970986}, {"X"=175375.97191079802, "Y"=530268.3882379278}, {"X"=175376.01228297348, "Y"=530268.4463333681}, {"X"=175376.05265943654, "Y"=530268.5043810724}, {"X"=175376.09293965067, "Y"=530268.562530056}, {"X"=175376.13402299516, "Y"=530268.6205878863}, {"X"=175376.17550761972, "Y"=530268.6789541855}, {"X"=175376.2171191087, "Y"=530268.7382901298}, {"X"=175376.25857909265, "Y"=530268.798215855}, {"X"=175376.30063365336, "Y"=530268.8576137554}, {"X"=175376.34250984906, "Y"=530268.9169023044}, {"X"=175376.38375533113, "Y"=530268.9761782852}, {"X"=175376.4239993277, "Y"=530269.0352652095}, {"X"=175376.46462206956, "Y"=530269.0942278227}, {"X"=175376.5061171255, "Y"=530269.1522278391}, {"X"=175376.5475091983, "Y"=530269.20984859}, {"X"=175376.58769639168, "Y"=530269.2676948581}, {"X"=175376.62757688668, "Y"=530269.3254665607}, {"X"=175376.667320457, "Y"=530269.3824628744}, {"X"=175376.70731428557, "Y"=530269.4393174993}, {"X"=175376.74719239495, "Y"=530269.495980459}, {"X"=175376.7866007532, "Y"=530269.5537480027}, {"X"=175376.82704140185, "Y"=530269.6116368113}, {"X"=175376.86867427992, "Y"=530269.6692157873}, {"X"=175376.91032201465, "Y"=530269.7264251373}, {"X"=175376.9512818232, "Y"=530269.7837452792}, {"X"=175376.99105095697, "Y"=530269.8410012267}, {"X"=175377.02996204546, "Y"=530269.8986514817}, {"X"=175377.06897030905, "Y"=530269.9562137703}, {"X"=175377.1089557823, "Y"=530270.0135423321}, {"X"=175377.14928842592, "Y"=530270.0708510028}, {"X"=175377.18985192844, "Y"=530270.1274475757}, {"X"=175377.2301206264, "Y"=530270.1834967455}, {"X"=175377.2706423454, "Y"=530270.2388393001}, {"X"=175377.31043959537, "Y"=530270.2942139549}, {"X"=175377.34961013673, "Y"=530270.3497336272}, {"X"=175377.38805029093, "Y"=530270.4062842885}, {"X"=175377.42698760645, "Y"=530270.4629167287}, {"X"=175377.4664671266, "Y"=530270.5195853052}, {"X"=175377.50645504915, "Y"=530270.5753411908}, {"X"=175377.5459466516, "Y"=530270.6313005314}, {"X"=175377.58575752817, "Y"=530270.6876951077}, {"X"=175377.62575899236, "Y"=530270.7447406121}, {"X"=175377.66585884744, "Y"=530270.8024117845}, {"X"=175377.70568216513, "Y"=530270.8603246126}, {"X"=175377.74558738028, "Y"=530270.9180740495}, {"X"=175377.7855966506, "Y"=530270.974763265}, {"X"=175377.82569728378, "Y"=530271.0302924092}, {"X"=175377.86556871625, "Y"=530271.084692392}, {"X"=175377.90532123862, "Y"=530271.1393202449}, {"X"=175377.94501325546, "Y"=530271.1944565923}, {"X"=175377.98486513883, "Y"=530271.2503405145}, {"X"=175378.02435570536, "Y"=530271.3062510273}, {"X"=175378.06409336728, "Y"=530271.3621497148}, {"X"=175378.103309077, "Y"=530271.4176703686}, {"X"=175378.14220560313, "Y"=530271.473087634}, {"X"=175378.1814429543, "Y"=530271.5284373041}, {"X"=175378.22134028416, "Y"=530271.5838127786}, {"X"=175378.26121354155, "Y"=530271.6397365938}, {"X"=175378.30082891998, "Y"=530271.695920876}, {"X"=175378.34050395305, "Y"=530271.7519096485}, {"X"=175378.38047696327, "Y"=530271.8074180826}, {"X"=175378.42039218737, "Y"=530271.8628545483}, {"X"=175378.46029272696, "Y"=530271.9181179173}, {"X"=175378.50024812756, "Y"=530271.973962691}, {"X"=175378.54103024217, "Y"=530272.0296030378}, {"X"=175378.58160302788, "Y"=530272.0854482147}, {"X"=175378.6219478474, "Y"=530272.1405826434}, {"X"=175378.66133265817, "Y"=530272.1948741865}, {"X"=175378.70041345863, "Y"=530272.2478991648}, {"X"=175378.73875308977, "Y"=530272.3003991435}, {"X"=175378.7769726777, "Y"=530272.3530437571}, {"X"=175378.81478900305, "Y"=530272.4059093122}, {"X"=175378.85344642977, "Y"=530272.4595459604}, {"X"=175378.8927827093, "Y"=530272.5129997034}, {"X"=175378.9328368426, "Y"=530272.5662793056}, {"X"=175378.97299077566, "Y"=530272.619159064}, {"X"=175379.01313879451, "Y"=530272.6724361693}, {"X"=175379.05281503018, "Y"=530272.7267301857}, {"X"=175379.09275090517, "Y"=530272.7819634884}, {"X"=175379.13273609988, "Y"=530272.8380035125}, {"X"=175379.17377965036, "Y"=530272.8933911546}, {"X"=175379.21499514012, "Y"=530272.9488104766}, {"X"=175379.25621501883, "Y"=530273.0033163701}, {"X"=175379.2960237182, "Y"=530273.0580761392}, {"X"=175379.33575262167, "Y"=530273.1128117243}, {"X"=175379.3756350914, "Y"=530273.1676578454}, {"X"=175379.41577269154, "Y"=530273.222211321}, {"X"=175379.45561149748, "Y"=530273.2769687815}, {"X"=175379.49584439732, "Y"=530273.3307983498}, {"X"=175379.53572220702, "Y"=530273.3837610537}, {"X"=175379.57504594701, "Y"=530273.4362681268}, {"X"=175379.61395791481, "Y"=530273.4879118324}, {"X"=175379.653285014, "Y"=530273.5397552007}, {"X"=175379.69188306064, "Y"=530273.5924819438}, {"X"=175379.73056062285, "Y"=530273.6460419565}, {"X"=175379.76959291293, "Y"=530273.6994422176}, {"X"=175379.8094673134, "Y"=530273.7524515456}, {"X"=175379.8491786922, "Y"=530273.8051483744}, {"X"=175379.88896082636, "Y"=530273.8581091418}, {"X"=175379.9291784505, "Y"=530273.9121673888}, {"X"=175379.97054167185, "Y"=530273.9666229206}, {"X"=175380.01182172928, "Y"=530274.0226169619}, {"X"=175380.05318232844, "Y"=530274.079491995}, {"X"=175380.09513207295, "Y"=530274.1364019196}, {"X"=175380.13819652947, "Y"=530274.1925460887}, {"X"=175380.18149366078, "Y"=530274.2491956674}, {"X"=175380.2250484434, "Y"=530274.3055070925}, {"X"=175380.26838144008, "Y"=530274.3623041774}, {"X"=175380.31188147655, "Y"=530274.4186745853}, {"X"=175380.3549409229, "Y"=530274.4749230964}, {"X"=175380.3972649774, "Y"=530274.5308053015}, {"X"=175380.43836973322, "Y"=530274.5862271729}, {"X"=175380.47931384272, "Y"=530274.6406384385}, {"X"=175380.5204471117, "Y"=530274.694614081}, {"X"=175380.56209510507, "Y"=530274.748920056}, {"X"=175380.60371871642, "Y"=530274.8033692753}, {"X"=175380.6451534636, "Y"=530274.8583540027}, {"X"=175380.68621689494, "Y"=530274.91297912}, {"X"=175380.72710987853, "Y"=530274.9677778766}, {"X"=175380.76810750342, "Y"=530275.0226162815}, {"X"=175380.80994694738, "Y"=530275.0778672938}, {"X"=175380.85239067252, "Y"=530275.1334805603}, {"X"=175380.89503053552, "Y"=530275.1901265308}, {"X"=175380.9377349384, "Y"=530275.246731244}, {"X"=175380.9805978658, "Y"=530275.3030247326}, {"X"=175381.0230490275, "Y"=530275.3587578452}, {"X"=175381.06513342983, "Y"=530275.4135730725}, {"X"=175381.10631238978, "Y"=530275.4686295863}, {"X"=175381.14743795973, "Y"=530275.5233022464}, {"X"=175381.18891169218, "Y"=530275.5779927488}, {"X"=175381.23041948982, "Y"=530275.6325200024}, {"X"=175381.27197850702, "Y"=530275.6875975949}, {"X"=175381.3141971989, "Y"=530275.7425955562}, {"X"=175381.35612077633, "Y"=530275.7987464201}, {"X"=175381.39866254883, "Y"=530275.8545702754}, {"X"=175381.44144096706, "Y"=530275.9110449206}, {"X"=175381.48396489912, "Y"=530275.9674281975}, {"X"=175381.52566846483, "Y"=530276.0237661658}, {"X"=175381.56639495818, "Y"=530276.0791813901}, {"X"=175381.60614632058, "Y"=530276.1337315745}, {"X"=175381.64565829624, "Y"=530276.1873035681}, {"X"=175381.68537671026, "Y"=530276.2408927118}, {"X"=175381.72567720927, "Y"=530276.2954279619}, {"X"=175381.76592636586, "Y"=530276.3505771153}, {"X"=175381.8065536897, "Y"=530276.4066074943}, {"X"=175381.84723761232, "Y"=530276.4623069686}, {"X"=175381.8881185681, "Y"=530276.5175375018}, {"X"=175381.92892906343, "Y"=530276.5717005575}, {"X"=175381.96981449414, "Y"=530276.6260454104}, {"X"=175382.0109063195, "Y"=530276.6806926475}, {"X"=175382.05228986236, "Y"=530276.7360426767}, {"X"=175382.09401500106, "Y"=530276.7918878068}, {"X"=175382.13590830663, "Y"=530276.848290703}, {"X"=175382.17683812688, "Y"=530276.9053778878}, {"X"=175382.21736197197, "Y"=530276.9623663815}, {"X"=175382.25794670594, "Y"=530277.0195777777}, {"X"=175382.299110183, "Y"=530277.076300242}, {"X"=175382.3405598369, "Y"=530277.1330462806}, {"X"=175382.3816216344, "Y"=530277.1898323065}, {"X"=175382.42177914153, "Y"=530277.246647631}, {"X"=175382.4623105062, "Y"=530277.3016794228}, {"X"=175382.50294386526, "Y"=530277.3558518823}, {"X"=175382.54306338512, "Y"=530277.4093932352}, {"X"=175382.58212770906, "Y"=530277.4634571102}, {"X"=175382.62030600384, "Y"=530277.5183382287}, {"X"=175382.65887284116, "Y"=530277.5734135413}, {"X"=175382.69841257622, "Y"=530277.6285958623}, {"X"=175382.73787164403, "Y"=530277.6837573361}, {"X"=175382.77683788392, "Y"=530277.7388048348}, {"X"=175382.81560297194, "Y"=530277.7935244082}, {"X"=175382.85500985917, "Y"=530277.8484130106}, {"X"=175382.89468581765, "Y"=530277.9029312362}, {"X"=175382.93342362894, "Y"=530277.9580138144}, {"X"=175382.97016422707, "Y"=530278.0137726283}, {"X"=175383.00719641265, "Y"=530278.0689867527}, {"X"=175383.04524049233, "Y"=530278.1234110076}, {"X"=175383.08446525745, "Y"=530278.177516587}, {"X"=175383.12400785997, "Y"=530278.2324713808}, {"X"=175383.16341338272, "Y"=530278.2884021463}, {"X"=175383.20321088587, "Y"=530278.3450931216}, {"X"=175383.24388467334, "Y"=530278.4018691962}, {"X"=175383.28416762798, "Y"=530278.46038113}, {"X"=175383.32348511857, "Y"=530278.5201078751}, {"X"=175383.36322165257, "Y"=530278.5798589126}, {"X"=175383.40385465274, "Y"=530278.6390279633}, {"X"=175383.44465535972, "Y"=530278.6989001713}, {"X"=175383.4862341692, "Y"=530278.75830284}, {"X"=175383.52822093136, "Y"=530278.8175722327}, {"X"=175383.56995807827, "Y"=530278.8769011825}, {"X"=175383.61148408483, "Y"=530278.9361197695}, {"X"=175383.65323525056, "Y"=530278.9944953114}, {"X"=175383.69421530858, "Y"=530279.0530074155}, {"X"=175383.7350554744, "Y"=530279.111541019}, {"X"=175383.77542995836, "Y"=530279.1704555652}, {"X"=175383.8157298488, "Y"=530279.2293070713}, {"X"=175383.8559401721, "Y"=530279.2881233235}, {"X"=175383.89695070562, "Y"=530279.3461569902}, {"X"=175383.93826252603, "Y"=530279.4039311717}, {"X"=175383.97949878522, "Y"=530279.4619153388}, {"X"=175384.02036026714, "Y"=530279.5201691986}, {"X"=175384.06054778706, "Y"=530279.5790632094}, {"X"=175384.10039149693, "Y"=530279.6382146104}, {"X"=175384.14101006766, "Y"=530279.6973004678}, {"X"=175384.1822571442, "Y"=530279.7559505224}, {"X"=175384.22384488, "Y"=530279.8141767163}, {"X"=175384.26575571846, "Y"=530279.8720312649}, {"X"=175384.30757643149, "Y"=530279.9302634323}, {"X"=175384.34938070193, "Y"=530279.988026178}, {"X"=175384.39056756336, "Y"=530280.0457807535}, {"X"=175384.4300316461, "Y"=530280.1038567104}, {"X"=175384.46858665868, "Y"=530280.1612416819}, {"X"=175384.5074643027, "Y"=530280.2174947566}, {"X"=175384.54749630456, "Y"=530280.2726090478}, {"X"=175384.586673461, "Y"=530280.3276992185}, {"X"=175384.62548891825, "Y"=530280.3817849228}, {"X"=175384.66357065516, "Y"=530280.4351669155}, {"X"=175384.70142916602, "Y"=530280.4873442599}, {"X"=175384.7383800607, "Y"=530280.538421075}, {"X"=175384.77384348479, "Y"=530280.5882103939}, {"X"=175384.80759560052, "Y"=530280.6358982379}, {"X"=175384.8404099675, "Y"=530280.6812770056}, {"X"=175384.87250879448, "Y"=530280.7243071992}, {"X"=175384.90436964578, "Y"=530280.7647299246}, {"X"=175384.93436790677, "Y"=530280.80311488}, {"X"=175384.9616378935, "Y"=530280.8381638632}, {"X"=175384.9850736076, "Y"=530280.8648757731}, {"X"=175385.00324402758, "Y"=530280.8833868961}, {"X"=175385.0150459357, "Y"=530280.8944529634}, {"X"=175385.02297698648, "Y"=530280.9010033109}, {"X"=175385.02939790592, "Y"=530280.9042851299}, {"X"=175385.03577591613, "Y"=530280.9056281495}, {"X"=175385.04157625238, "Y"=530280.9066199363}, {"X"=175385.04734175224, "Y"=530280.9069115034}, {"X"=175385.0522705122, "Y"=530280.9070113084}, {"X"=175385.05647557072, "Y"=530280.9068024849}, {"X"=175385.06001046783, "Y"=530280.9061183934}, {"X"=175385.06346903727, "Y"=530280.9044811573}, {"X"=175385.06641534183, "Y"=530280.9021439983}, {"X"=175385.06904727407, "Y"=530280.8992328586}, {"X"=175385.0711258982, "Y"=530280.896123573}, {"X"=175385.0733705323, "Y"=530280.8925376674}, {"X"=175385.0755269345, "Y"=530280.8887688976}, {"X"=175385.07764847262, "Y"=530280.8848914615}, {"X"=175385.07942518912, "Y"=530280.8812292453}, {"X"=175385.08167830165, "Y"=530280.8775145715}, {"X"=175385.08414133126, "Y"=530280.8740967229}, {"X"=175385.08691378706, "Y"=530280.871078623}]}, ...(6 in all)]
  out "back ground":bool
  # "Waypoint Simulation"
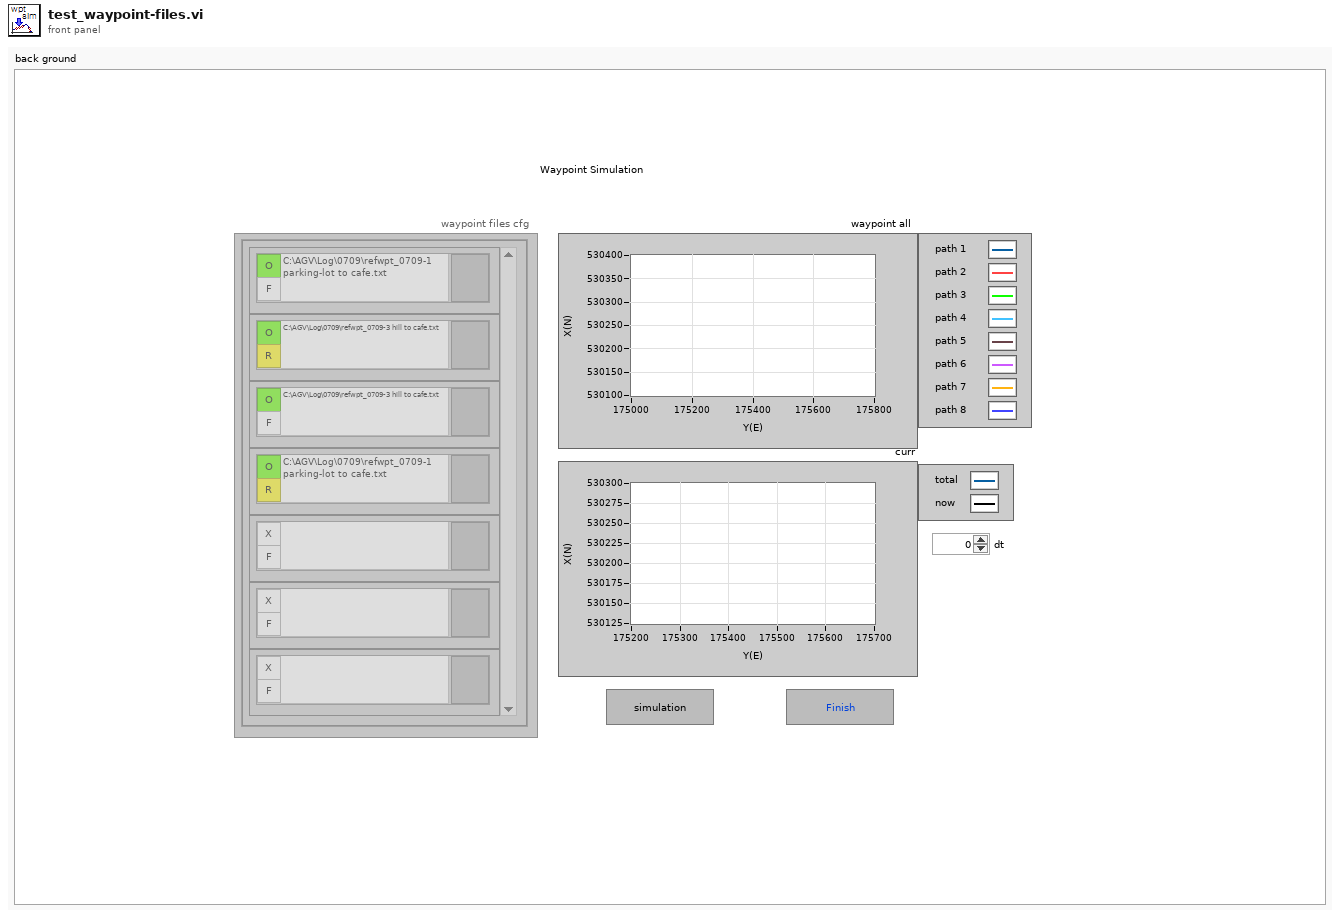
[diagram p1: front panel]
types:
  T1 = cluster{"Waypoint array":cluster{"sel":bool, "inv":bool, "path":path}[]}
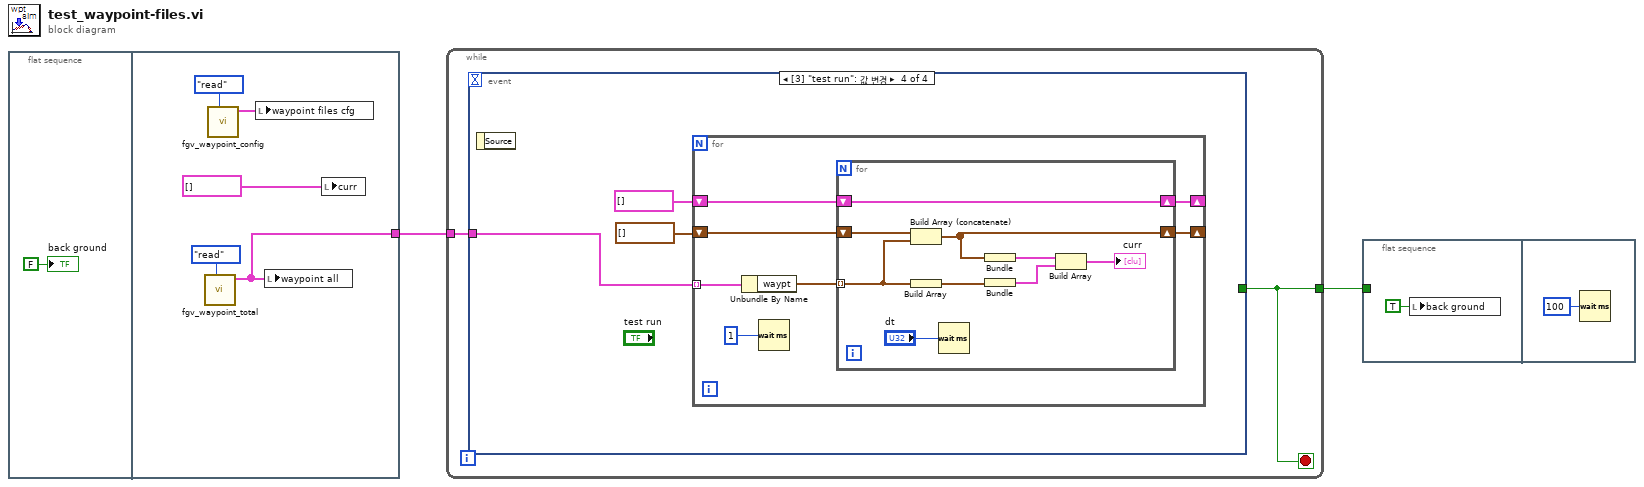
[diagram p0: block diagram]
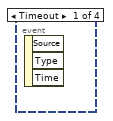
[diagram p2: hidden frame]
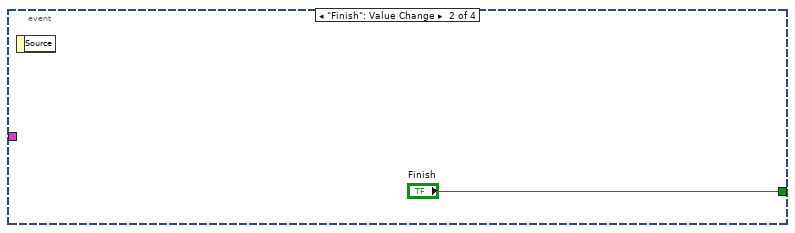
[diagram p3: hidden frame]
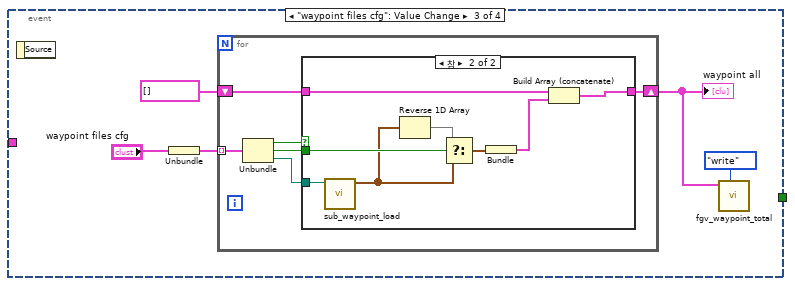
[diagram p4: hidden frame]
diagram:
  n1 = flat-sequence {
    tunnel: [w4] -> w1
    frame #0 {
      "back ground" <- FALSE ("back ground")
    }
    frame #1 {
      n2 = call "fgv_waypoint_total.vi"("cmd"=enum16{"write", "read"}."read") -> ("waypoint total out"=w4:cluster{"waypt":cluster{"X":dbl, "Y":dbl}[]}[])  [unwired: 10 in]
      n3 = call "fgv_waypoint_config.vi"("cmd"=enum16{"read", "write"}."read") -> ("waypoint files cfg out"=w6:T1)  [unwired: 10 in]
      n4 = local write "waypoint files cfg"(w6) -> ()
      n5 = local write "waypoint all"(w4) -> ()
      n6 = local write "curr"(cluster{cluster{"X":dbl, "Y":dbl}[]}[] [] ("curr")) -> ()
    }
  }
  n7 = while {
    tunnel: [w10] -> w2
    tunnel: w1 -> [w9]
    stop <- w10 stop-if-true
    n8 = event shown="[3] \"test run\": 값 변경" {
      selector: _ -> [_ _ _ _]
      dyn-events: _ -> [_ _ _ _]
      timeout: _ -> [_ _ _ _]
      tunnel: [_ "Finish" _ _] -> w10
      tunnel: w9 -> [_ _ _ w32]
      event Timeout {
        n9 = event-data() -> ()  [unwired: 1 in, 3 out]
      }
      event "Finish": Value Change {
        n10 = event-data() -> ()  [unwired: 1 in, 1 out]
      }
      event "waypoint files cfg": Value Change {
        n11 = event-data() -> ()  [unwired: 1 in, 1 out]
        n12 = Unbundle("waypoint files cfg") -> ("Waypoint array"=w16:cluster{"sel":bool, "inv":bool, "path":path}[])
        n13 = for {
          tunnel: w16 -> [w20] mode=indexing
          shift-right: [w21] -> w13
          shift-left: cluster{"XY 그래프":cluster{"X":dbl, "Y":dbl}[]}[] [] -> [w22]
          n14 = Unbundle(w20) -> ("sel"=w19:bool, "inv"=w17:bool, "path"=w18:path)
          n15 = case shown="참" w19 {
            tunnel: w22 -> [w23 w31]
            tunnel: [w23 w30] -> w21
            tunnel: w18 -> [_ w28]
            tunnel: w17 -> [_ w27]
            frame False {
            }
            frame True {
              n16 = call "sub_waypoint_load.vi"("path"=w28) -> ("XY 그래프"=w24:cluster{"X":dbl, "Y":dbl}[])  [unwired: 10 in]
              n17 = Reverse 1D Array(array=w24) -> (reversed array=w25:cluster{"X":dbl, "Y":dbl}[])
              n18 = Select(t=w25, s=w27, f=w24) -> (s? t:f=w26:cluster{"X":dbl, "Y":dbl}[])
              n19 = Bundle("XY 그래프"=w26) -> (w29:cluster{"XY 그래프":cluster{"X":dbl, "Y":dbl}[]})  [unwired: 1 in]
              n20 = Build Array (concatenate)(w31, w29) -> (w30:cluster{"XY 그래프":cluster{"X":dbl, "Y":dbl}[]}[])
            }
          }
        }
        "waypoint all" <- w13
        n21 = call "fgv_waypoint_total.vi"("cmd"=enum16{"write", "read"}."write", "waypoint total in"=w13) -> ()  [unwired: 9 in, 1 out]
      }
      event "test run": Value Change {
        n22 = event-data() -> ()  [unwired: 1 in, 1 out]
        n23 = for {
          tunnel: w32 -> [w41] mode=indexing
          shift-right: [w38] -> _
          shift-left: cluster{"XY 그래프":cluster{"X":dbl, "Y":dbl}[]}[] [] ("waypoint all graph") -> [w39]
          shift-right: [w36] -> _
          shift-left: cluster{"X":dbl, "Y":dbl}[] [] ("XY 그래프") -> [w37]
          n24 = Unbundle By Name(w41) -> ("waypt"=w40:cluster{"X":dbl, "Y":dbl}[])
          n25 = Wait (ms)(milliseconds to wait=u32 1 ("dt")) -> ()  [unwired: 1 out]
          n26 = for {
            tunnel: w40 -> [w44] mode=indexing
            shift-right: [w48] -> w38
            shift-left: w39 -> [w48]
            shift-right: [w45] -> w36
            shift-left: w37 -> [w49]
            n27 = Build Array (concatenate)(w49, w44) -> (w45:cluster{"X":dbl, "Y":dbl}[])
            n28 = Build Array(w44) -> (w43:cluster{"X":dbl, "Y":dbl}[])
            n29 = Wait (ms)(milliseconds to wait="dt") -> ()  [unwired: 1 out]
            n30 = Bundle(w45) -> (w47:cluster{cluster{"X":dbl, "Y":dbl}[]})  [unwired: 1 in]
            n31 = Bundle(w43) -> (w42:cluster{cluster{"X":dbl, "Y":dbl}[]})  [unwired: 1 in]
            n32 = Build Array(w47, w42) -> (→"curr":cluster{cluster{"X":dbl, "Y":dbl}[]}[])
          }
        }
      }
    }
  }
  n33 = flat-sequence {
    tunnel: w2 -> [_]
    frame #0 {
      n34 = local write "back ground"(TRUE ("back ground")) -> ()
    }
    frame #1 {
      n35 = Wait (ms)(milliseconds to wait=u32 100 ("대기 시간 (ms)")) -> ()  [unwired: 1 out]
    }
  }
